vi "Text control 2 v7.2.vi"() -> ()   [LabVIEW 2019]
panel:
  in  "Tab Control":enum32{"Main", "Other parameters"}(tab)
  out "Vdg vs time (Bias Stress)":cluster{"Y data in":dbl[], "X data in":dbl[]}[](graph)
  out "Vp vs Vg (FPP)":cluster{"Y data in":dbl[], "X data in":dbl[]}[](graph)
  out "Vp2":dbl format="%.2e"
  out "Vp1":dbl format="%.2e"
  out "Vp vs time (FPP Bias Stress)":cluster{"Y data in":dbl[], "X data in":dbl[]}[](graph)
  in  "Plot sample extrema vs time":bool
  out "Line running":i32
  out "Total lines":i32
  out "Path":path=path "C:/users/rlp38/09Apr2009LTtesting/test2.txt"
  out "I vs Vg":cluster{"Y data in":dbl[], "X data in":dbl[]}[](graph)
  out "Is max":dbl format="%.2e"
  out "Id max":dbl format="%.2e"
  out "Ig max":dbl format="%.2e"
  out "Imax vs time":cluster{"Y data in":dbl[], "X data in":dbl[]}[](graph)
  out "Imin vs time":cluster{"Y data in":dbl[], "X data in":dbl[]}[](graph)
  out "I vs Vd":cluster{"Y data in":dbl[], "X data in":dbl[]}[](graph)
  in  "Script":string="#pulsedstressV d 0.03 20 0 0.5 0.0827 5\n#\n#itime m\n#gaterangemode a\n#drainrangemode a\n#pulsed on 0.05 0 0.02\n#transfer d -10 40 1 5 40 35\n#transfer d -10 40 1 5 40 35\n#transfer d -10 40 1 5 40 35\n#output d 0 40 20 0 40 1\n#\n#\n#sample 1 0.008 221 6 0.003\n#samplei 400e-6 200 6 0.002 0.1\n#vsu2pulse -10 4\n#\n#stressV 0.016 0.03 2e-4 0.1e-3 11\n#stressI 220e-7 0.08 15\n#transfer s -1 1 0.5 -0.005 0.005 0.005\n#output s 0 0 0 -0.008 0.008 0.002"
  out "Command running:":string
  out "Serial port data":string
  out "Elapsed Time":dbl caption="Elapsed Time (s)"
  in  "Time Units":u16(ring)=1 items=["Seconds", "Minutes", "Hours"]
  in  "Time Offset":dbl caption="Set Start Time (s)"
  in  "Reset":bool
  in  "Auto Reset":bool
  in  "integration time":u32(slide) max=2 step=1 scale=0.0..2.0
  out "Is on":dbl format="%.2e"
  out "Id on":dbl format="%.2e"
  out "Ig on":dbl format="%.2e"
  out "Ion vs time":cluster{"Y data in":dbl[], "X data in":dbl[]}[](graph)
  out "Ioff vs time":cluster{"Y data in":dbl[], "X data in":dbl[]}[](graph)
  out "Ig min":dbl format="%.2e"
  out "Id min":dbl format="%.2e"
  out "Is min":dbl format="%.2e"
  out "Is off":dbl format="%.2e"
  out "Id off":dbl format="%.2e"
  out "Ig off":dbl format="%.2e"
  in  "Integration time (long)":dbl=0.32 min=0.04 max=2.0 step=0.02 format="%.2f"
  in  "Integration time (short)":dbl=0.0019 min=8e-05 max=0.0019 step=8e-05 format="%^.0e"
  in  "Drain: Compliance":dbl=0.001 format="%.8f"
  in  "Gate: Compliance":dbl=0.001 format="%.8f"
  in  "Interrupt scan":bool
  in  "Interrupt program":bool
  in  "Plot output curve extrema vs time":bool
  in  "Plot transfer curve extrema vs time":bool
  out "I vs time (Bias Stress)":cluster{"Y data in":dbl[], "X data in":dbl[]}[](graph)
  in  "Sample I - Probe 4 (Disabled)":u32(ring)=3 items=["SMU1  ", "SMU2  ", "SMU3  ", "SMU4  ", "SMU5  ", "SMU6  ", "VSU1  ", "VSU2  "]
  in  "Sample I - Source/Common":u32(ring) items=["SMU1  ", "SMU2  ", "SMU3  ", "SMU4  ", "SMU5  ", "SMU6  ", "VSU1  ", "VSU2  "]
  in  "Sample I - Probe 3 (Disabled)":u32(ring)=2 items=["SMU1  ", "SMU2  ", "SMU3  ", "SMU4  ", "SMU5  ", "SMU6  ", "VSU1  ", "VSU2  "]
  in  "Sample I - Drain/Gate":u32(ring)=1 items=["SMU1  ", "SMU2  ", "SMU3  ", "SMU4  ", "SMU5  ", "SMU6  ", "VSU1  ", "VSU2  "]
  in  "Sample - Probe 4":u32(ring)=3 items=["SMU1  ", "SMU2  ", "SMU3  ", "SMU4  ", "SMU5  ", "SMU6  ", "VSU1  ", "VSU2  "]
  in  "Sample - Source/Common":u32(ring) items=["SMU1  ", "SMU2  ", "SMU3  ", "SMU4  ", "SMU5  ", "SMU6  ", "VSU1  ", "VSU2  "]
  in  "Sample - Gate":u32(ring)=2 items=["SMU1  ", "SMU2  ", "SMU3  ", "SMU4  ", "SMU5  ", "SMU6  ", "VSU1  ", "VSU2  "]
  in  "Sample - Drain":u32(ring)=1 items=["SMU1  ", "SMU2  ", "SMU3  ", "SMU4  ", "SMU5  ", "SMU6  ", "VSU1  ", "VSU2  "]
  in  "Gate Range\nmode":u16(ring) items=["Auto", "Limited", "Fixed"]
  in  "Gate Range":u8(slide)=3 max=11 scale=0.0..11.0
  in  "Source/Drain\nRange mode":u16(ring) items=["Auto", "Limited", "Fixed"]
  in  "Source/Drain Range":u8(slide)=3 max=11 scale=0.0..11.0
  in  "Panel Controls":T1={"Emergency Stop"=refnum, "TransGraph Max"=1e-05, "Text/Graph (text=false)"=TRUE} {"TransGraph Max" format="%.2e"}
  in  "Panel Controls 2":T2={"Emergency Stop"=refnum, "TransGraph Max"=1e-05, "Text/Graph (text=false)"=TRUE, "TransGraph Min"=1e-11} {"TransGraph Min" format="%.2e"; "TransGraph Max" format="%.2e"}
  out "error out":errorcluster
  in  "Delay before read (ms)":u32=1000
  in  "byte count":u32=64
  in  "Serial End Mode for Reads":u16(ring)=2 items=["None", "LastBit", "TermChar"]
  in  "Timeout (ms)":u32=10000
  in  "Enable Termination\nChar (T)":bool=TRUE
  in  "Termination char\n(0xA = '\\n' = LF)\n(0xD = '\\r' = CR)":u8=13 format="%.0x"
  in  "flow control":u16(ring) items=["None"=0, "XON/XOFF"=1, "RTS/CTS"=2, "DTR/DSR"=4]
  in  "stop bits":u16(ring)=10 items=["1.0"=10, "1.5"=15, "2.0"=20]
  in  "parity":u16(ring) items=["None", "Odd", "Even", "Mark", "Space"]
  in  "data bits":u16=8 min=5 max=8 step=1
  in  "VISA resource name":refnum<visa-resource-name>="COM6"
  in  "baud rate":u32=9600
  out "Timings Indicator":T3
  in  "Timings (overwritten by the Front Panel)":T4={"integration time"=0, "Short/Long integration time"=0.00064, "hold time (sec)"=0.0, "delay time (sec)"=0.0, "Step Time (0 disables)"=0.0, "sweep method"=0, "Pulse period"=0.005, "Base voltage"=0.0, "Pulse width"=0.0005} {"Pulse width" min=0.0005 max=0.1 step=0.0001 format="%.4f"; "Base voltage" format="%^.4e"; "Pulse period" min=0.005 max=1.0 step=0.0001 format="%.4f"; "sweep method" items=["Continuous", "Pulsed"]; "Step Time (0 disables)" format="%.2f"; "delay time (sec)" format="%.4f"; "hold time (sec)" format="%.4f"; "Short/Long integration time" format="%^.0e"; "integration time" scale=0.0..2.0}
  in  "Probe 4":cluster{"on/off":bool, "Voltage":dbl} {"Voltage" min=-100.0 max=100.0 format="%.2f"}
  in  "Full Reset":bool
  in  "Standby":T5
  out "Probe 4 Indicator":cluster{"on/off":bool, "Voltage":dbl} {"Voltage" min=-100.0 max=100.0 format="%.2f"}
  in  "Transfer/Output - Drain":u32(ring)=1 items=["SMU1  ", "SMU2  ", "SMU3  ", "SMU4  ", "SMU5  ", "SMU6  ", "VSU1  ", "VSU2  "]
  in  "Transfer/Output - Gate":u32(ring)=2 items=["SMU1  ", "SMU2  ", "SMU3  ", "SMU4  ", "SMU5  ", "SMU6  ", "VSU1  ", "VSU2  "]
  in  "Transfer/Output - Source/Common":u32(ring) items=["SMU1  ", "SMU2  ", "SMU3  ", "SMU4  ", "SMU5  ", "SMU6  ", "VSU1  ", "VSU2  "]
  in  "Transfer/Output - Probe 4":u32(ring)=3 items=["SMU1  ", "SMU2  ", "SMU3  ", "SMU4  ", "SMU5  ", "SMU6  ", "VSU1  ", "VSU2  "]
  in  "Pulsed Stress V - Probe 4":u32(ring)=3 items=["SMU1  ", "SMU2  ", "SMU3  ", "SMU4  ", "SMU5  ", "SMU6  ", "VSU1  ", "VSU2  "]
  in  "Pulsed Stress V - Vextra":u32(ring)=6 items=["SMU1  ", "SMU2  ", "SMU3  ", "SMU4  ", "SMU5  ", "SMU6  ", "VSU1  ", "VSU2  "]
  in  "Pulsed Stress V - Drain":u32(ring)=1 items=["SMU1  ", "SMU2  ", "SMU3  ", "SMU4  ", "SMU5  ", "SMU6  ", "VSU1  ", "VSU2  "]
  in  "Pulsed Stress V - Source/Common":u32(ring) items=["SMU1  ", "SMU2  ", "SMU3  ", "SMU4  ", "SMU5  ", "SMU6  ", "VSU1  ", "VSU2  "]
  in  "Pulsed Stress V - Gate":u32(ring)=2 items=["SMU1  ", "SMU2  ", "SMU3  ", "SMU4  ", "SMU5  ", "SMU6  ", "VSU1  ", "VSU2  "]
  in  "FPP - Drain":u32(ring)=1 items=["SMU1  ", "SMU2  ", "SMU3  ", "SMU4  ", "SMU5  ", "SMU6  ", "VSU1  ", "VSU2  "]
  in  "FPP - Gate":u32(ring)=2 items=["SMU1  ", "SMU2  ", "SMU3  ", "SMU4  ", "SMU5  ", "SMU6  ", "VSU1  ", "VSU2  "]
  in  "FPP - Probe 1":u32(ring) items=["SMU1  ", "SMU2  ", "SMU3  ", "SMU4  ", "SMU5  ", "SMU6  ", "VSU1  ", "VSU2  "]
  in  "FPP - Probe 2":u32(ring)=3 items=["SMU1  ", "SMU2  ", "SMU3  ", "SMU4  ", "SMU5  ", "SMU6  ", "VSU1  ", "VSU2  "]
  in  "FPP - Source":u32(ring)=6 items=["SMU1  ", "SMU2  ", "SMU3  ", "SMU4  ", "SMU5  ", "SMU6  ", "VSU1  ", "VSU2  "]
  in  "Stress V - Drain":u32(ring)=1 items=["SMU1  ", "SMU2  ", "SMU3  ", "SMU4  ", "SMU5  ", "SMU6  ", "VSU1  ", "VSU2  "]
  in  "Stress V - Gate":u32(ring)=2 items=["SMU1  ", "SMU2  ", "SMU3  ", "SMU4  ", "SMU5  ", "SMU6  ", "VSU1  ", "VSU2  "]
  in  "Stress V - Source/Common":u32(ring) items=["SMU1  ", "SMU2  ", "SMU3  ", "SMU4  ", "SMU5  ", "SMU6  ", "VSU1  ", "VSU2  "]
  in  "Stress I - Drain/Gate":u32(ring)=1 items=["SMU1  ", "SMU2  ", "SMU3  ", "SMU4  ", "SMU5  ", "SMU6  ", "VSU1  ", "VSU2  "]
  in  "Stress I - Source/Common":u32(ring) items=["SMU1  ", "SMU2  ", "SMU3  ", "SMU4  ", "SMU5  ", "SMU6  ", "VSU1  ", "VSU2  "]
  in  "VSU2 Stress - Source/Common":u32(ring) items=["SMU1  ", "SMU2  ", "SMU3  ", "SMU4  ", "SMU5  ", "SMU6  ", "VSU1  "]
  in  "VISA resource name in":refnum<visa-resource-name>="GPIB0::14::INSTR"
  in  "Gate":T6={"Gate Start"=0.0, "Gate Stop"=2.0, "Gate Step (linear only)"=1.0, "Gate Compliance"=0.0001, "Gate PComp"=0.0, "Range mode"=0, "Range"=6} {"Range" max=11 scale=0.0..11.0; "Range mode" items=["Auto", "Limited", "Fixed"]; "Gate PComp" format="%^.2e"; "Gate Compliance" format="%^.2e"; "Gate Step (linear only)" format="%^.4e"; "Gate Stop" format="%^.4e"; "Gate Start" format="%^.4e"}
  in  "Drain 2":T7={"Drain Start"=0.0, "Drain Stop"=2.0, "Drain Compliance"=0.0001, "Drain Step"=1.0, "Drain PComp"=0.0, "Range mode"=0, "Range"=6} {"Range" max=11 scale=0.0..11.0; "Range mode" items=["Auto", "Limited", "Fixed"]; "Drain PComp" format="%^.2e"; "Drain Step" format="%^.4e"; "Drain Compliance" format="%^.2e"; "Drain Stop" format="%^.4e"; "Drain Start" format="%^.4e"}
  # "Time"
  # "Syntax:\nitime [s|m|l] time(sec): [s|m|l] determines the integration time setting (small|medium|long) and time sets the value.\nNOTE: The value of the integration time has to be within the range allowed by its category (s|m|l), otherwise, the closest value will be used. (e.g. if the category is set to short but the time value is very long, the actual value used will be the maximum short integration time.\nIntegration times:\n    Short: Default: 640 us. Range: 8E-5 - 1.92E-3 seconds.\n    Medium: Fixed at 1 NPL cycle (0.02 seconds).\n    Long: Default: 16 NPL cycles (0.32 seconds). Range: 2-100 NPL cycles (0.04 seconds - 2 seconds).\ngaterangemode [a|l|f]\ndrainrangemode [a|l|f]\npulsed [on|off] PulsePeriod(sec) PulseBaseVoltage PulseONWidth(sec)\nstandby [on l off]\nwait NumMilliseconds\nwait-min NumMinutes\n# texthere = comment\nProbe4 [ON|OFF] Voltage\ntransfer [s|d] VgStart VgStop VgStep VdStart VdStop VdStep\noutput [s|d] VgStart VgStop VgStep VdStart VdStop VdStep\nsample Vg Vd NumSamples Time(s) SampleInterval(s)\nsamplei Idg NumSamples Time(s) SampleInterval(s) VDGcompliance\n100 samples is approximately 13 seconds with medium integration\n# if in doubt use SampleInterval(s) = 0.004\n    NOTE: When doing bias stress measurements, it is best to set the Time Units to \"Seconds\", as the \"sample\" command has been configured to give the output to seconds.\nstressV VG VD IGcompliance IDcompliance Duration(sec)\nstressI IDG VDGcompliance Duration(sec)\nvsu2pulse Bias Duration(s)\npulsedstressV [s|d] VEstop VgON VgOFF Period(s) PulseONwidth(s) Vd\nsample-fpp Vg Vd NumSamples Time\nresample-fpp Vg Vd\ntransfer-fpp [s|d] VgStart VgStop VgStep VdStart VdStop VdStep\noutput-fpp [s|d] VgStart VgStop VgStep VdStart VdStop VdStep\nserial SerialPortCommand"
  # "1\n2\n3\n4\n5\n6\n7\n8\n9\n10\n11\n12\n13\n14\n15\n16\n17\n18\n19\n20"
  # "SMUs"
  # "Serial port settings"
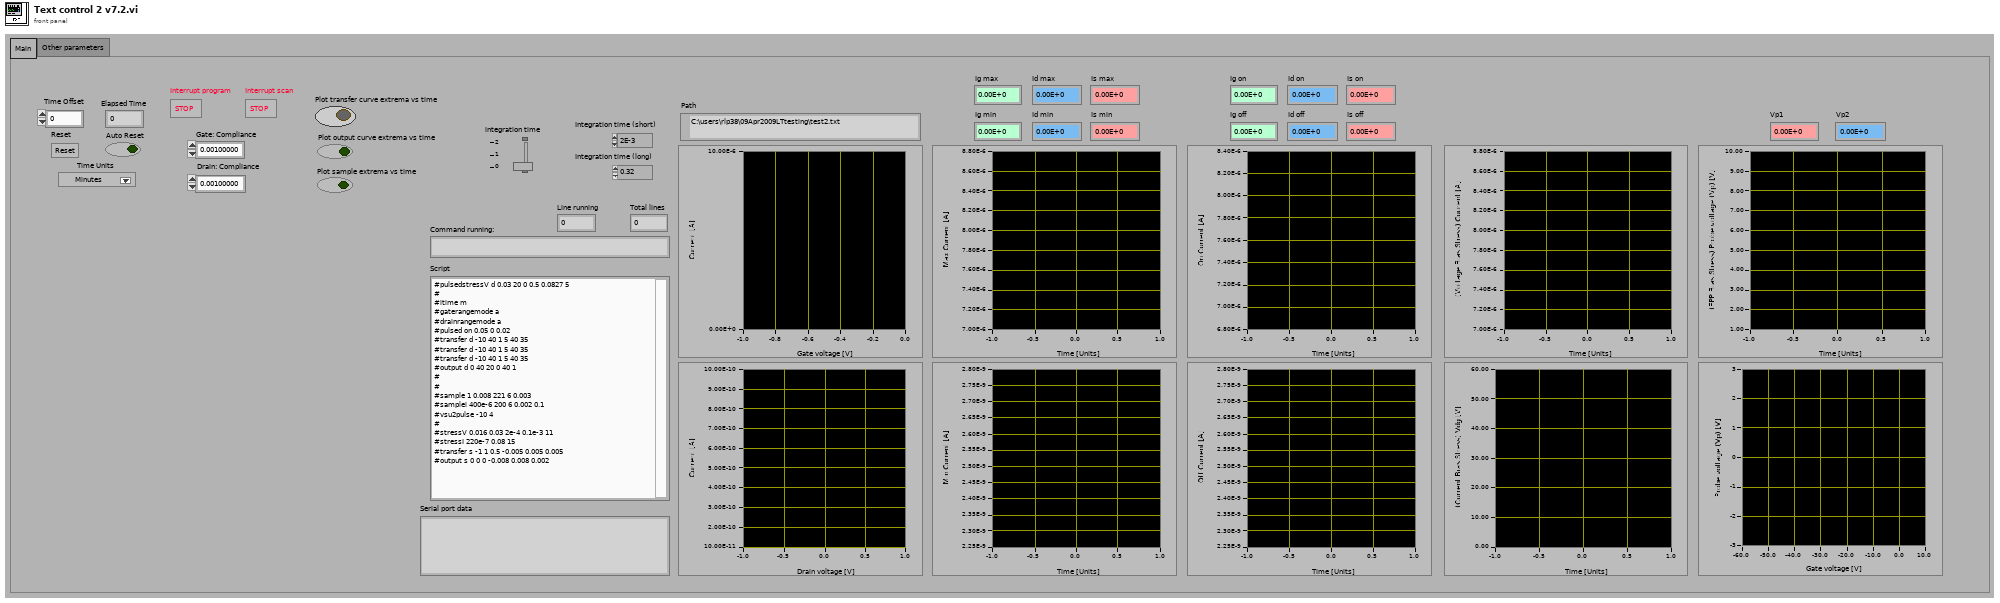
[diagram p1: front panel]
types:
  T1 = cluster{"Emergency Stop":refnum<vi>, "TransGraph Max":dbl, "Text/Graph (text=false)":bool}
  T2 = cluster{"Emergency Stop":refnum<vi>, "TransGraph Max":dbl, "Text/Graph (text=false)":bool, "TransGraph Min":dbl}
  T3 = cluster{"integration time (0:s, 1:m, 2:l)":u32, "Short/Long integration time":dbl, "hold time (sec)":dbl, "delay time (sec)":dbl, "Step Time (0 disables)":dbl, "sweep method":u16, "Pulse period":dbl, "Base voltage":dbl, "Pulse width":dbl}
  T4 = cluster{"integration time":u32, "Short/Long integration time":dbl, "hold time (sec)":dbl, "delay time (sec)":dbl, "Step Time (0 disables)":dbl, "sweep method":u16, "Pulse period":dbl, "Base voltage":dbl, "Pulse width":dbl}
  T5 = cluster{"Gate Standby":bool, "Drain Standby":bool}
  T6 = cluster{"Gate Start":dbl, "Gate Stop":dbl, "Gate Step (linear only)":dbl, "Gate Compliance":dbl, "Gate PComp":dbl, "Range mode":u16, "Range":u8}
  T7 = cluster{"Drain Start":dbl, "Drain Stop":dbl, "Drain Compliance":dbl, "Drain Step":dbl, "Drain PComp":dbl, "Range mode":u16, "Range":u8}
  T8 = enum16{"open", "replace", "create", "open or create", "replace or create", "replace or create with confirmation"}
  T9 = cluster{"V2 Start":dbl, "V2 Step":dbl, "Number of points":i32}
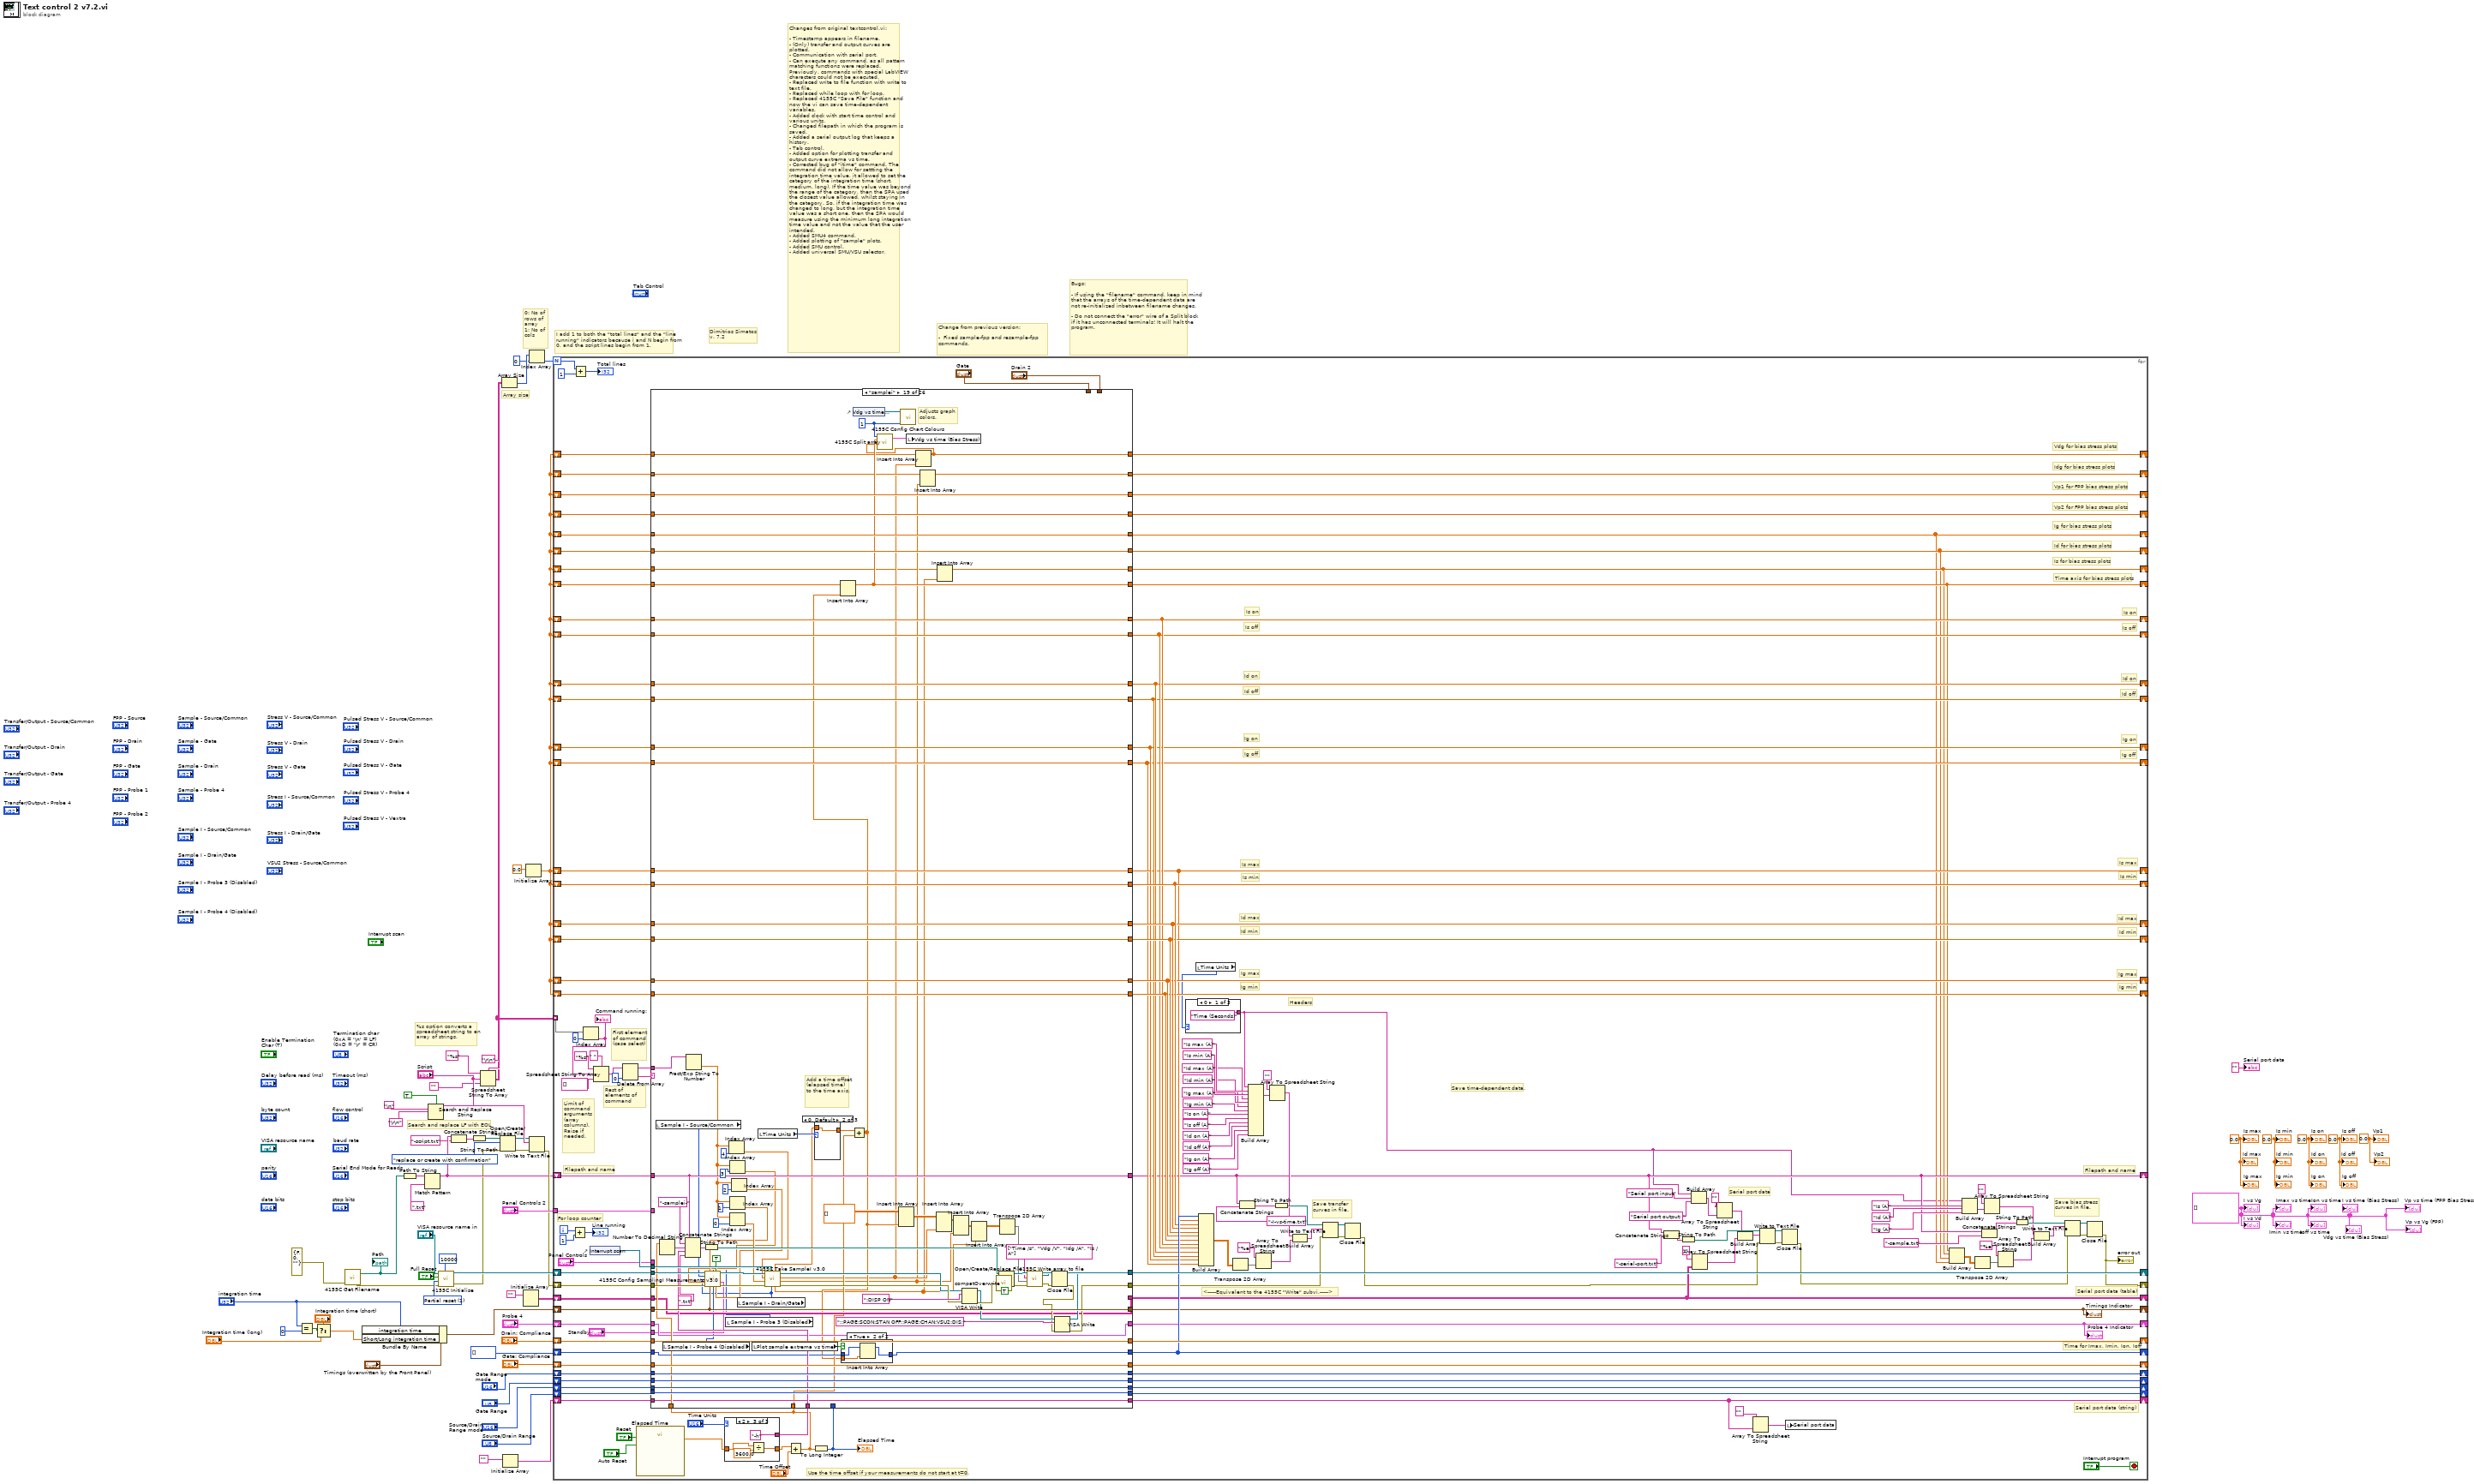
[diagram p0: block diagram]
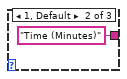
[diagram p2: hidden frame]
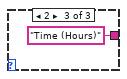
[diagram p3: hidden frame]
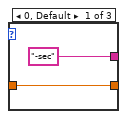
[diagram p4: hidden frame]
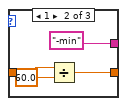
[diagram p5: hidden frame]
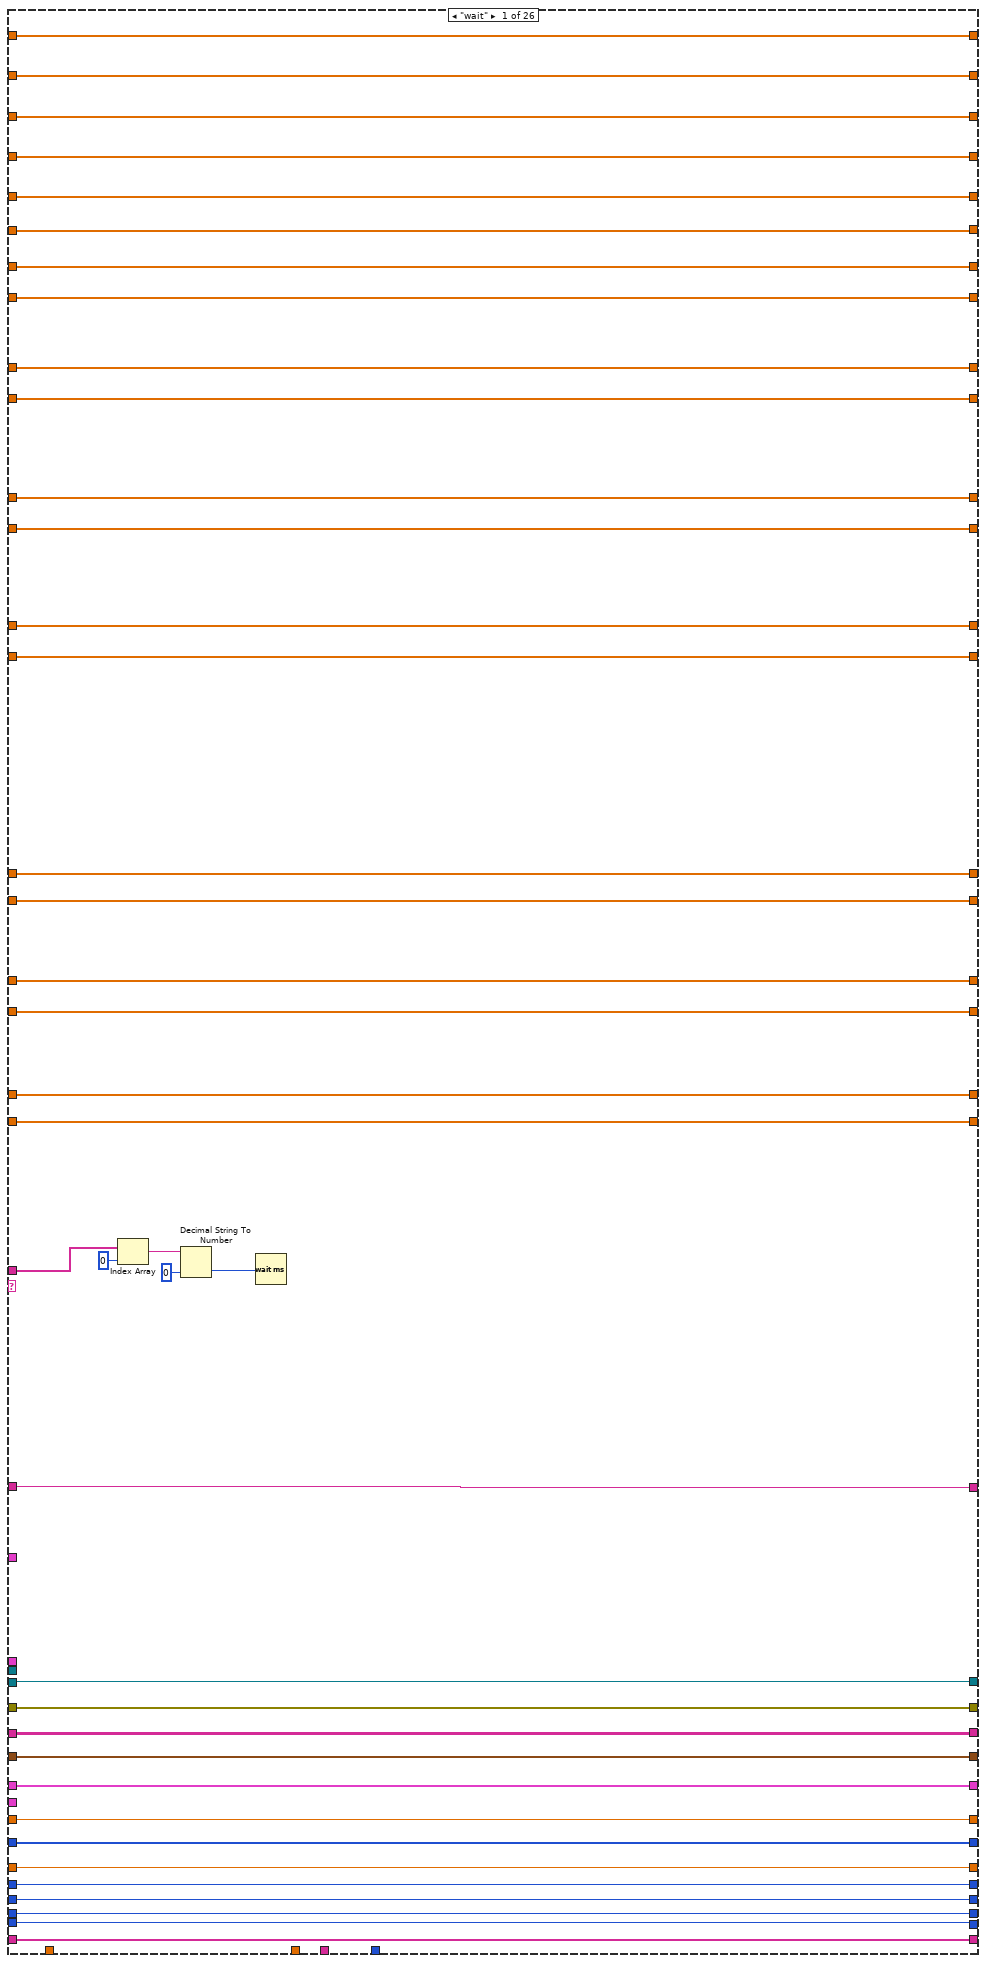
[diagram p6: hidden frame]
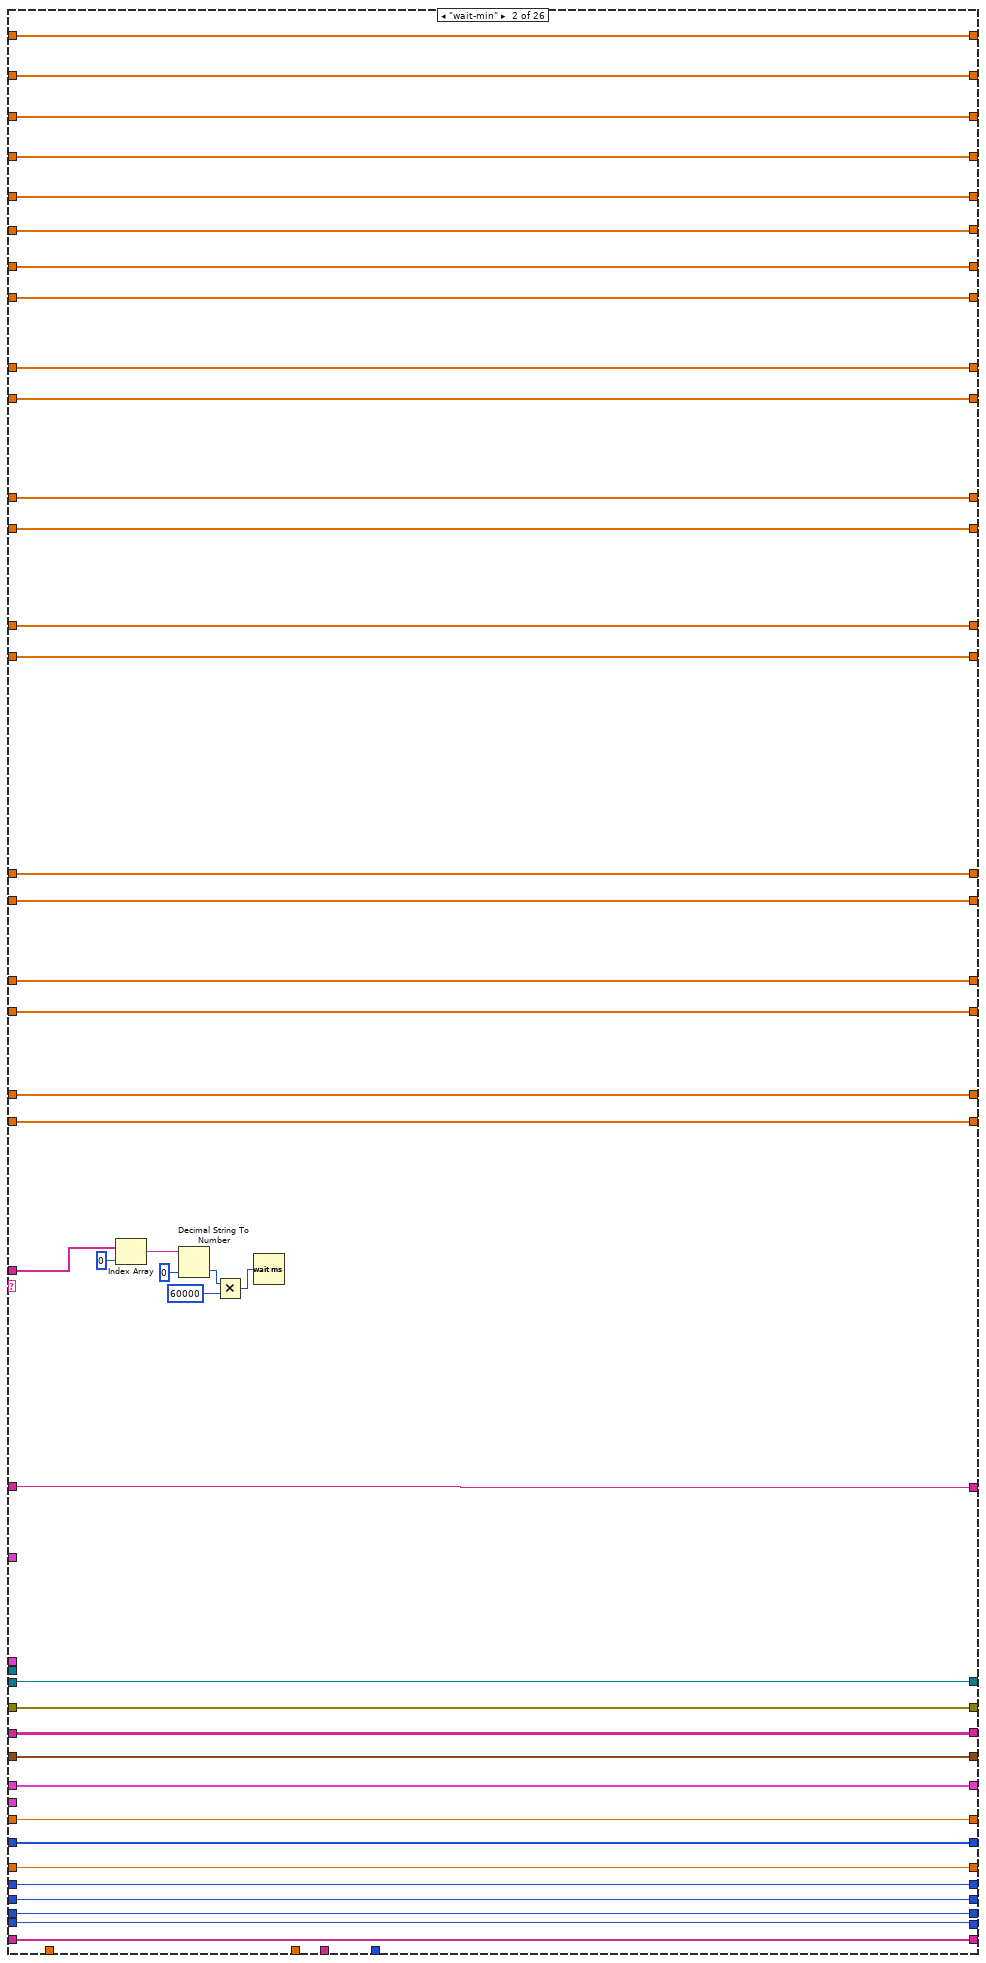
[diagram p7: hidden frame]
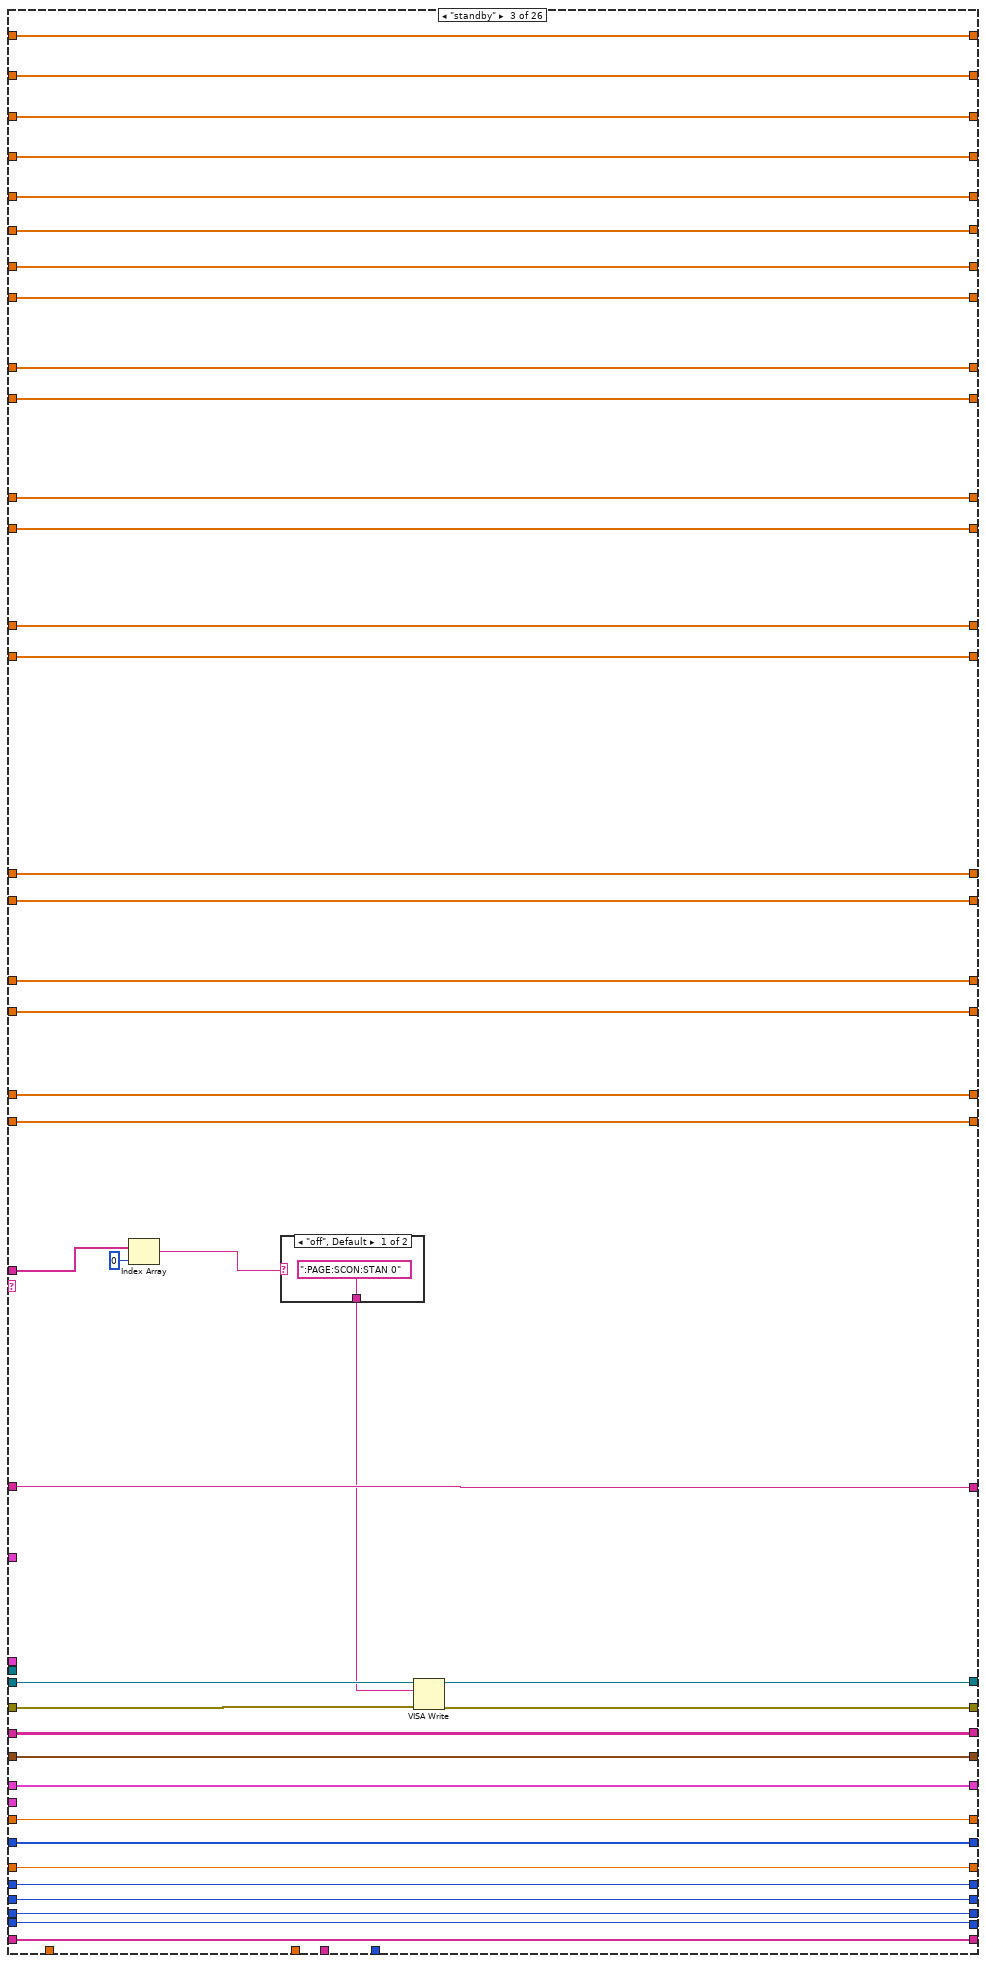
[diagram p8: hidden frame]
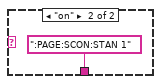
[diagram p9: hidden frame]
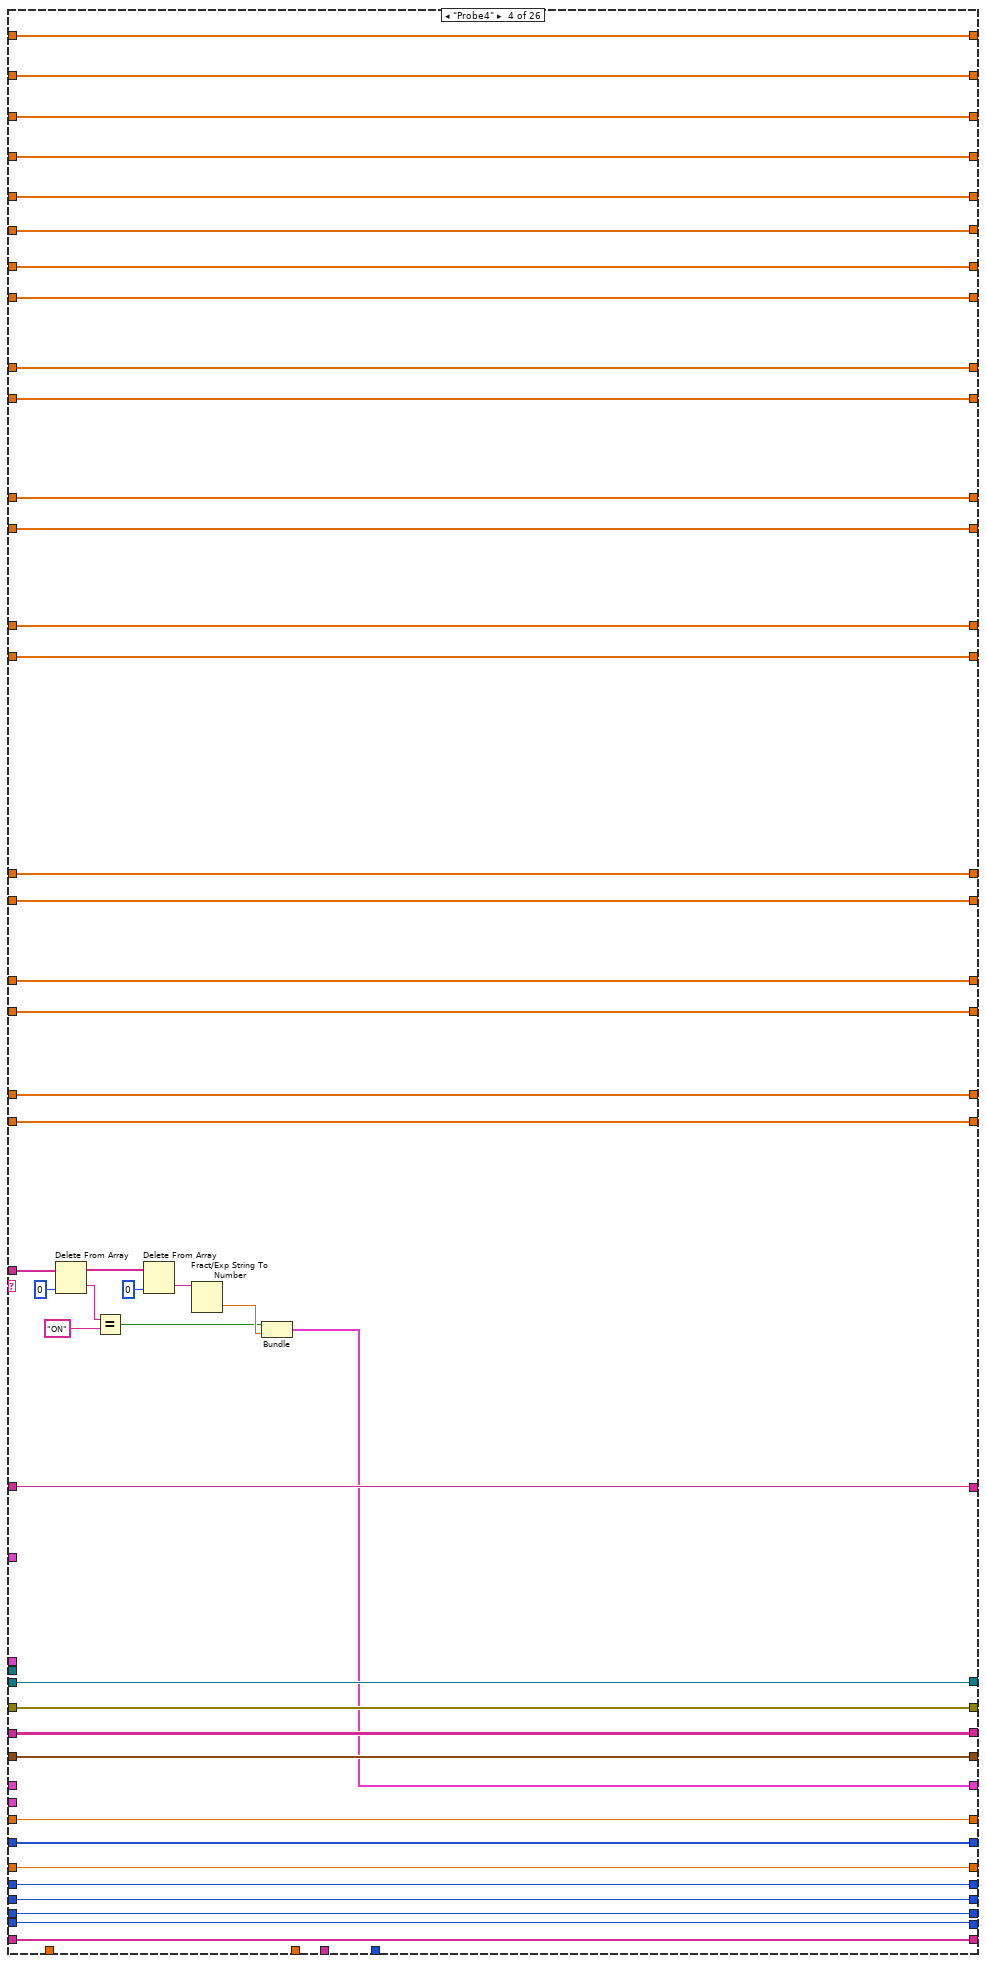
[diagram p10: hidden frame]
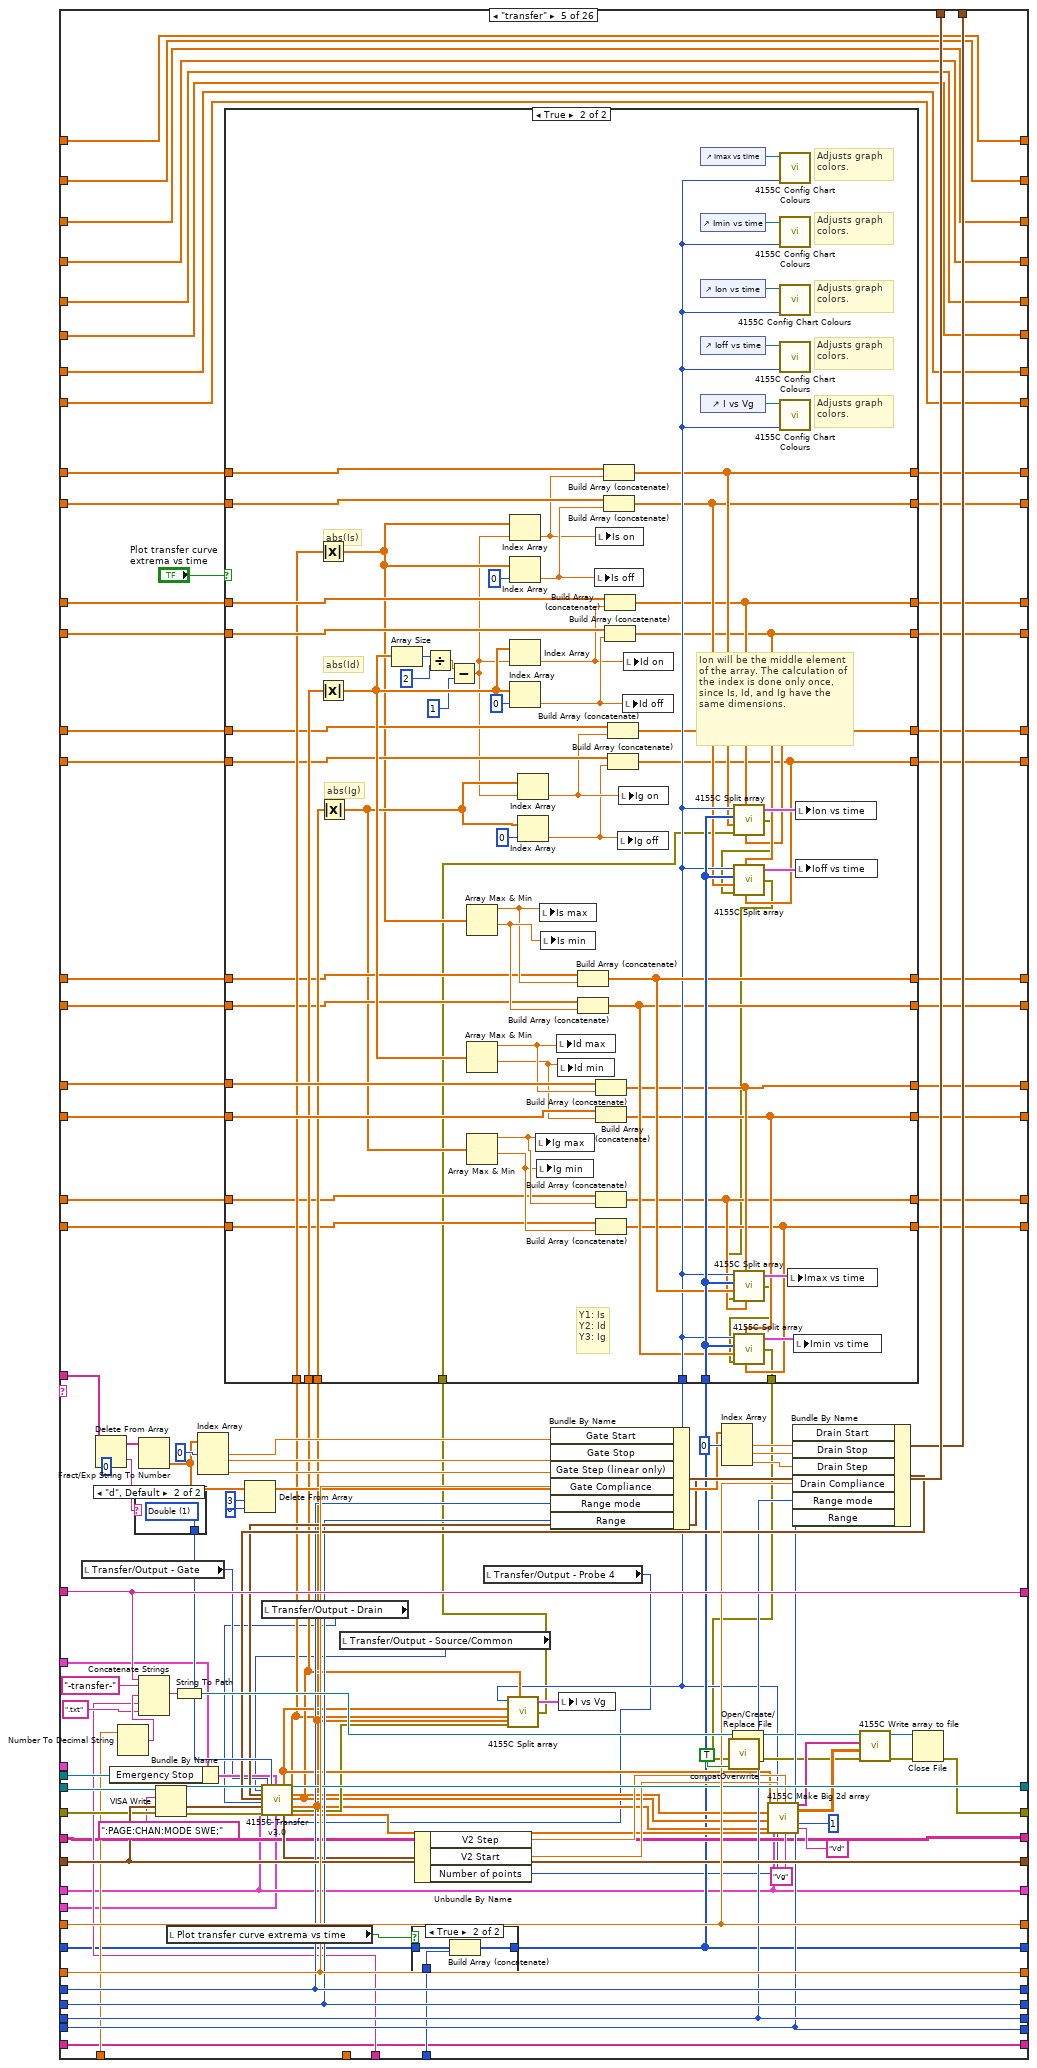
[diagram p11: hidden frame]
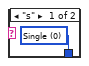
[diagram p14: hidden frame]
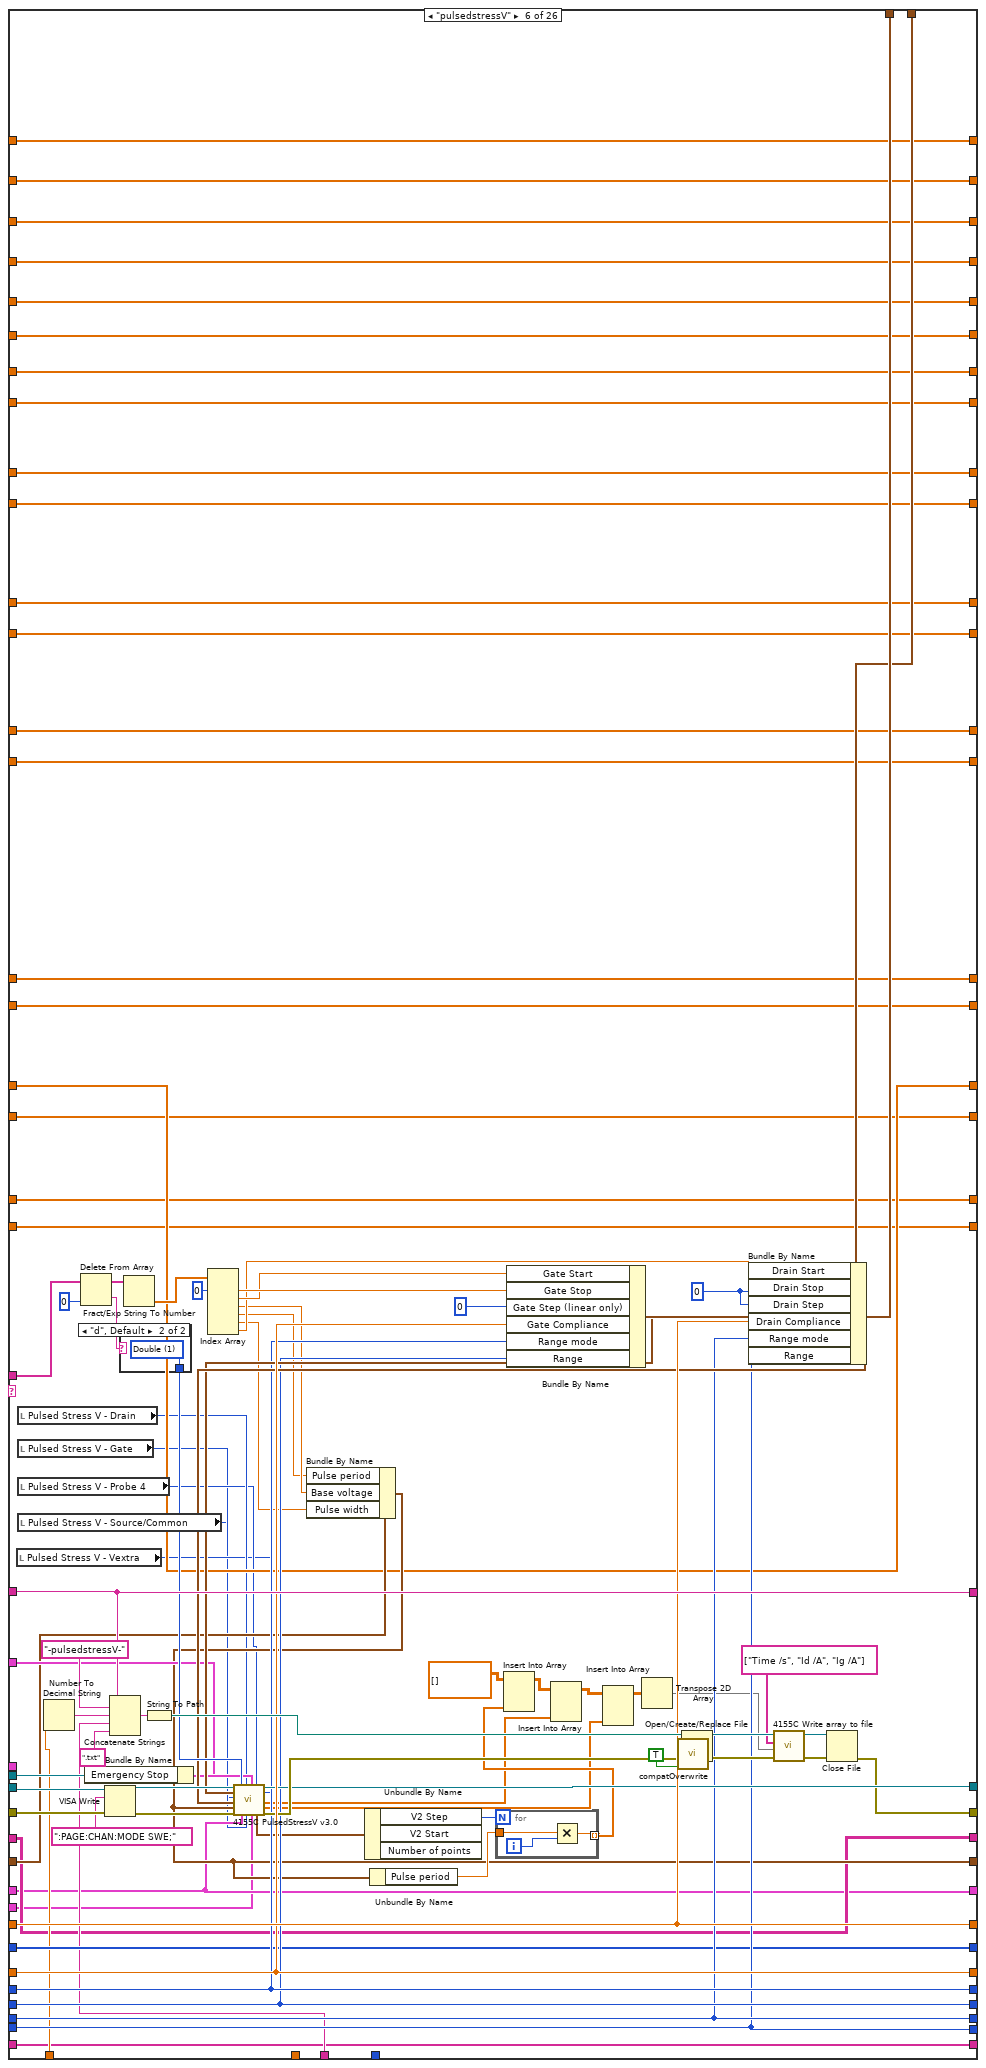
[diagram p15: hidden frame]
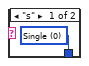
[diagram p16: hidden frame]
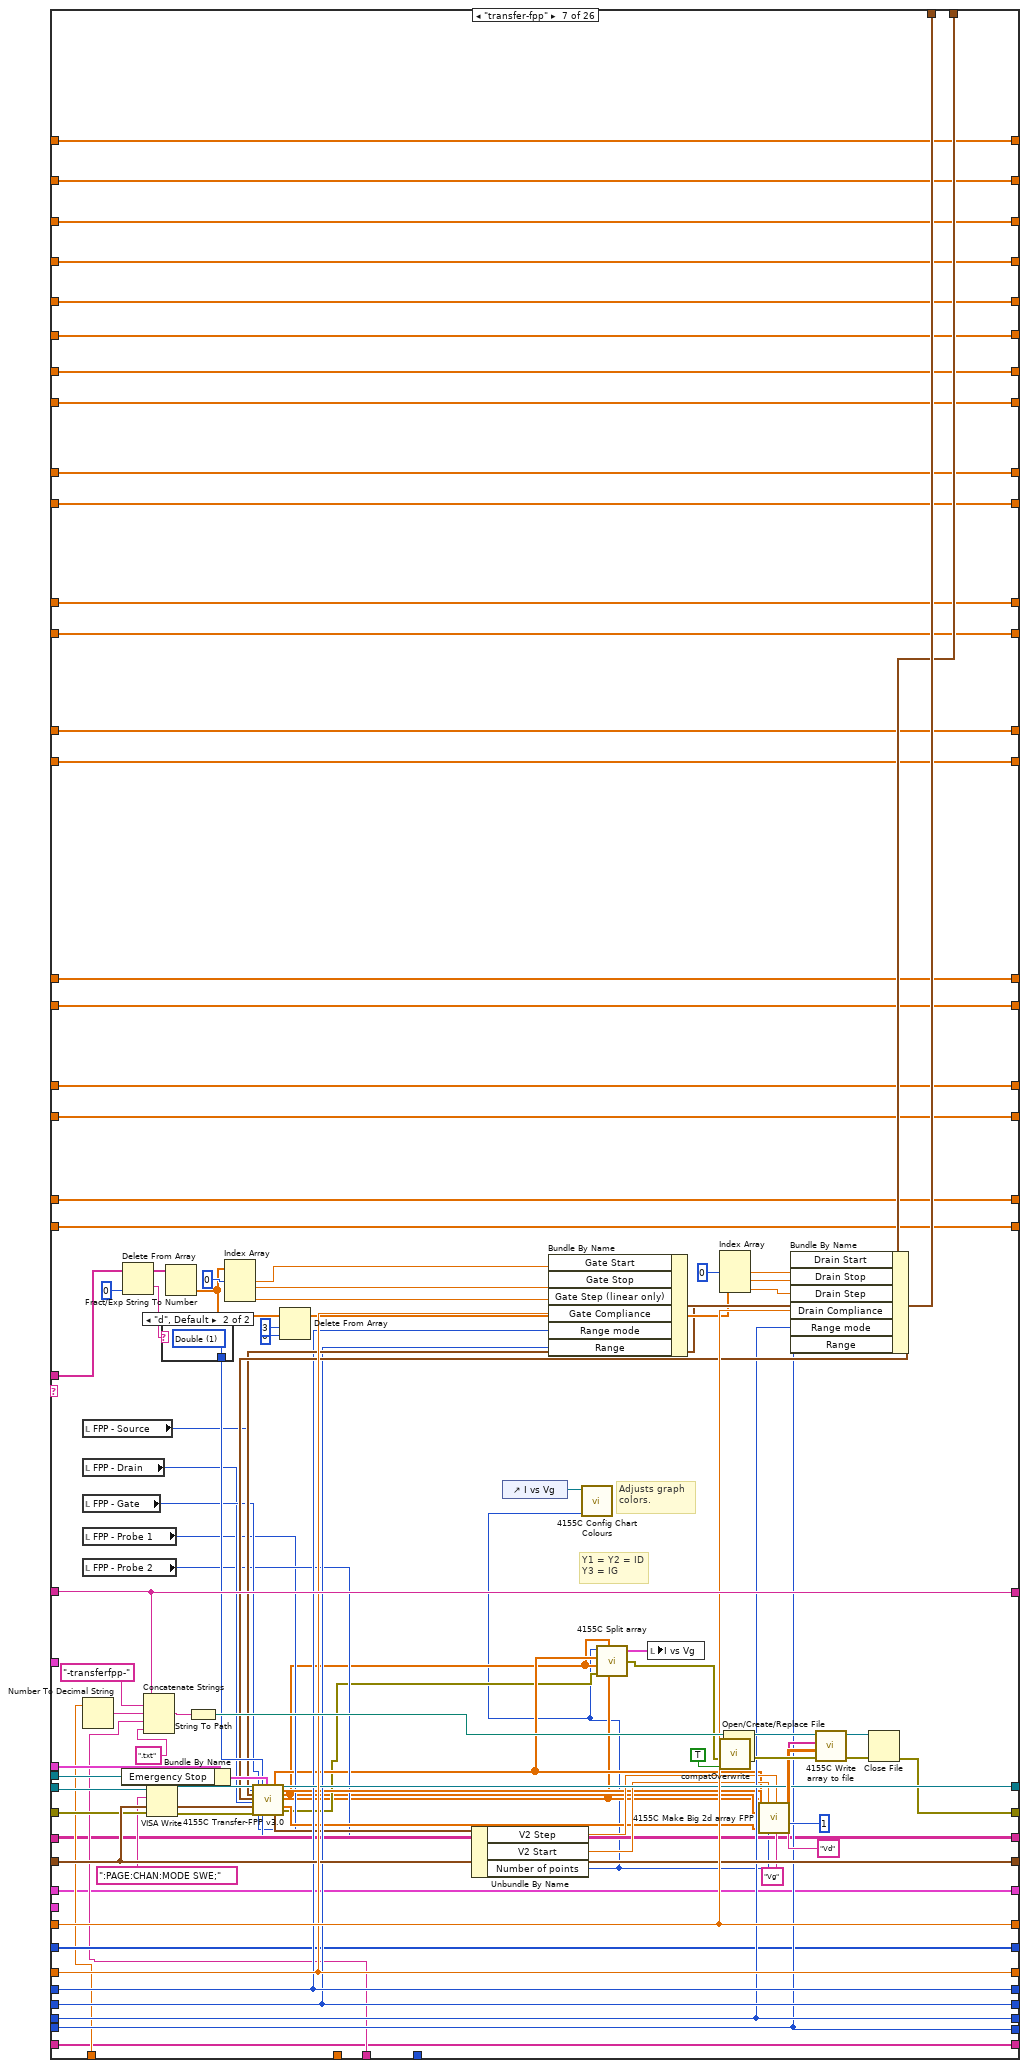
[diagram p17: hidden frame]
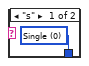
[diagram p18: hidden frame]
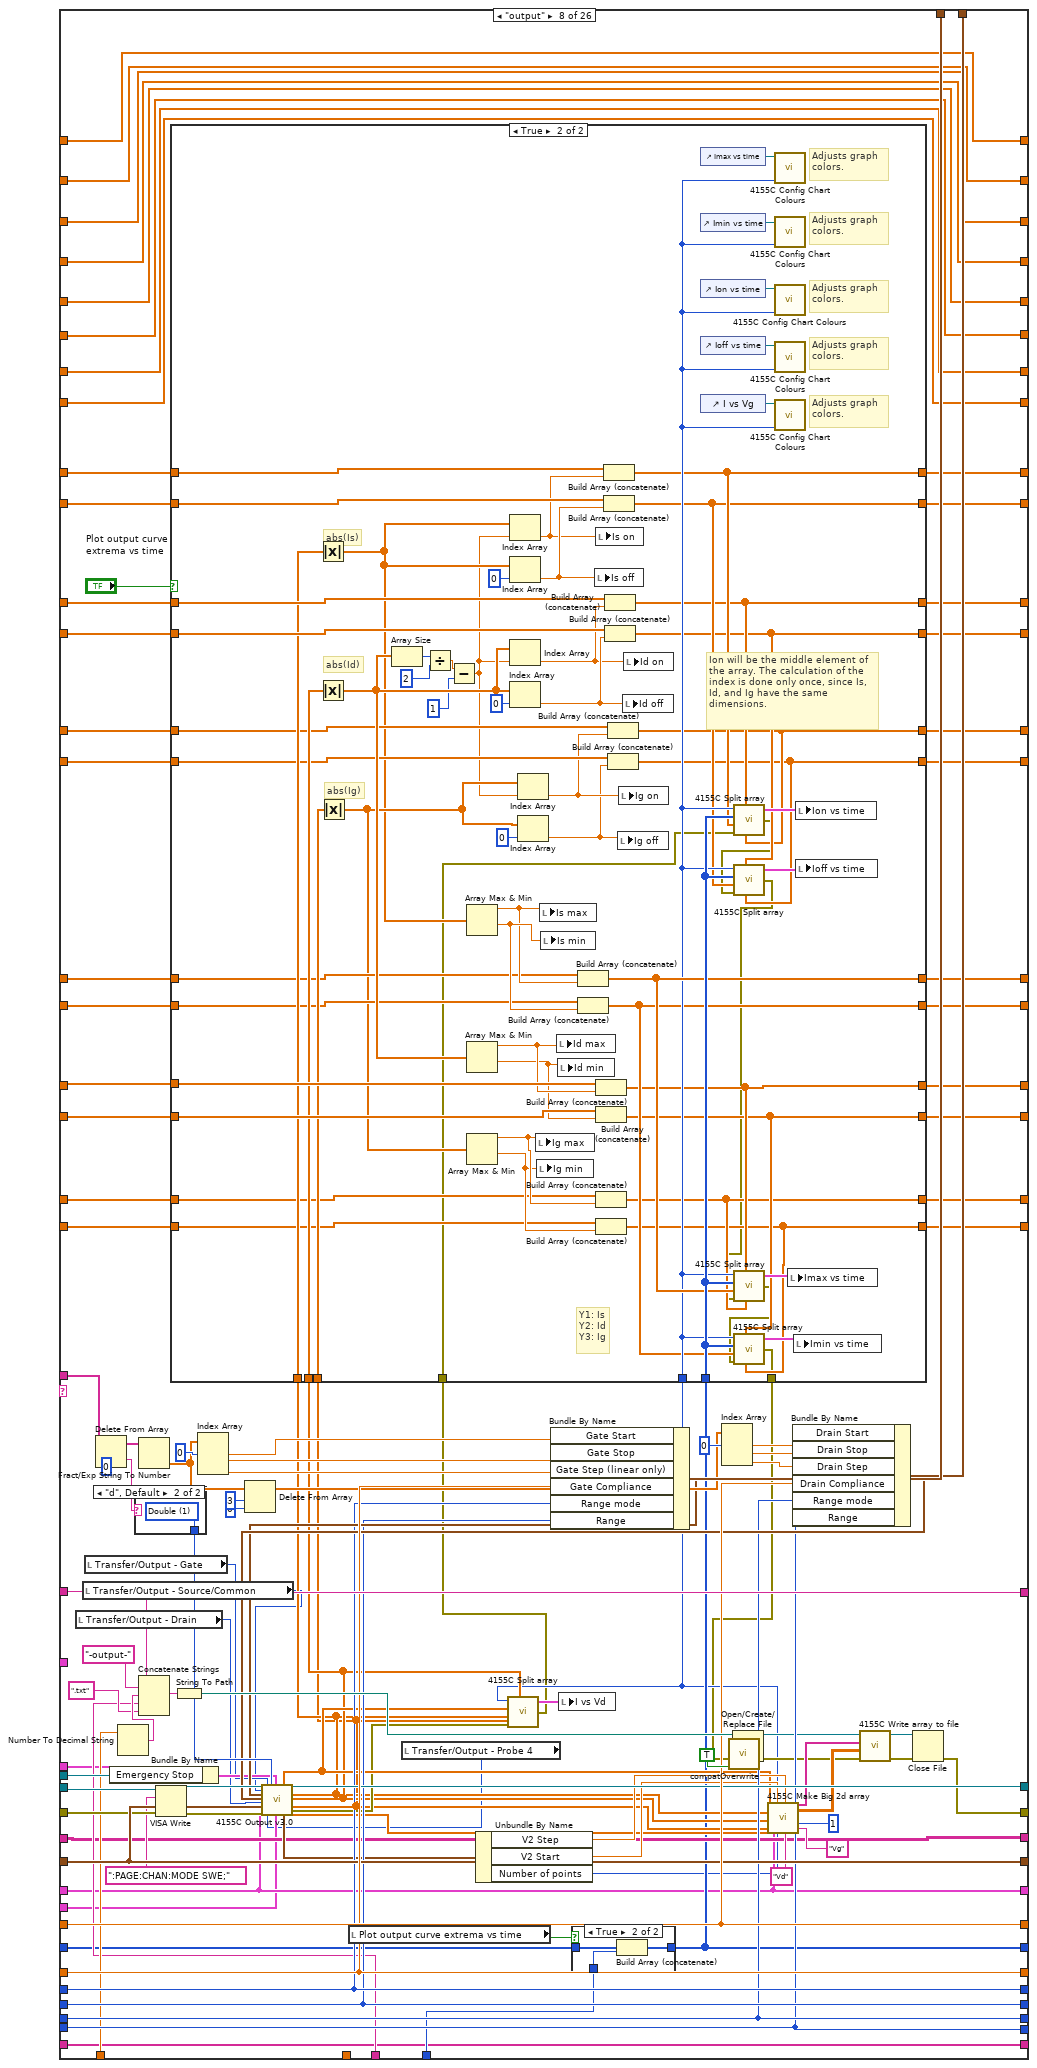
[diagram p19: hidden frame]
diagram:
  w3 = 0.0 ("Is off")
  w2 = cluster{"Y data in":dbl[], "X data in":dbl[]}[] [] ("I vs Vg")
  w10 = 0.0 ("Is off")
  w11 = 0.0 ("Is on")
  w12 = 0.0 ("Is min")
  w13 = 0.0 ("Is max")
  w56 = u16 1 items=["Reset All", "Partial reset"] ("Type of reset")
  # "Change from previous version:\n\n-  Fixed sample-fpp and resample-fpp commands."
  # "I add 1 to both the \"total lines\" and the \"line running\" indicators because i and N begin from 0, and the script lines begin from 1."
  # "Bugs:\n\n- If using the \"filename\" command, keep in mind that the arrays of the time-dependent data are not re-initialized inbetween filename changes. \n\n- Do not connect the \"error\" wire of a Split block if it has unconnected terminals! It will halt the program."
  # "Array size"
  # "%s option converts a spreadsheet string to an array of strings."
  # "0: No of rows of array\n1: No of cols"
  # "Dimitrios Simatos\nv. 7.2"
  # "Changes from original textcontrol.vi:\n\n- Timestamp appears in filename.\n- (Only) transfer and output curves are plotted.\n- Communication with serial port.\n- Can execute any command, as all pattern matching functions were replaced. Previously, commands with special LabVIEW characters could not be executed.\n- Replaced write to file function with write to text file.\n- Replaced while loop with for loop.\n- Replaced 4155C \"Save File\" function and now the vi can save time-dependent variables.\n- Added clock with start time control and various units.\n- Changed filepath in which the program is saved.\n- Added a serial output log that keeps a history.\n- Tab control.\n- Added option for plotting transfer and output curve extrema vs time.\n- Corrected bug of \"itime\" command. The command did not allow for settting the integration time value, it allowed to set the category of the integration time (short, medium, long). If the time value was beyond the range of the category, then the SPA used the closest value allowed, whilst staying in the category. So, if the integration time was changed to long, but the integration time value was a short one, then the SPA would measure using the minimum long integration time value and not the value that the user intended.\n- Added SMU4 command.\n- Added plotting of \"sample\" plots.\n- Added SMU control.\n- Added universal SMU/VSU selector."
  # "Search and replace LF with EOL"
  n1 = Equal?(x="integration time", y=u32 0) -> (x = y?=w57:bool)
  n2 = Select(t="Integration time (short)", s=w57, f="Integration time (long)") -> (s? t:f=w18:dbl)
  n3 = call "4155C Get Filename.vi"("error in (no error)"=errorcluster {"status"=FALSE, "code"=0, "source"=""}) -> ("error out"=w51:errorcluster, "path"=w26:path)  [unwired: 2 in, 1 out]
  "Path" <- w26
  n4 = Bundle By Name(cluster="Timings (overwritten by the Front Panel)", "integration time"="integration time", "Short/Long integration time"=w18) -> (w49:T4)
  n5 = Path To String(path=w26) -> (string=w27:string)
  n6 = Match Pattern(string=w27, regular expression=".txt") -> (before substring=w16:string)  [unwired: 1 in, 3 out]
  n7 = Search and Replace String(replace all?=TRUE ("replace all? (F)"), input string="Script", search string="\n", replace string="\r\n") -> (result string=w39:string)  [unwired: 4 in, 3 out]
  n8 = call "4155C Initialise.vi"("VISA resource name in"="VISA resource name in", "Reset"="Full Reset", "Type of reset"=w56, "error in (no error)"=w51, "VISA Timeout Value"=u32 10000) -> ("VISA Resource Name out"=w50:refnum<visa-resource-name>, "error out"=w8:errorcluster)
  n9 = Concatenate Strings(w16, "-script.txt" ("string")) -> (w17:string)
  n10 = String To Path(string=w17) -> (path=w6:path)
  n11 = Spreadsheet String To Array(delimiter (Tab)="\r\n", format string="%s", spreadsheet string="Script", array type (2D Dbl)="") -> (array=w30:string[][])
  n12 = Open/Create/Replace File(file path (use dialog)=w6, error in=w8, operation (0:open)=T8."replace or create with confirmation") -> (refnum out=w5:refnum<file>, error out=w7:errorcluster)  [unwired: 3 in, 1 out]
  n13 = Array Size(array=w30) -> (size(s)=w34:i32[])
  n14 = Initialize Array("") -> (w21:string[])  [unwired: 1 in]
  n15 = Initialize Array("") -> (w19:string[][])  [unwired: 2 in]
  n16 = Initialize Array(0.0 ("element")) -> (w1:dbl[])  [unwired: 1 in]
  n17 = Index Array(array=w34, index=0) -> (element=w32:i32)
  n18 = Write to Text File(file (use dialog)=w5, text=w39, error in=w7) -> (error out=w24:errorcluster)  [unwired: 1 in, 2 out]
  n19 = for {
    N: w32 -> [w166]
    shift-left: "Source/Drain Range" -> [w206]
    shift-right: [w202] -> _
    shift-left: "Source/Drain\nRange mode" -> [w207]
    shift-right: [w203] -> _
    shift-left: "Gate Range" -> [w208]
    shift-right: [w204] -> _
    shift-left: "Gate Range\nmode" -> [w209]
    shift-right: [w205] -> _
    shift-left: "Gate: Compliance" -> [w217]
    shift-right: [w214] -> _
    shift-left: "Drain: Compliance" -> [w218]
    shift-right: [w215] -> _
    shift-left: w49 -> [w219]
    shift-right: [w71] -> _
    shift-left: w24 -> [w220]
    shift-right: [w72] -> _
    shift-left: w50 -> [w221]
    shift-right: [w216] -> _
    shift-left: w16 -> [w222]
    shift-right: [w79] -> _
    tunnel: "Panel Controls 2" -> [w200]
    shift-right: [w119] -> _
    shift-left: w1 -> [w199]
    shift-right: [w153] -> _
    shift-left: i32[] [] -> [w195]
    tunnel: w30 -> [w194] mode=indexing
    shift-right: [w118] -> _
    shift-left: w1 -> [w171]
    shift-right: [w148] -> _
    shift-left: w21 -> [w158]
    shift-right: [w149] -> _
    shift-left: w19 -> [w151]
    shift-right: [w112] -> _
    shift-left: w1 -> [w140]
    shift-right: [w113] -> _
    shift-left: w1 -> [w139]
    shift-right: [w117] -> _
    shift-left: w1 -> [w128]
    shift-right: [w116] -> _
    shift-left: w1 -> [w127]
    shift-right: [w110] -> _
    shift-left: w1 -> [w126]
    shift-right: [w120] -> _
    shift-left: w1 -> [w125]
    shift-right: [w111] -> _
    shift-left: w1 -> [w124]
    shift-right: [w109] -> _
    shift-left: w1 -> [w123]
    shift-right: [w115] -> _
    shift-left: w1 -> [w122]
    shift-right: [w114] -> _
    shift-left: w1 -> [w121]
    shift-right: [w70] -> _
    shift-left: "Probe 4" -> [w201]
    shift-right: [w75] -> _
    shift-left: w1 -> [w100]
    shift-right: [w76] -> _
    shift-left: w1 -> [w99]
    shift-right: [w77] -> _
    shift-left: w1 -> [w98]
    shift-right: [w78] -> _
    shift-left: w1 -> [w97]
    shift-right: [w67] -> _
    shift-left: w1 -> [w69]
    shift-right: [w66] -> _
    shift-left: w1 -> [w68]
    shift-right: [w63] -> _
    shift-left: w1 -> [w65]
    shift-right: [w62] -> _
    shift-left: w1 -> [w64]
    i -> [w161]
    stop <- "Interrupt program" stop-if-true
    # "Vdg for bias stress plots"
    # "Idg for bias stress plots"
    # "Vp2 for FPP bias stress plots"
    # "Vp1 for FPP bias stress plots"
    # "Ig for bias stress plots"
    # "Id for bias stress plots"
    # "Is for bias stress plots"
    # "Time axis for bias stress plots"
    # "Save bias stress curves in file."
    # "Is off"
    # "Is on"
    # "Ig off"
    # "Ig on"
    # "Is min"
    # "Is max"
    # "Ig min"
    # "Ig max"
    # "Id min"
    # "Id max"
    # "Id off"
    # "Id on"
    # "Is off"
    # "Is on"
    # "Ig off"
    # "Ig on"
    # "Is min"
    # "Is max"
    # "Ig min"
    # "Ig max"
    # "Id min"
    # "Id max"
    # "Id off"
    # "Id on"
    # "Filepath and name"
    # "Limit of command arguments (array columns). Raise if needed."
    # "Serial port data (string)"
    # "Serial port data (table)"
    # "Serial port data"
    # "For loop counter"
    # "<-----Equivalent to the 4155C \"Write\" subvi.----->"
    # "Headers"
    # "Save transfer curves in file."
    # "Filepath and name"
    # "Save time-dependent data."
    # "Use the time offset if your measurements do not start at t=0."
    # "Time for Imax, Imin, Ion, Ioff"
    # "Rest of elements of command"
    # "First element of command\n(case select)"
    n20 = Add(x=w161, y=1) -> (x+y=→"Line running":i32)
    n21 = Add(x=w166, y=1) -> (x+y=→"Total lines":i32)
    n22 = Index Array(array=w194, index=0 ("line index")) -> (element=w189:string)
    "Command running:" <- w189
    n23 = control-ref of="Interrupt scan"() -> (w213:refnum<vi>)
    n24 = Spreadsheet String To Array(delimiter (Tab)=" ", format string="%s", spreadsheet string=w189, array type (2D Dbl)=string[] []) -> (array=w187:string[])
    n25 = Delete From Array(array=w187, index=0) -> (deleted portion=w141:string, array with subset deleted=w186:string[])  [unwired: 1 in]
    n26 = call "Elapsed Time"("Reset"="Reset", "Auto Reset"="Auto Reset") -> ("Elapsed Time (s)"=w196:dbl)  [unwired: 10 in, 7 out]
    n27 = case shown="2" "Time Units" {
      tunnel: ["-sec" "-min" "-h"] -> w197
      tunnel: [w226 w230 w233] -> w167
      tunnel: w196 -> [w226 w229 w234]
      frame 0, Default {
      }
      frame 1 {
        n28 = Divide(x=w229, y=60.0) -> (x/y=w230:dbl)
      }
      frame 2 {
        n29 = Divide(x=w234, y=3600.0) -> (x/y=w233:dbl)
      }
    }
    n30 = Add(x=w167, y="Time Offset") -> (x+y=w101:dbl)
    n31 = To Long Integer(number=w101) -> (32bit integer=w102:i32)
    "Elapsed Time" <- w102
    n32 = case shown="\"samplei\"" w141 {
      tunnel: w186 -> [w274 w315 w355 w375 w505 w626 w779 w905 w1080 w1115 w1192 w1241 w1288 w1331 w1367 _ _ w1565 w1716 _ w1837 w1905 w1970 w2091 w2243 w2329]
      tunnel: w222 -> [w269 w311 w353 w388 w512 w685 w786 w912 w1087 w1132 w1181 w1233 w1281 w1325 w1360 w1401 w1465 w1546 w1700 w1760 w1824 w1892 w1958 w2085 w2239 w2331]
      tunnel: w221 -> [w268 w310 w344 w387 w483 w670 w756 w883 w1056 w1133 w1182 w1234 w1282 w1326 w1361 w1406 w1467 w1571 w1722 w1764 w1843 w1911 w1976 w2097 w2203 w2335]
      tunnel: w220 -> [w267 w309 w343 w386 w482 w669 w755 w882 w1053 w1134 w1183 w1235 w1283 w1327 w1362 w1405 w1438 w1570 w1721 w1763 w1842 w1910 w1975 w2096 w2202 w2334]
      tunnel: w219 -> [w266 w308 w352 w384 w508 w646 w782 w908 w1083 w1142 w1191 w1232 w1280 w1324 w1359 w1404 w1462 w1538 w1692 w1769 w1817 w1885 w1951 w2084 w2238 w2336]
      tunnel: w218 -> [w265 w307 w351 w383 w510 w683 w784 w910 w1085 w1141 w1190 w1240 w1287 w1330 w1366 w1403 w1447 w1569 w1720 w1772 w1841 w1909 w1974 w2095 w2247 w2337]
      tunnel: w217 -> [w264 w306 w350 w381 w509 w682 w783 w909 w1084 w1140 w1189 w1239 w1286 w1329 w1365 w1402 w1448 w1547 w1701 w1771 w1825 w1893 w1959 w2086 w2240 w2339]
      tunnel: [w268 w310 w342 w387 w507 w680 w781 w907 w1082 w1133 w1182 w1234 w1282 w1326 w1361 w1406 w1467 w1539 w1674 w1762 w1818 w1886 w1952 w2044 w2205 w2335] -> w216
      tunnel: [w267 w309 w341 w386 w506 w679 w780 w906 w1081 w1134 w1183 w1235 w1283 w1327 w1362 w1405 w1437 w1548 w1675 w1761 w1826 w1894 w1960 w2043 w2204 w2333] -> w152
      tunnel: [w266 w308 w352 w384 w508 w642 w782 w908 w1083 w1135 w1184 w1232 w1280 w1324 w1359 w1404 w1462 w1538 w1692 w1769 w1817 w1885 w1951 w2084 w2238 w2336] -> w71
      tunnel: [w265 w307 w351 w383 w510 w683 w784 w910 w1085 w1141 w1190 w1240 w1287 w1330 w1366 w1403 w1447 w1569 w1720 w1772 w1841 w1909 w1974 w2095 w2247 w2337] -> w215
      tunnel: [w264 w306 w350 w381 w509 w682 w783 w909 w1084 w1140 w1189 w1239 w1286 w1329 w1365 w1402 w1448 w1547 w1701 w1771 w1825 w1893 w1959 w2086 w2240 w2339] -> w214
      tunnel: [w269 w311 w353 w388 w512 w685 w786 w912 w1087 w1132 w1181 w1233 w1281 w1325 w1360 w1401 w1465 w1546 w1700 w1760 w1824 w1892 w1958 w2085 w2239 w2331] -> w79
      tunnel: w213 -> [_ _ _ _ w514 w689 w790 w914 w1091 _ _ _ _ _ _ _ _ w1543 w1697 _ w1823 w1891 w1957 w2063 w2221 _]
      tunnel: "Gate" -> [_ _ _ _ w492 w673 w766 w892 w1067 _ _ _ _ _ _ _ _ _ _ _ _ _ _ _ _ _]
      tunnel: "Drain 2" -> [_ _ _ _ w491 w672 w765 w891 w1066 _ _ _ _ _ _ _ _ _ _ _ _ _ _ _ _ _]
      tunnel: "Panel Controls" -> [_ _ _ _ _ _ w764 w818 w1065 _ _ _ _ _ _ _ _ _ _ _ _ _ _ _ _ _]
      tunnel: w209 -> [w263 w305 w349 w380 w476 w663 w749 w876 w1051 w1139 w1188 _ w1279 w1323 w1358 w1400 w1449 w1534 w1688 w1765 w1813 w1881 w1947 w2080 w2234 w2340]
      tunnel: w208 -> [w262 w304 w348 w379 w475 w662 w748 w875 w1050 w1138 w1187 w1238 _ w1314 w1364 w1399 w1450 w1535 w1689 w1766 w1814 w1882 w1948 w2081 w2235 w2341]
      tunnel: w207 -> [w261 w303 w347 w378 w474 w661 w747 w874 w1049 w1137 w1186 w1237 w1285 w1328 _ w1398 w1451 w1536 w1690 w1767 w1815 w1883 w1949 w2082 w2236 w2342]
      tunnel: w206 -> [w260 w302 w346 w377 w473 w660 w746 w873 w1052 w1136 w1185 w1236 w1284 _ w1363 w1397 w1452 w1537 w1691 w1768 w1816 w1884 w1950 w2083 w2237 w2343]
      tunnel: [w263 w305 w349 w380 w476 w663 w749 w876 w1051 w1139 w1188 w1231 w1279 w1323 w1358 w1400 w1449 w1534 w1688 w1765 w1813 w1881 w1947 w2080 w2234 w2340] -> w205
      tunnel: [w262 w304 w348 w379 w475 w662 w748 w875 w1050 w1138 w1187 w1238 w1271 w1314 w1364 w1399 w1450 w1535 w1689 w1766 w1814 w1882 w1948 w2081 w2235 w2341] -> w204
      tunnel: [w261 w303 w347 w378 w474 w661 w747 w874 w1049 w1137 w1186 w1237 w1285 w1328 w1357 w1398 w1451 w1536 w1690 w1767 w1815 w1883 w1949 w2082 w2236 w2342] -> w203
      tunnel: [w260 w302 w346 w377 w473 w660 w746 w873 w1052 w1136 w1185 w1236 w1284 w1315 w1363 w1397 w1452 w1537 w1691 w1768 w1816 w1884 w1950 w2083 w2237 w2343] -> w202
      tunnel: w201 -> [w244 w283 w324 _ w414 w615 w721 w814 w1026 w1112 w1164 w1215 w1255 w1298 w1341 w1381 w1415 w1521 w1655 w1744 w1784 w1856 w1923 w2030 w2187 w2300]
      tunnel: w200 -> [_ _ _ _ w467 w657 _ _ _ _ _ _ _ _ _ _ _ _ _ _ _ _ _ _ _ _]
      tunnel: [w259 w298 w339 w392 w429 w634 w739 w830 w1044 w1131 w1179 w1230 w1270 w1313 w1356 w1396 w1433 w1511 w1659 w1759 w1802 w1874 w1941 w2005 w2166 w2332] -> w119
      tunnel: w199 -> [w259 w298 w339 w392 w464 w634 w739 w865 w1044 w1131 w1179 w1230 w1270 w1313 w1356 w1396 w1433 w1517 w1659 w1759 w1802 w1874 w1941 w2011 w2172 w2332]
      tunnel: w101 -> [_ _ _ _ w463 w631 w737 w864 w1041 _ _ _ _ _ _ _ w1431 w1526 w1671 _ w1799 w1871 w1938 w2040 w2196 _]
      tunnel: w197 -> [_ _ _ _ w460 w630 w735 w861 w1040 _ _ _ _ _ _ _ w1429 w1524 w1670 _ w1798 w1870 w1937 w2039 w2197 _]
      tunnel: w102 -> [_ _ _ _ w456 _ _ w857 _ _ _ _ _ _ _ _ _ _ _ _ _ _ _ _ _ _]
      tunnel: [w258 w297 w338 w382 w433 w633 w738 w834 w1043 w1130 w1178 w1229 w1269 w1312 w1355 w1395 w1432 w1496 w1643 w1758 w1801 w1873 w1940 w1999 w2161 w2338] -> w153
      tunnel: w195 -> [w258 w297 w338 w382 w459 w633 w738 w860 w1043 w1130 w1178 w1229 w1269 w1312 w1355 w1395 w1432 w1498 w1644 w1758 w1801 w1873 w1940 w2000 w2163 w2338]
      tunnel: [w257 w296 w337 w391 w428 w629 w734 w829 w1039 w1129 w1177 w1228 w1268 w1311 w1354 w1394 w1428 w1510 w1658 w1757 w1797 w1869 w1936 w2004 w2165 w2327] -> w118
      tunnel: w171 -> [w257 w296 w337 w391 w455 w629 w734 w856 w1039 w1129 w1177 w1228 w1268 w1311 w1354 w1394 w1428 w1516 w1658 w1757 w1797 w1869 w1936 w2010 w2171 w2327]
      tunnel: [w256 w295 w336 w376 w448 w628 w733 w849 w1038 w1128 w1176 w1227 w1267 w1310 w1353 w1393 w1427 w1523 w1669 w1756 w1796 w1868 w1935 w2038 w2195 w2326] -> w148
      tunnel: w158 -> [w256 w295 w336 w376 w448 w628 w733 w849 w1038 w1128 w1176 w1227 w1267 w1310 w1353 w1393 w1427 w1523 w1669 w1756 w1796 w1868 w1935 w2038 w2195 w2325]
      tunnel: [w255 w294 w335 w385 w447 w627 w732 w848 w1037 w1127 w1175 w1226 w1266 w1309 w1352 w1392 w1426 w1522 w1668 w1755 w1795 w1867 w1934 w2037 w2194 w2311] -> w149
      tunnel: w151 -> [w255 w294 w335 w385 w447 w627 w732 w848 w1037 w1127 w1175 w1226 w1266 w1309 w1352 w1392 w1426 w1522 w1668 w1755 w1795 w1867 w1934 w2037 w2194 w2311]
      tunnel: [w253 w292 w333 w397 w422 w624 w730 w823 w1035 w1125 w1174 w1225 w1264 w1307 w1350 w1390 w1424 w1504 w1667 w1754 w1794 w1866 w1932 w2036 w2193 w2310] -> w112
      tunnel: w140 -> [w253 w292 w333 w397 w446 w624 w730 w847 w1035 w1125 w1174 w1225 w1264 w1307 w1350 w1390 w1424 w1504 w1667 w1754 w1794 w1866 w1932 w2036 w2193 w2310]
      tunnel: [w254 w293 w334 w398 w423 w625 w731 w824 w1036 w1126 w1173 w1224 w1265 w1308 w1351 w1391 w1425 w1505 w1666 w1753 w1793 w1865 w1933 w2035 w2192 w2309] -> w113
      tunnel: w139 -> [w254 w293 w334 w398 w445 w625 w731 w846 w1036 w1126 w1173 w1224 w1265 w1308 w1351 w1391 w1425 w1505 w1666 w1753 w1793 w1865 w1933 w2035 w2192 w2309]
      tunnel: [w246 w285 w326 w390 w427 w621 w728 w828 w1033 w1118 w1171 w1222 w1262 w1305 w1348 w1388 w1417 w1509 w1657 w1752 w1786 w1858 w1925 w2003 w2168 w2302] -> w117
      tunnel: w128 -> [w246 w285 w326 w390 w441 w621 w728 w842 w1033 w1118 w1171 w1222 w1262 w1305 w1348 w1388 w1417 w1515 w1657 w1752 w1786 w1858 w1925 w2009 w2170 w2302]
      tunnel: [w245 w284 w325 w389 w426 w622 w729 w827 w1034 w1117 w1172 w1223 w1263 w1306 w1349 w1389 w1416 w1508 w1656 w1751 w1785 w1857 w1924 w2002 w2167 w2301] -> w116
      tunnel: w127 -> [w245 w284 w325 w389 w440 w622 w729 w841 w1034 w1117 w1172 w1223 w1263 w1306 w1349 w1389 w1416 w1514 w1656 w1751 w1785 w1857 w1924 w2008 w2169 w2301]
      tunnel: [w248 w287 w328 w394 w432 w620 w726 w833 w1031 w1123 w1169 w1220 w1260 w1303 w1346 w1386 w1419 w1513 w1661 w1746 w1788 w1860 w1927 w2007 w2174 w2306] -> w110
      tunnel: w126 -> [w248 w287 w328 w394 w439 w620 w726 w840 w1031 w1123 w1169 w1220 w1260 w1303 w1346 w1386 w1419 w1519 w1661 w1746 w1788 w1860 w1927 w2013 w2176 w2306]
      tunnel: [w247 w286 w327 w393 w430 w623 w727 w831 w1032 w1124 w1170 w1221 w1261 w1304 w1347 w1387 w1418 w1512 w1660 w1745 w1787 w1859 w1926 w2006 w2164 w2305] -> w120
      tunnel: w125 -> [w247 w286 w327 w393 w438 w623 w727 w839 w1032 w1124 w1170 w1221 w1261 w1304 w1347 w1387 w1418 w1518 w1660 w1745 w1787 w1859 w1926 w2012 w2173 w2305]
      tunnel: [w250 w289 w330 w396 w421 w619 w724 w822 w1029 w1121 w1167 w1218 w1258 w1301 w1344 w1384 w1421 w1503 w1663 w1748 w1790 w1862 w1929 w2032 w2189 w2308] -> w111
      tunnel: w124 -> [w250 w289 w330 w396 w437 w619 w724 w838 w1029 w1121 w1167 w1218 w1258 w1301 w1344 w1384 w1421 w1503 w1663 w1748 w1790 w1862 w1929 w2032 w2189 w2308]
      tunnel: [w249 w288 w329 w395 w420 w618 w725 w821 w1030 w1122 w1168 w1219 w1259 w1302 w1345 w1385 w1420 w1502 w1662 w1747 w1789 w1861 w1928 w2031 w2188 w2307] -> w109
      tunnel: w123 -> [w249 w288 w329 w395 w436 w618 w725 w837 w1030 w1122 w1168 w1219 w1259 w1302 w1345 w1385 w1420 w1502 w1662 w1747 w1789 w1861 w1928 w2031 w2188 w2307]
      tunnel: [w252 w291 w332 w400 w425 w617 w722 w826 w1027 w1119 w1165 w1216 w1256 w1299 w1342 w1382 w1423 w1507 w1665 w1750 w1792 w1864 w1931 w2034 w2191 w2304] -> w115
      tunnel: w122 -> [w252 w291 w332 w400 w435 w617 w722 w836 w1027 w1119 w1165 w1216 w1256 w1299 w1342 w1382 w1423 w1507 w1665 w1750 w1792 w1864 w1931 w2034 w2191 w2304]
      tunnel: [w251 w290 w331 w399 w424 w616 w723 w825 w1028 w1120 w1166 w1217 w1257 w1300 w1343 w1383 w1422 w1506 w1664 w1749 w1791 w1863 w1930 w2033 w2190 w2303] -> w114
      tunnel: w121 -> [w251 w290 w331 w399 w434 w616 w723 w835 w1028 w1120 w1166 w1217 w1257 w1300 w1343 w1383 w1422 w1506 w1664 w1749 w1791 w1863 w1930 w2033 w2190 w2303]
      tunnel: [w244 w283 w324 w366 w414 w615 w721 w814 w1026 w1112 w1164 w1215 w1255 w1298 w1341 w1381 w1415 w1521 w1655 w1744 w1784 w1856 w1923 w2030 w2187 w2300] -> w70
      tunnel: w101 -> [_ _ _ _ _ _ _ _ _ _ _ _ _ _ _ _ _ w1473 w1639 _ _ _ _ w2014 w2180 _]
      tunnel: [w243 w282 w323 w365 w413 w614 w720 w813 w1025 w1111 w1163 w1214 w1254 w1297 w1340 w1380 w1414 w1485 w1654 w1743 w1783 w1855 w1922 w2020 w2183 w2299] -> w75
      tunnel: [w242 w281 w322 w364 w412 w613 w719 w812 w1024 w1110 w1162 w1213 w1253 w1296 w1339 w1379 w1413 w1482 w1653 w1742 w1782 w1854 w1921 w1981 w2144 w2298] -> w76
      tunnel: [w241 w280 w321 w363 w411 w612 w718 w811 w1023 w1109 w1161 w1212 w1252 w1295 w1338 w1378 w1412 w1483 w1626 w1741 w1781 w1853 w1920 w1993 w2156 w2297] -> w77
      tunnel: [w240 w279 w320 w362 w410 w611 w717 w810 w1022 w1108 w1160 w1211 w1251 w1294 w1337 w1377 w1411 w1484 w1633 w1740 w1780 w1852 w1919 w1989 w2152 w2296] -> w78
      tunnel: w100 -> [w243 w282 w323 w365 w413 w614 w720 w813 w1025 w1111 w1163 w1214 w1254 w1297 w1340 w1380 w1414 w1489 w1654 w1743 w1783 w1855 w1922 w2023 w2186 w2299]
      tunnel: w99 -> [w242 w281 w322 w364 w412 w613 w719 w812 w1024 w1110 w1162 w1213 w1253 w1296 w1339 w1379 w1413 w1488 w1653 w1742 w1782 w1854 w1921 w2022 w2185 w2298]
      tunnel: w98 -> [w241 w280 w321 w363 w411 w612 w718 w811 w1023 w1109 w1161 w1212 w1252 w1295 w1338 w1378 w1412 w1487 w1627 w1741 w1781 w1853 w1920 w1993 w2156 w2297]
      tunnel: w97 -> [w240 w279 w320 w362 w410 w611 w717 w810 w1022 w1108 w1160 w1211 w1251 w1294 w1337 w1377 w1411 w1486 w1635 w1740 w1780 w1852 w1919 w2021 w2184 w2296]
      tunnel: "Standby" -> [_ _ _ _ w409 w610 _ w809 _ _ _ _ _ _ _ _ _ w1480 w1652 _ _ _ _ w2029 _ _]
      tunnel: w69 -> [w239 w278 w319 w361 w404 w604 w711 w803 w1015 w1107 w1159 w1210 w1250 w1293 w1336 w1376 w1410 w1471 w1647 w1739 w1776 w1849 w1917 w1987 w2150 w2295]
      tunnel: w68 -> [w238 w277 w318 w360 w403 w603 w710 w804 w1016 w1106 w1158 w1209 w1249 w1292 w1335 w1375 w1409 w1470 w1646 w1738 w1775 w1848 w1916 w1986 w2149 w2294]
      tunnel: [w239 w278 w319 w361 w404 w604 w711 w803 w1015 w1107 w1159 w1210 w1250 w1293 w1336 w1376 w1410 w1471 w1647 w1739 w1776 w1849 w1917 w1982 w2145 w2295] -> w67
      tunnel: [w238 w277 w318 w360 w403 w603 w710 w804 w1016 w1106 w1158 w1209 w1249 w1292 w1335 w1375 w1409 w1470 w1646 w1738 w1775 w1848 w1916 w1985 w2148 w2294] -> w66
      tunnel: w65 -> [w237 w276 w317 w359 w401 w601 w700 w801 w1001 w1104 w1156 w1207 w1247 w1290 w1333 w1373 w1407 w1469 w1632 w1737 w1774 w1847 w1915 w1980 w2143 w2293]
      tunnel: w64 -> [w236 w275 w316 w358 w402 w602 w701 w802 w1002 w1105 w1157 w1208 w1248 w1291 w1334 w1374 w1408 w1468 w1631 w1736 w1773 w1846 w1914 w1979 w2142 w2292]
      tunnel: [w237 w276 w317 w359 w401 w601 w700 w801 w1001 w1104 w1156 w1207 w1247 w1290 w1333 w1373 w1407 w1469 w1624 w1737 w1774 w1847 w1915 w1980 w2143 w2293] -> w63
      tunnel: [w236 w275 w316 w358 w402 w602 w701 w802 w1002 w1105 w1157 w1208 w1248 w1291 w1334 w1374 w1408 w1468 w1630 w1736 w1773 w1846 w1914 w1979 w2142 w2292] -> w62
      frame "wait" {
        n33 = Index Array(array=w274, index=0 ("Index")) -> (element=w272:string)
        n34 = Decimal String To Number(string=w272, default (0L)=u32 0) -> (number=w271:u32)  [unwired: 1 in, 1 out]
        n35 = Wait (ms)(milliseconds to wait=w271) -> ()  [unwired: 1 out]
      }
      frame "wait-min" {
        n36 = Index Array(array=w315, index=0 ("Index")) -> (element=w313:string)
        n37 = Decimal String To Number(string=w313, default (0L)=u32 0) -> (number=w301:u32)  [unwired: 1 in, 1 out]
        n38 = Multiply(x=w301, y=u32 60000) -> (x*y=w300:u32)
        n39 = Wait (ms)(milliseconds to wait=w300) -> ()  [unwired: 1 out]
      }
      frame "standby" {
        n40 = Index Array(array=w355, index=0 ("Index")) -> (element=w345:string)
        n41 = case shown="\"off\", Default" w345 {
          tunnel: [":PAGE:SCON:STAN 0" ":PAGE:SCON:STAN 1"] -> w340
          frame "off", Default {
          }
          frame "on" {
          }
        }
        n42 = VISA Write(VISA resource name=w344, write buffer=w340, error in (no error)=w343) -> (VISA resource name out=w342:refnum<visa-resource-name>, error out=w341:errorcluster)  [unwired: 1 out]
      }
      frame "Probe4" {
        n43 = Delete From Array(array=w375, index=0) -> (deleted portion=w369:string, array with subset deleted=w372:string[])  [unwired: 1 in]
        n44 = Equal?(x=w369, y="ON") -> (x = y?=w367:bool)
        n45 = Delete From Array(array=w372, index=0) -> (deleted portion=w371:string)  [unwired: 1 in, 1 out]
        n46 = Fract/Exp String To Number(string=w371) -> (number=w368:dbl)  [unwired: 3 in, 1 out]
        n47 = Bundle(w367, w368) -> (w366:cluster{bool, dbl})  [unwired: 1 in]
      }
      frame "transfer" {
        n48 = local read "Transfer/Output - Gate"() -> (w408:u32)
        n49 = Delete From Array(array=w505, index=0 ("Index")) -> (deleted portion=w503:string, array with subset deleted=w502:string[])  [unwired: 1 in]
        n50 = Bundle By Name(cluster=w467, "Emergency Stop"=w514) -> (w468:T2)
        n51 = Number To Decimal String(number=w463) -> (decimal integer string=w462:string)  [unwired: 1 in]
        n52 = case shown="\"d\", Default" w503 {
          tunnel: [w599 w600] -> w501
          frame "s" {
            w599 = u16 0 items=["Single", "Double"] ("sweep mode")
          }
          frame "d", Default {
            w600 = u16 1 items=["Single", "Double"] ("sweep mode")
          }
        }
        n53 = Fract/Exp String To Number(string=w502) -> (number=w487:dbl[])  [unwired: 3 in, 1 out]
        n54 = Concatenate Strings(w512, "-transfer-" ("Prefix"), w462, w460, ".txt" ("Suffix (transfer)")) -> (w513:string)
        n55 = VISA Write(VISA resource name=w483, write buffer=":PAGE:CHAN:MODE SWE;" ("write buffer (\"\")"), error in (no error)=w482) -> (VISA resource name out=w480:refnum<visa-resource-name>, error out=w481:errorcluster)  [unwired: 1 out]
        n56 = local read "Plot transfer curve extrema vs time"() -> (w415:bool)
        n57 = String To Path(string=w513) -> (path=w511:path)
        n58 = Index Array(array=w487, index #1=0 ("Index")) -> (element #1=w500:dbl, element #2=w499:dbl, element #3=w498:dbl)  [unwired: 2 in]
        n59 = Delete From Array(array=w487, length=3 ("Length"), index=0 ("Index")) -> (array with subset deleted=w485:dbl[])  [unwired: 1 out]
        n60 = local read "Transfer/Output - Drain"() -> (w405:u32)
        n61 = local read "Transfer/Output - Source/Common"() -> (w407:u32)
        n62 = case shown="True" w415 {
          tunnel: w459 -> [w516 w519]
          tunnel: w456 -> [_ w518]
          tunnel: [w516 w517] -> w433
          frame False {
          }
          frame True {
            n63 = Build Array (concatenate)(w519, w518) -> (w517:i32[])
          }
        }
        n64 = local read "Transfer/Output - Probe 4"() -> (w406:u32)
        n65 = Bundle By Name(cluster=w492, "Gate Start"=w500, "Gate Stop"=w499, "Gate Step (linear only)"=w498, "Gate Compliance"=w509, "Range mode"=w476, "Range"=w475) -> (w477:T6)
        n66 = Index Array(array=w485, index #1=0 ("Index")) -> (element #1=w495:dbl, element #2=w494:dbl, element #3=w493:dbl)  [unwired: 2 in]
        n67 = call <vilib>:"compatOverwrite.vi"("overwrite (F)"=TRUE) -> ("overwrite?"=w466:T8)
        n68 = Bundle By Name(cluster=w491, "Drain Start"=w495, "Drain Stop"=w494, "Drain Step"=w493, "Drain Compliance"=w510, "Range mode"=w474, "Range"=w473) -> (w478:T7)
        n69 = call "4155C Transfer v3.0.vi"("VISA resource name in"=w480, "Source/Common"=w407, 2:"Gate"=w477, 3:"Drain"=w478, 4:"Drain"=w405, "Timings"=w508, "error in (no error)"=w481, 7:"Probe 4"=w414, 8:"Gate"=w408, 9:"Probe 4"=w406, "sweep mode"=w501, "Panel Controls"=w468, "Standby"=w409) -> ("VG"=w465:dbl[], "Outparams"=w472:T9, "VISA Resource Name out"=w507:refnum<visa-resource-name>, "IS"=w443:dbl[], "ID"=w444:dbl[], "IG"=w442:dbl[], "error out"=w457:errorcluster, "Probe 4"=w469:dbl[])  [unwired: 7 in]
        n70 = Unbundle By Name(w472) -> ("V2 Step"=w471:dbl, "V2 Start"=w470:dbl, "Number of points"=w431:i32)
        n71 = call "4155C Split array.vi"("Number of VAR2 steps"=w431, "Y2 data in"=w444, "X data in"=w465, "Y1 data in"=w443, "Y3 data in"=w442, "error in (no error)"=w457) -> ("Array of clusters"=w458:cluster{"Y data in":dbl[], "X data in":dbl[]}[], "error out"=w419:errorcluster)  [unwired: 1 in]
        n72 = case shown="True" "Plot transfer curve extrema vs time" {
          tunnel: w464 -> [w522 w598]
          tunnel: w455 -> [w523 w593]
          tunnel: w446 -> [w529 w589]
          tunnel: w445 -> [w530 w588]
          tunnel: w444 -> [_ w585]
          tunnel: w443 -> [_ w583]
          tunnel: w442 -> [_ w582]
          tunnel: w441 -> [w524 w578]
          tunnel: w440 -> [w526 w577]
          tunnel: w439 -> [w520 w574]
          tunnel: w438 -> [w521 w573]
          tunnel: w437 -> [w528 w570]
          tunnel: w436 -> [w527 w569]
          tunnel: w435 -> [w532 w566]
          tunnel: w434 -> [w531 w565]
          tunnel: w433 -> [_ w558]
          tunnel: [w520 w553] -> w432
          tunnel: w431 -> [_ w552]
          tunnel: [w521 w551] -> w430
          tunnel: [w522 w550] -> w429
          tunnel: [w523 w549] -> w428
          tunnel: [w524 w548] -> w427
          tunnel: [w526 w547] -> w426
          tunnel: [w532 w546] -> w425
          tunnel: [w531 w545] -> w424
          tunnel: [w530 w544] -> w423
          tunnel: [w529 w543] -> w422
          tunnel: [w528 w542] -> w421
          tunnel: [w527 w541] -> w420
          tunnel: w419 -> [w525 w540]
          tunnel: [w525 w536] -> w418
          frame False {
          }
          frame True {
            # "Adjusts graph colors."
            # "Adjusts graph colors."
            # "Ion will be the middle element of the array. The calculation of the index is done only once, since Is, Id, and Ig have the same dimensions."
            # "abs(Ig)"
            # "abs(Is)"
            # "Y1: Is\nY2: Id\nY3: Ig"
            # "abs(Id)"
            # "Adjusts graph colors."
            # "Adjusts graph colors."
            # "Adjusts graph colors."
            n73 = Absolute Value(x=w583) -> (abs(x)=w568:dbl[])
            n74 = Absolute Value(x=w585) -> (abs(x)=w584:dbl[])
            n75 = Absolute Value(x=w582) -> (abs(x)=w571:dbl[])
            n76 = Array Size(array=w584) -> (size(s)=w592:i32)
            n77 = Divide(x=w592, y=2) -> (x/y=w535:dbl)
            n78 = Subtract(x=w535, y=1) -> (x-y=w534:dbl)
            n79 = Array Max & Min(array=w568) -> (max value=w575:dbl, min value=w576:dbl)  [unwired: 2 out]
            n80 = Array Max & Min(array=w584) -> (max value=w597:dbl, min value=w581:dbl)  [unwired: 2 out]
            n81 = Array Max & Min(array=w571) -> (max value=w580:dbl, min value=w579:dbl)  [unwired: 2 out]
            n82 = Index Array(array=w568, index=w534) -> (element=w559:dbl)
            n83 = Index Array(array=w568, index=0) -> (element=w560:dbl)
            n84 = Index Array(array=w584, index=w534) -> (element=w561:dbl)
            n85 = Index Array(array=w584, index=0) -> (element=w562:dbl)
            n86 = Index Array(array=w571, index=w534) -> (element=w564:dbl)
            n87 = Index Array(array=w571, index=0) -> (element=w563:dbl)
            n88 = local write "Ig max"(w580) -> ()
            n89 = local write "Ig min"(w579) -> ()
            n90 = local write "Is max"(w575) -> ()
            n91 = local write "Is min"(w576) -> ()
            n92 = local write "Id max"(w597) -> ()
            n93 = local write "Id min"(w581) -> ()
            n94 = Build Array (concatenate)(w574, w575) -> (w553:dbl[])
            n95 = Build Array (concatenate)(w573, w576) -> (w551:dbl[])
            n96 = local write "Is off"(w560) -> ()
            n97 = local write "Is on"(w559) -> ()
            n98 = Build Array (concatenate)(w598, w597) -> (w550:dbl[])
            n99 = Build Array (concatenate)(w593, w581) -> (w549:dbl[])
            n100 = Build Array (concatenate)(w578, w580) -> (w548:dbl[])
            n101 = Build Array (concatenate)(w577, w579) -> (w547:dbl[])
            n102 = Build Array (concatenate)(w566, w559) -> (w546:dbl[])
            n103 = Build Array (concatenate)(w565, w560) -> (w545:dbl[])
            n104 = Build Array (concatenate)(w588, w561) -> (w544:dbl[])
            n105 = Build Array (concatenate)(w589, w562) -> (w543:dbl[])
            n106 = Build Array (concatenate)(w570, w564) -> (w542:dbl[])
            n107 = Build Array (concatenate)(w569, w563) -> (w541:dbl[])
            n108 = local write "Ig off"(w563) -> ()
            n109 = local write "Ig on"(w564) -> ()
            n110 = local write "Id off"(w562) -> ()
            n111 = local write "Id on"(w561) -> ()
            n112 = control-ref of="Imax vs time"() -> (w587:refnum<vi>)
            n113 = control-ref of="Imin vs time"() -> (w586:refnum<vi>)
            n114 = control-ref of="Ion vs time"() -> (w555:refnum<vi>)
            n115 = control-ref of="Ioff vs time"() -> (w554:refnum<vi>)
            n116 = control-ref of="I vs Vg"() -> (w596:refnum<vi>)
            n117 = call "4155C Split array.vi"("Number of VAR2 steps"=w552, "Y2 data in"=w544, "X data in"=w558, "Y1 data in"=w546, "Y3 data in"=w542, "error in (no error)"=w540) -> ("Array of clusters"=w556:cluster{"Y data in":dbl[], "X data in":dbl[]}[], "error out"=w539:errorcluster)  [unwired: 1 in]
            n118 = call "4155C Split array.vi"("Number of VAR2 steps"=w552, "Y2 data in"=w543, "X data in"=w558, "Y1 data in"=w545, "Y3 data in"=w541, "error in (no error)"=w539) -> ("Array of clusters"=w557:cluster{"Y data in":dbl[], "X data in":dbl[]}[], "error out"=w538:errorcluster)  [unwired: 1 in]
            n119 = call "4155C Split array.vi"("Number of VAR2 steps"=w552, "Y2 data in"=w550, "X data in"=w558, "Y1 data in"=w553, "Y3 data in"=w548, "error in (no error)"=w538) -> ("Array of clusters"=w595:cluster{"Y data in":dbl[], "X data in":dbl[]}[], "error out"=w537:errorcluster)  [unwired: 1 in]
            n120 = call "4155C Split array.vi"("Number of VAR2 steps"=w552, "Y2 data in"=w549, "X data in"=w558, "Y1 data in"=w551, "Y3 data in"=w547, "error in (no error)"=w537) -> ("Array of clusters"=w594:cluster{"Y data in":dbl[], "X data in":dbl[]}[], "error out"=w536:errorcluster)  [unwired: 1 in]
            n121 = call "4155C Config Chart Colours.vi"("Numeric"=w552, "XY Graph 2"=w587) -> ()  [unwired: 6 in]
            n122 = call "4155C Config Chart Colours.vi"("Numeric"=w552, "XY Graph 2"=w586) -> ()  [unwired: 6 in]
            n123 = call "4155C Config Chart Colours.vi"("Numeric"=w552, "XY Graph 2"=w555) -> ()  [unwired: 6 in]
            n124 = call "4155C Config Chart Colours.vi"("Numeric"=w552, "XY Graph 2"=w554) -> ()  [unwired: 6 in]
            n125 = call "4155C Config Chart Colours.vi"("Numeric"=w552, "XY Graph 2"=w596) -> ()  [unwired: 6 in]
            n126 = local write "Imax vs time"(w595) -> ()
            n127 = local write "Imin vs time"(w594) -> ()
            n128 = local write "Ion vs time"(w556) -> ()
            n129 = local write "Ioff vs time"(w557) -> ()
          }
        }
        n130 = local write "I vs Vg"(w458) -> ()
        n131 = Open/Create/Replace File(file path (use dialog)=w511, error in=w418, operation (0:open)=w466) -> (refnum out=w453:refnum<file>, error out=w451:errorcluster)  [unwired: 3 in, 1 out]
        n132 = call "4155C Make Big 2d array.vi"("1D Var1"=w465, "1d IS"=w443, "1d ID"=w444, "1d IG"=w442, "1d SMU4"=w469, "SMU4"=w414, "VAR2 START"=w470, "Number of VAR2 steps"=w431, "VAR2 STEP"=w471, "VAR1 Name"="Vg", "Decimal places in header"=i8 1, "VAR2 Name"="Vd") -> ("Header array"=w454:string[], "Data array"=w452:dbl[][])  [unwired: 14 in]
        n133 = call "4155C Write array to file.vi"("Byte Stream File Refnum"=w453, "Header"=w454, "Data Array"=w452, "error in (no error)"=w451) -> ("dup refnum"=w450:refnum<file>, "error out"=w449:errorcluster)  [unwired: 1 in]
        n134 = Close File(refnum=w450, error in=w449) -> (error out=w506:errorcluster)  [unwired: 1 out]
      }
      frame "pulsedstressV" {
        w640 = 0
        n135 = local read "Pulsed Stress V - Vextra"() -> (w607:u32)
        n136 = local read "Pulsed Stress V - Drain"() -> (w609:u32)
        n137 = local read "Pulsed Stress V - Gate"() -> (w606:u32)
        n138 = local read "Pulsed Stress V - Probe 4"() -> (w608:u32)
        n139 = local read "Pulsed Stress V - Source/Common"() -> (w605:u32)
        n140 = Number To Decimal String(number=w631) -> (decimal integer string=w686:string)  [unwired: 1 in]
        n141 = Delete From Array(array=w626, index=0 ("Index")) -> (deleted portion=w677:string, array with subset deleted=w676:string[])  [unwired: 1 in]
        n142 = Bundle By Name(cluster=w657, "Emergency Stop"=w689) -> (w658:T2)
        n143 = VISA Write(VISA resource name=w670, write buffer=":PAGE:CHAN:MODE SWE;" ("write buffer (\"\")"), error in (no error)=w669) -> (VISA resource name out=w667:refnum<visa-resource-name>, error out=w668:errorcluster)  [unwired: 1 out]
        n144 = Concatenate Strings(w685, "-pulsedstressV-" ("Substring"), w686, w630, ".txt" ("Substring")) -> (w688:string)
        n145 = case shown="\"d\", Default" w677 {
          tunnel: [w698 w699] -> w675
          frame "s" {
            w698 = u16 0 items=["Single", "Double"] ("sweep mode")
          }
          frame "d", Default {
            w699 = u16 1 items=["Single", "Double"] ("sweep mode")
          }
        }
        n146 = Fract/Exp String To Number(string=w676) -> (number=w671:dbl[])  [unwired: 3 in, 1 out]
        n147 = String To Path(string=w688) -> (path=w684:path)
        n148 = Index Array(array=w671, index #1=0 ("Index")) -> (element #1=w649:dbl, element #2=w648:dbl, element #3=w645:dbl, element #4=w644:dbl, element #5=w643:dbl, element #6=w647:dbl)  [unwired: 5 in]
        n149 = Bundle By Name(cluster=w646, "Pulse period"=w644, "Base voltage"=w645, "Pulse width"=w643) -> (w642:T4)
        n150 = Unbundle By Name(w642) -> ("Pulse period"=w650:dbl)
        n151 = Bundle By Name(cluster=w673, "Gate Start"=w648, "Gate Stop"=w649, "Gate Step (linear only)"=0, "Gate Compliance"=w682, "Range mode"=w663, "Range"=w662) -> (w664:T6)
        n152 = call <vilib>:"compatOverwrite.vi"("overwrite (F)"=TRUE) -> ("overwrite?"=w635:T8)
        n153 = Bundle By Name(cluster=w672, "Drain Start"=w647, "Drain Stop"=w640, "Drain Step"=w640, "Drain Compliance"=w683, "Range mode"=w661, "Range"=w660) -> (w665:T7)
        n154 = call "4155C PulsedStressV v3.0.vi"("VISA resource name in"=w667, "Gate"=w664, "Pulsed Stress V - Source/Common"=w605, "Drain"=w665, "Timings"=w642, "error in (no error)"=w668, "sweep mode"=w675, "Probe 4"=w615, "Pulsed Stress V - Drain"=w609, "Pulsed Stress V - Gate"=w606, "Panel Controls"=w658, "Standby"=w610, "Pulsed Stress V - Probe 4"=w608, "Pulsed Stress V - Vextra"=w607) -> ("Outparams"=w659:T9, "VISA Resource Name out"=w680:refnum<visa-resource-name>, "ID"=w638:dbl[], "IG"=w636:dbl[], "error out"=w681:errorcluster)  [unwired: 1 in]
        n155 = Unbundle By Name(w659) -> ("Number of points"=w637:i32)  [unwired: 2 out]
        n156 = for {
          N: w637 -> [_]
          tunnel: [w695] -> w639 mode=indexing
          tunnel: w650 -> [w697]
          i -> [w696]
          n157 = Multiply(x=w697, y=w696) -> (x*y=w695:dbl)
        }
        n158 = Insert Into Array(array=dbl[][] [] ("Input Array"), new element=w639) -> (w651:dbl[][])  [unwired: 2 in]
        n159 = Insert Into Array(array=w651, new element=w638) -> (w656:dbl[][])  [unwired: 2 in]
        n160 = Insert Into Array(array=w656, new element=w636) -> (w655:dbl[][])  [unwired: 2 in]
        n161 = Transpose 2D Array(2D array=w655) -> (transposed array=w654:dbl[][])
        n162 = Open/Create/Replace File(file path (use dialog)=w684, error in=w681, operation (0:open)=w635) -> (refnum out=w692:refnum<file>, error out=w693:errorcluster)  [unwired: 3 in, 1 out]
        n163 = call "4155C Write array to file.vi"("Byte Stream File Refnum"=w692, "Header"=string[] ["Time /s", "Id /A", "Ig /A"], "Data Array"=w654, "error in (no error)"=w693) -> ("dup refnum"=w690:refnum<file>, "error out"=w691:errorcluster)  [unwired: 1 in]
        n164 = Close File(refnum=w690, error in=w691) -> (error out=w679:errorcluster)  [unwired: 1 out]
      }
      frame "transfer-fpp" {
        # "Adjusts graph colors."
        # "Y1 = Y2 = ID\nY3 = IG"
        n165 = local read "FPP - Source"() -> (w716:u32)
        n166 = local read "FPP - Drain"() -> (w714:u32)
        n167 = local read "FPP - Gate"() -> (w715:u32)
        n168 = local read "FPP - Probe 1"() -> (w712:u32)
        n169 = local read "FPP - Probe 2"() -> (w713:u32)
        n170 = Number To Decimal String(number=w737) -> (decimal integer string=w787:string)  [unwired: 1 in]
        n171 = Bundle By Name(cluster=w764, "Emergency Stop"=w790) -> (w798:T1)
        n172 = Delete From Array(array=w779, index=0 ("Index")) -> (deleted portion=w777:string, array with subset deleted=w776:string[])  [unwired: 1 in]
        n173 = Concatenate Strings(w786, "-transferfpp-" ("Substring"), w787, w735, ".txt" ("Substring")) -> (w789:string)
        n174 = VISA Write(VISA resource name=w756, write buffer=":PAGE:CHAN:MODE SWE;" ("write buffer (\"\")"), error in (no error)=w755) -> (VISA resource name out=w753:refnum<visa-resource-name>, error out=w754:errorcluster)  [unwired: 1 out]
        n175 = case shown="\"d\", Default" w777 {
          tunnel: [w799 w800] -> w775
          frame "s" {
            w799 = u16 0 items=["Single", "Double"] ("sweep mode")
          }
          frame "d", Default {
            w800 = u16 1 items=["Single", "Double"] ("sweep mode")
          }
        }
        n176 = Fract/Exp String To Number(string=w776) -> (number=w760:dbl[])  [unwired: 3 in, 1 out]
        n177 = String To Path(string=w789) -> (path=w785:path)
        n178 = Index Array(array=w760, index #1=0 ("Index")) -> (element #1=w774:dbl, element #2=w773:dbl, element #3=w772:dbl)  [unwired: 2 in]
        n179 = Delete From Array(array=w760, length=3 ("Length"), index=0 ("Index")) -> (array with subset deleted=w758:dbl[])  [unwired: 1 out]
        n180 = control-ref of="I vs Vg"() -> (w703:refnum<vi>)
        n181 = Bundle By Name(cluster=w766, "Gate Start"=w774, "Gate Stop"=w773, "Gate Step (linear only)"=w772, "Gate Compliance"=w783, "Range mode"=w749, "Range"=w748) -> (w750:T6)
        n182 = Index Array(array=w758, index #1=0 ("Index")) -> (element #1=w769:dbl, element #2=w768:dbl, element #3=w767:dbl)  [unwired: 2 in]
        n183 = call <vilib>:"compatOverwrite.vi"("overwrite (F)"=TRUE) -> ("overwrite?"=w740:T8)
        n184 = Bundle By Name(cluster=w765, "Drain Start"=w769, "Drain Stop"=w768, "Drain Step"=w767, "Drain Compliance"=w784, "Range mode"=w747, "Range"=w746) -> (w751:T7)
        n185 = call "4155C Transfer-FPP v3.0.vi"("VISA resource name in"=w753, "FPP - Source"=w716, "Gate"=w750, "Drain"=w751, "FPP - Drain"=w714, "Timings"=w782, "error in (no error)"=w754, "FPP - Gate"=w715, "FPP - Probe 1"=w712, "sweep mode"=w775, "FPP - Probe 2"=w713, "Panel Controls"=w798) -> ("VG"=w708:dbl[], "Outparams"=w745:T9, "VISA Resource Name out"=w781:refnum<visa-resource-name>, "Vprobe2"=w742:dbl[], "ID"=w705:dbl[], "IG"=w704:dbl[], "Vprobe1"=w741:dbl[], "error out"=w707:errorcluster)  [unwired: 8 in]
        n186 = Unbundle By Name(w745) -> ("V2 Step"=w744:dbl, "V2 Start"=w743:dbl, "Number of points"=w702:i32)
        n187 = call "4155C Config Chart Colours.vi"("Numeric"=w702, "XY Graph 2"=w703) -> ()  [unwired: 6 in]
        n188 = call "4155C Split array.vi"("Number of VAR2 steps"=w702, "Y2 data in"=w705, "X data in"=w708, "Y1 data in"=w705, "Y3 data in"=w704, "error in (no error)"=w707) -> ("Array of clusters"=w709:cluster{"Y data in":dbl[], "X data in":dbl[]}[], "error out"=w706:errorcluster)  [unwired: 1 in]
        n189 = local write "I vs Vg"(w709) -> ()
        n190 = Open/Create/Replace File(file path (use dialog)=w785, error in=w706, operation (0:open)=w740) -> (refnum out=w795:refnum<file>, error out=w796:errorcluster)  [unwired: 3 in, 1 out]
        n191 = call "4155C Make Big 2d array FPP.vi"("1D Var1"=w708, "1d ID"=w705, "1d Vp2"=w742, "1d IG"=w704, "1d Vp1"=w741, "VAR2 START"=w743, "Number of VAR2 steps"=w702, "VAR2 STEP"=w744, "VAR1 Name"="Vg", "Decimal places in header"=i8 1, "VAR2 Name"="Vd") -> ("Header array"=w791:string[], "Data array"=w792:dbl[][])  [unwired: 15 in]
        n192 = call "4155C Write array to file.vi"("Byte Stream File Refnum"=w795, "Header"=w791, "Data Array"=w792, "error in (no error)"=w796) -> ("dup refnum"=w793:refnum<file>, "error out"=w794:errorcluster)  [unwired: 1 in]
        n193 = Close File(refnum=w793, error in=w794) -> (error out=w780:errorcluster)  [unwired: 1 out]
      }
      frame "output" {
        n194 = local read "Transfer/Output - Drain"() -> (w806:u32)
        n195 = local read "Transfer/Output - Source/Common"() -> (w805:u32)
        n196 = local read "Transfer/Output - Gate"() -> (w807:u32)
        n197 = Delete From Array(array=w905, index=0 ("Index")) -> (deleted portion=w903:string, array with subset deleted=w902:string[])  [unwired: 1 in]
        n198 = Bundle By Name(cluster=w818, "Emergency Stop"=w914) -> (w868:T1)
        n199 = Number To Decimal String(number=w864) -> (decimal integer string=w863:string)  [unwired: 1 in]
        n200 = case shown="\"d\", Default" w903 {
          tunnel: [w999 w1000] -> w901
          frame "s" {
            w999 = u16 0 items=["Single", "Double"] ("sweep mode")
          }
          frame "d", Default {
            w1000 = u16 1 items=["Single", "Double"] ("sweep mode")
          }
        }
        n201 = Fract/Exp String To Number(string=w902) -> (number=w887:dbl[])  [unwired: 3 in, 1 out]
        n202 = Concatenate Strings(w912, "-output-" ("Substring"), w863, w861, ".txt" ("Suffix (transfer)")) -> (w913:string)
        n203 = VISA Write(VISA resource name=w883, write buffer=":PAGE:CHAN:MODE SWE;" ("write buffer (\"\")"), error in (no error)=w882) -> (VISA resource name out=w880:refnum<visa-resource-name>, error out=w881:errorcluster)  [unwired: 1 out]
        n204 = String To Path(string=w913) -> (path=w911:path)
        n205 = Index Array(array=w887, index #1=0 ("Index")) -> (element #1=w900:dbl, element #2=w899:dbl, element #3=w898:dbl)  [unwired: 2 in]
        n206 = Delete From Array(array=w887, length=3 ("Length"), index=0 ("Index")) -> (array with subset deleted=w885:dbl[])  [unwired: 1 out]
        n207 = local read "Plot output curve extrema vs time"() -> (w815:bool)
        n208 = local read "Transfer/Output - Probe 4"() -> (w808:u32)
        n209 = Bundle By Name(cluster=w892, "Gate Start"=w900, "Gate Stop"=w899, "Gate Step (linear only)"=w898, "Gate Compliance"=w909, "Range mode"=w876, "Range"=w875) -> (w877:T6)
        n210 = case shown="True" w815 {
          tunnel: w860 -> [w916 w919]
          tunnel: w857 -> [_ w918]
          tunnel: [w916 w917] -> w834
          frame False {
          }
          frame True {
            n211 = Build Array (concatenate)(w919, w918) -> (w917:i32[])
          }
        }
        n212 = Index Array(array=w885, index #1=0 ("Index")) -> (element #1=w895:dbl, element #2=w894:dbl, element #3=w893:dbl)  [unwired: 2 in]
        n213 = call <vilib>:"compatOverwrite.vi"("overwrite (F)"=TRUE) -> ("overwrite?"=w867:T8)
        n214 = Bundle By Name(cluster=w891, "Drain Start"=w895, "Drain Stop"=w894, "Drain Step"=w893, "Drain Compliance"=w910, "Range mode"=w874, "Range"=w873) -> (w878:T7)
        n215 = call "4155C Output v3.0.vi"("VISA resource name in"=w880, "Source/Common"=w805, 2:"Gate"=w877, 3:"Drain"=w878, 4:"Drain"=w806, "Timings"=w908, "error in (no error)"=w881, 7:"Probe 4"=w814, 8:"Gate"=w807, 9:"Probe 4"=w808, "sweep mode"=w901, "Panel controls"=w868, "Standby"=w809) -> ("VD"=w866:dbl[], "Outparams"=w872:T9, "VISA Resource Name out"=w907:refnum<visa-resource-name>, "IS"=w844:dbl[], "ID"=w845:dbl[], "IG"=w843:dbl[], "error out"=w858:errorcluster, "Probe 4"=w869:dbl[])  [unwired: 7 in]
        n216 = Unbundle By Name(w872) -> ("V2 Step"=w871:dbl, "V2 Start"=w870:dbl, "Number of points"=w832:i32)
        n217 = call "4155C Split array.vi"("Number of VAR2 steps"=w832, "Y2 data in"=w845, "X data in"=w866, "Y1 data in"=w844, "Y3 data in"=w843, "error in (no error)"=w858) -> ("Array of clusters"=w859:cluster{"Y data in":dbl[], "X data in":dbl[]}[], "error out"=w820:errorcluster)  [unwired: 1 in]
        n218 = case shown="True" "Plot output curve extrema vs time" {
          tunnel: w865 -> [w928 w998]
          tunnel: w856 -> [w929 w993]
          tunnel: w847 -> [w923 w989]
          tunnel: w846 -> [w922 w988]
          tunnel: w845 -> [_ w985]
          tunnel: w844 -> [_ w983]
          tunnel: w843 -> [_ w982]
          tunnel: w842 -> [w930 w978]
          tunnel: w841 -> [w931 w977]
          tunnel: w840 -> [w926 w974]
          tunnel: w839 -> [w927 w973]
          tunnel: w838 -> [w924 w970]
          tunnel: w837 -> [w925 w969]
          tunnel: w836 -> [w920 w966]
          tunnel: w835 -> [w921 w965]
          tunnel: w834 -> [_ w958]
          tunnel: [w926 w953] -> w833
          tunnel: w832 -> [_ w952]
          tunnel: [w927 w951] -> w831
          tunnel: [w928 w950] -> w830
          tunnel: [w929 w949] -> w829
          tunnel: [w930 w948] -> w828
          tunnel: [w931 w947] -> w827
          tunnel: [w920 w946] -> w826
          tunnel: [w921 w945] -> w825
          tunnel: [w922 w944] -> w824
          tunnel: [w923 w943] -> w823
          tunnel: [w924 w942] -> w822
          tunnel: [w925 w941] -> w821
          tunnel: w820 -> [w932 w940]
          tunnel: [w932 w936] -> w819
          frame False {
          }
          frame True {
            # "Adjusts graph colors."
            # "Adjusts graph colors."
            # "Ion will be the middle element of the array. The calculation of the index is done only once, since Is, Id, and Ig have the same dimensions."
            # "abs(Ig)"
            # "abs(Is)"
            # "Y1: Is\nY2: Id\nY3: Ig"
            # "abs(Id)"
            # "Adjusts graph colors."
            # "Adjusts graph colors."
            # "Adjusts graph colors."
            n219 = Absolute Value(x=w983) -> (abs(x)=w968:dbl[])
            n220 = Absolute Value(x=w985) -> (abs(x)=w984:dbl[])
            n221 = Absolute Value(x=w982) -> (abs(x)=w971:dbl[])
            n222 = Array Size(array=w984) -> (size(s)=w992:i32)
            n223 = Divide(x=w992, y=2) -> (x/y=w935:dbl)
            n224 = Subtract(x=w935, y=1) -> (x-y=w934:dbl)
            n225 = Array Max & Min(array=w968) -> (max value=w975:dbl, min value=w976:dbl)  [unwired: 2 out]
            n226 = Array Max & Min(array=w984) -> (max value=w997:dbl, min value=w981:dbl)  [unwired: 2 out]
            n227 = Array Max & Min(array=w971) -> (max value=w980:dbl, min value=w979:dbl)  [unwired: 2 out]
            n228 = Index Array(array=w968, index=w934) -> (element=w959:dbl)
            n229 = Index Array(array=w968, index=0) -> (element=w960:dbl)
            n230 = Index Array(array=w984, index=w934) -> (element=w961:dbl)
            n231 = Index Array(array=w984, index=0) -> (element=w962:dbl)
            n232 = Index Array(array=w971, index=w934) -> (element=w964:dbl)
            n233 = Index Array(array=w971, index=0) -> (element=w963:dbl)
            n234 = local write "Ig max"(w980) -> ()
            n235 = local write "Ig min"(w979) -> ()
            n236 = local write "Is max"(w975) -> ()
            n237 = local write "Is min"(w976) -> ()
            n238 = local write "Id max"(w997) -> ()
            n239 = local write "Id min"(w981) -> ()
            n240 = Build Array (concatenate)(w974, w975) -> (w953:dbl[])
            n241 = Build Array (concatenate)(w973, w976) -> (w951:dbl[])
            n242 = local write "Is off"(w960) -> ()
            n243 = local write "Is on"(w959) -> ()
            n244 = Build Array (concatenate)(w998, w997) -> (w950:dbl[])
            n245 = Build Array (concatenate)(w993, w981) -> (w949:dbl[])
            n246 = Build Array (concatenate)(w978, w980) -> (w948:dbl[])
            n247 = Build Array (concatenate)(w977, w979) -> (w947:dbl[])
            n248 = Build Array (concatenate)(w966, w959) -> (w946:dbl[])
            n249 = Build Array (concatenate)(w965, w960) -> (w945:dbl[])
            n250 = Build Array (concatenate)(w988, w961) -> (w944:dbl[])
            n251 = Build Array (concatenate)(w989, w962) -> (w943:dbl[])
            n252 = Build Array (concatenate)(w970, w964) -> (w942:dbl[])
            n253 = Build Array (concatenate)(w969, w963) -> (w941:dbl[])
            n254 = local write "Ig off"(w963) -> ()
            n255 = local write "Ig on"(w964) -> ()
            n256 = local write "Id off"(w962) -> ()
            n257 = local write "Id on"(w961) -> ()
            n258 = control-ref of="Imax vs time"() -> (w987:refnum<vi>)
            n259 = control-ref of="Imin vs time"() -> (w986:refnum<vi>)
            n260 = control-ref of="Ion vs time"() -> (w955:refnum<vi>)
            n261 = control-ref of="Ioff vs time"() -> (w954:refnum<vi>)
            n262 = control-ref of="I vs Vg"() -> (w996:refnum<vi>)
            n263 = call "4155C Split array.vi"("Number of VAR2 steps"=w952, "Y2 data in"=w944, "X data in"=w958, "Y1 data in"=w946, "Y3 data in"=w942, "error in (no error)"=w940) -> ("Array of clusters"=w956:cluster{"Y data in":dbl[], "X data in":dbl[]}[], "error out"=w939:errorcluster)  [unwired: 1 in]
            n264 = call "4155C Split array.vi"("Number of VAR2 steps"=w952, "Y2 data in"=w943, "X data in"=w958, "Y1 data in"=w945, "Y3 data in"=w941, "error in (no error)"=w939) -> ("Array of clusters"=w957:cluster{"Y data in":dbl[], "X data in":dbl[]}[], "error out"=w938:errorcluster)  [unwired: 1 in]
            n265 = call "4155C Split array.vi"("Number of VAR2 steps"=w952, "Y2 data in"=w950, "X data in"=w958, "Y1 data in"=w953, "Y3 data in"=w948, "error in (no error)"=w938) -> ("Array of clusters"=w995:cluster{"Y data in":dbl[], "X data in":dbl[]}[], "error out"=w937:errorcluster)  [unwired: 1 in]
            n266 = call "4155C Split array.vi"("Number of VAR2 steps"=w952, "Y2 data in"=w949, "X data in"=w958, "Y1 data in"=w951, "Y3 data in"=w947, "error in (no error)"=w937) -> ("Array of clusters"=w994:cluster{"Y data in":dbl[], "X data in":dbl[]}[], "error out"=w936:errorcluster)  [unwired: 1 in]
            n267 = call "4155C Config Chart Colours.vi"("Numeric"=w952, "XY Graph 2"=w987) -> ()  [unwired: 6 in]
            n268 = call "4155C Config Chart Colours.vi"("Numeric"=w952, "XY Graph 2"=w986) -> ()  [unwired: 6 in]
            n269 = call "4155C Config Chart Colours.vi"("Numeric"=w952, "XY Graph 2"=w955) -> ()  [unwired: 6 in]
            n270 = call "4155C Config Chart Colours.vi"("Numeric"=w952, "XY Graph 2"=w954) -> ()  [unwired: 6 in]
            n271 = call "4155C Config Chart Colours.vi"("Numeric"=w952, "XY Graph 2"=w996) -> ()  [unwired: 6 in]
            n272 = local write "Imax vs time"(w995) -> ()
            n273 = local write "Imin vs time"(w994) -> ()
            n274 = local write "Ion vs time"(w956) -> ()
            n275 = local write "Ioff vs time"(w957) -> ()
          }
        }
        n276 = local write "I vs Vd"(w859) -> ()
        n277 = Open/Create/Replace File(file path (use dialog)=w911, error in=w819, operation (0:open)=w867) -> (refnum out=w854:refnum<file>, error out=w852:errorcluster)  [unwired: 3 in, 1 out]
        n278 = call "4155C Make Big 2d array.vi"("1D Var1"=w866, "1d IS"=w844, "1d ID"=w845, "1d IG"=w843, "1d SMU4"=w869, "SMU4"=w814, "VAR2 START"=w870, "Number of VAR2 steps"=w832, "VAR2 STEP"=w871, "VAR1 Name"="Vd", "Decimal places in header"=i8 1, "VAR2 Name"="Vg") -> ("Header array"=w855:string[], "Data array"=w853:dbl[][])  [unwired: 14 in]
        n279 = call "4155C Write array to file.vi"("Byte Stream File Refnum"=w854, "Header"=w855, "Data Array"=w853, "error in (no error)"=w852) -> ("dup refnum"=w851:refnum<file>, "error out"=w850:errorcluster)  [unwired: 1 in]
        n280 = Close File(refnum=w851, error in=w850) -> (error out=w906:errorcluster)  [unwired: 1 out]
      }
      frame "output-fpp" {
        # "Adjusts graph colors."
        # "Adjusts graph colors."
        # "Y1 = Vp2\nY2 = Y3 = Vp1"
        n281 = local read "FPP - Source"() -> (w1019:u32)
        n282 = local read "FPP - Drain"() -> (w1020:u32)
        n283 = local read "FPP - Gate"() -> (w1021:u32)
        n284 = Number To Decimal String(number=w1041) -> (decimal integer string=w1088:string)  [unwired: 1 in]
        n285 = Bundle By Name(cluster=w1065, "Emergency Stop"=w1091) -> (w1101:T1)
        n286 = Delete From Array(array=w1080, index=0 ("Index")) -> (deleted portion=w1078:string, array with subset deleted=w1077:string[])  [unwired: 1 in]
        n287 = VISA Write(VISA resource name=w1056, write buffer=":PAGE:CHAN:MODE SWE;" ("write buffer (\"\")"), error in (no error)=w1053) -> (VISA resource name out=w1055:refnum<visa-resource-name>, error out=w1054:errorcluster)  [unwired: 1 out]
        n288 = Concatenate Strings(w1087, "-outputfpp-" ("Substring"), w1088, w1040, ".txt" ("Substring")) -> (w1090:string)
        n289 = case shown="\"d\", Default" w1078 {
          tunnel: [w1102 w1103] -> w1076
          frame "s" {
            w1102 = u16 0 items=["Single", "Double"] ("sweep mode")
          }
          frame "d", Default {
            w1103 = u16 1 items=["Single", "Double"] ("sweep mode")
          }
        }
        n290 = Fract/Exp String To Number(string=w1077) -> (number=w1059:dbl[])  [unwired: 3 in, 1 out]
        n291 = String To Path(string=w1090) -> (path=w1086:path)
        n292 = Index Array(array=w1059, index #1=0 ("Index")) -> (element #1=w1075:dbl, element #2=w1074:dbl, element #3=w1073:dbl)  [unwired: 2 in]
        n293 = Delete From Array(array=w1059, length=3 ("Length"), index=0 ("Index")) -> (array with subset deleted=w1058:dbl[])  [unwired: 1 out]
        n294 = local read "FPP - Probe 1"() -> (w1017:u32)
        n295 = local read "FPP - Probe 2"() -> (w1018:u32)
        n296 = control-ref of="I vs Vd"() -> (w1005:refnum<vi>)
        n297 = control-ref of="Vp vs Vg (FPP)"() -> (w1004:refnum<vi>)
        n298 = Bundle By Name(cluster=w1067, "Gate Start"=w1075, "Gate Stop"=w1074, "Gate Step (linear only)"=w1073, "Gate Compliance"=w1084, "Range mode"=w1051, "Range"=w1050) -> (w1100:T6)
        n299 = Index Array(array=w1058, index #1=0 ("Index")) -> (element #1=w1070:dbl, element #2=w1069:dbl, element #3=w1068:dbl)  [unwired: 2 in]
        n300 = call <vilib>:"compatOverwrite.vi"("overwrite (F)"=TRUE) -> ("overwrite?"=w1045:T8)
        n301 = Bundle By Name(cluster=w1066, "Drain Start"=w1070, "Drain Stop"=w1069, "Drain Step"=w1068, "Drain Compliance"=w1085, "Range mode"=w1049, "Range"=w1052) -> (w1099:T7)
        n302 = call "4155C Output-FPP v3.0.vi"("VISA resource name in"=w1055, "FPP - Source"=w1019, "Gate"=w1100, "Drain"=w1099, "FPP - Drain"=w1020, "Timings"=w1083, "error in (no error)"=w1054, "FPP - Gate"=w1021, "FPP - Probe 1"=w1017, "sweep mode"=w1076, "FPP - Probe 2"=w1018, "Panel controls"=w1101) -> ("VD"=w1008:dbl[], "Outparams"=w1047:T9, "VISA Resource Name out"=w1082:refnum<visa-resource-name>, "Vprobe2"=w1007:dbl[], "ID"=w1011:dbl[], "IG"=w1010:dbl[], "Vprobe1"=w1006:dbl[], "error out"=w1012:errorcluster)  [unwired: 8 in]
        n303 = Unbundle By Name(w1047) -> ("V2 Step"=w1048:dbl, "V2 Start"=w1046:dbl, "Number of points"=w1003:i32)
        n304 = call "4155C Split array.vi"("Number of VAR2 steps"=w1003, "Y2 data in"=w1011, "X data in"=w1008, "Y1 data in"=w1011, "Y3 data in"=w1010, "error in (no error)"=w1012) -> ("Array of clusters"=w1014:cluster{"Y data in":dbl[], "X data in":dbl[]}[], "error out"=w1013:errorcluster)  [unwired: 1 in]
        n305 = call "4155C Split array.vi"("Number of VAR2 steps"=w1003, "Y2 data in"=w1006, "X data in"=w1008, "Y1 data in"=w1007, "Y3 data in"=w1006) -> ("Array of clusters"=w1009:cluster{"Y data in":dbl[], "X data in":dbl[]}[])  [unwired: 2 in, 1 out]
        n306 = call "4155C Config Chart Colours.vi"("Numeric"=w1003, "XY Graph 2"=w1005) -> ()  [unwired: 6 in]
        n307 = local write "I vs Vd"(w1014) -> ()
        n308 = call "4155C Config Chart Colours.vi"("Numeric"=w1003, "XY Graph 2"=w1004) -> ()  [unwired: 6 in]
        n309 = local write "Vp vs Vg (FPP)"(w1009) -> ()
        n310 = Open/Create/Replace File(file path (use dialog)=w1086, error in=w1013, operation (0:open)=w1045) -> (refnum out=w1096:refnum<file>, error out=w1097:errorcluster)  [unwired: 3 in, 1 out]
        n311 = call "4155C Make Big 2d array FPP.vi"("1D Var1"=w1008, "1d ID"=w1011, "1d Vp2"=w1007, "1d IG"=w1010, "1d Vp1"=w1006, "VAR2 START"=w1046, "Number of VAR2 steps"=w1003, "VAR2 STEP"=w1048, "VAR1 Name"="Vd", "Decimal places in header"=i8 1, "VAR2 Name"="Vg") -> ("Header array"=w1092:string[], "Data array"=w1093:dbl[][])  [unwired: 15 in]
        n312 = call "4155C Write array to file.vi"("Byte Stream File Refnum"=w1096, "Header"=w1092, "Data Array"=w1093, "error in (no error)"=w1097) -> ("dup refnum"=w1094:refnum<file>, "error out"=w1095:errorcluster)  [unwired: 1 in]
        n313 = Close File(refnum=w1094, error in=w1095) -> (error out=w1081:errorcluster)  [unwired: 1 out]
      }
      frame "itime" {
        n314 = Delete From Array(array=w1115, index=1) -> (deleted portion=w1114:string)  [unwired: 1 in, 1 out]
        n315 = Delete From Array(array=w1115, index=0 ("Index")) -> (deleted portion=w1143:string)  [unwired: 1 in, 1 out]
        n316 = Fract/Exp String To Number(string=w1114) -> (number=w1113:dbl)  [unwired: 3 in, 1 out]
        n317 = case shown="\"l\"" w1143 {
          tunnel: w1142 -> [w1148 w1150 w1154]
          tunnel: [w1147 w1149 w1153] -> w1135
          tunnel: w1113 -> [w1145 _ w1152]
          frame "s" {
            w1146 = u32 0 items=["short  ", "medium  ", "long  "] ("integration time 2")
            n318 = Bundle By Name(cluster=w1148, "integration time"=w1146, "Short/Long integration time"=w1145) -> (w1147:T4)
          }
          frame "m", Default {
            w1151 = u32 1 items=["short  ", "medium  ", "long  "] ("integration time 2")
            n319 = Bundle By Name(cluster=w1150, "integration time"=w1151) -> (w1149:T4)
          }
          frame "l" {
            w1155 = u32 2 items=["short  ", "medium  ", "long  "] ("integration time 2")
            n320 = Bundle By Name(cluster=w1154, "integration time"=w1155, "Short/Long integration time"=w1152) -> (w1153:T4)
          }
        }
      }
      frame "pulsed" {
        n321 = Delete From Array(array=w1192, index=0 ("Index")) -> (deleted portion=w1193:string, array with subset deleted=w1180:string[])  [unwired: 1 in]
        n322 = case shown="\"on\", Default" w1193 {
          tunnel: w1191 -> [w1203 w1206]
          tunnel: [w1202 w1205] -> w1184
          tunnel: w1180 -> [w1200 _]
          frame "on", Default {
            w1201 = u16 1 items=["Continuous", "Pulsed"] ("sweep method")
            n323 = Fract/Exp String To Number(string=w1200) -> (number=w1198:dbl[])  [unwired: 3 in, 1 out]
            n324 = Index Array(array=w1198, index #1=0 ("Index")) -> (element #1=w1197:dbl, element #2=w1196:dbl, element #3=w1195:dbl)  [unwired: 2 in]
            n325 = Bundle By Name(cluster=w1203, "sweep method"=w1201, "Pulse period"=w1197, "Base voltage"=w1196, "Pulse width"=w1195) -> (w1202:T4)
          }
          frame "off" {
            w1204 = u16 0 items=["Continuous", "Pulsed"] ("sweep method")
            n326 = Bundle By Name(cluster=w1206, "sweep method"=w1204) -> (w1205:T4)
          }
        }
      }
      frame "gaterangemode" {
        n327 = Delete From Array(array=w1241, index=0 ("Index")) -> (deleted portion=w1242:string)  [unwired: 1 in, 1 out]
        n328 = case shown="\"f\"" w1242 {
          tunnel: [w1244 w1245 w1246] -> w1231
          frame "a", Default {
            w1244 = u16 0 items=["Auto", "Limited", "Fixed"] ("Gate Range\nmode 2")
          }
          frame "f" {
            w1245 = u16 2 items=["Auto", "Limited", "Fixed"] ("Gate Range\nmode 2")
          }
          frame "l" {
            w1246 = u16 1 items=["Auto", "Limited", "Fixed"] ("Gate Range\nmode 2")
          }
        }
      }
      frame "gaterange" {
        (unwired) u8 11 items=["10fA  ", "100fA  ", "1nA  ", "10nA", "100nA", "1uA", "10uA", "100uA", "1mA", "10mA", "100mA", "1A"] ("Gate Range 2")
        n329 = Delete From Array(array=w1288, index=0 ("Index")) -> (deleted portion=w1278:string)  [unwired: 1 in, 1 out]
        n330 = Scan Value(string=w1278, format string="") -> (value=w1276:dbl)  [unwired: 1 in, 1 out]
        n331 = Logarithm Base 10(1:w1276) -> (0:w1275:dbl)
        n332 = Round To Nearest(number=w1275) -> (nearest integer value=w1274:dbl)
        n333 = Add(x=w1274, y=11.0) -> (x+y=w1272:dbl)
        n334 = To Unsigned Byte Integer(number=w1272) -> (unsigned 8bit integer=w1271:u8)
      }
      frame "drainrange" {
        (unwired) u8 11 items=["10fA  ", "100fA  ", "1nA  ", "10nA", "100nA", "1uA", "10uA", "100uA", "1mA", "10mA", "100mA", "1A"] ("Gate Range 2")
        n335 = Delete From Array(array=w1331, index=0 ("Index")) -> (deleted portion=w1322:string)  [unwired: 1 in, 1 out]
        n336 = Scan Value(string=w1322, format string="") -> (value=w1320:dbl)  [unwired: 1 in, 1 out]
        n337 = Logarithm Base 10(1:w1320) -> (0:w1319:dbl)
        n338 = Round To Nearest(number=w1319) -> (nearest integer value=w1318:dbl)
        n339 = Add(x=w1318, y=11.0) -> (x+y=w1316:dbl)
        n340 = To Unsigned Byte Integer(number=w1316) -> (unsigned 8bit integer=w1315:u8)
      }
      frame "drainrangemode" {
        n341 = Delete From Array(array=w1367, index=0 ("Index")) -> (deleted portion=w1368:string)  [unwired: 1 in, 1 out]
        n342 = case shown="\"f\"" w1368 {
          tunnel: [w1370 w1371 w1372] -> w1357
          frame "a", Default {
            w1370 = u16 0 items=["Auto", "Limited", "Fixed"] ("Gate Range\nmode 2")
          }
          frame "f" {
            w1371 = u16 2 items=["Auto", "Limited", "Fixed"] ("Gate Range\nmode 2")
          }
          frame "l" {
            w1372 = u16 1 items=["Auto", "Limited", "Fixed"] ("Gate Range\nmode 2")
          }
        }
      }
      frame "Error", Default {
      }
      frame "logfile" {
        n343 = Number To Decimal String(number=w1431) -> (decimal integer string=w1466:string)  [unwired: 1 in]
        n344 = Concatenate Strings(w1465, "logfile" ("Substring"), w1466, w1429, ".txt" ("Substring")) -> (w1463:string)
        n345 = String To Path(string=w1463) -> (path=w1436:path)
        n346 = Unbundle(w1462) -> ("integration time"=w1461:u32, "Short/Long integration time"=w1460:dbl, "hold time (sec)"=w1459:dbl, "delay time (sec)"=w1458:dbl, "Step Time (0 disables)"=w1457:dbl, "sweep method"=w1456:u16, "Pulse period"=w1455:dbl, "Base voltage"=w1454:dbl, "Pulse width"=w1453:dbl)
        n347 = Build Array(w1461, w1460, w1459, w1458, w1457, w1456, w1455, w1454, w1453, w1447, w1448, w1449, w1450, w1451, w1452) -> (w1440:dbl[])
        n348 = Insert Into Array(array=dbl[][] [] ("Input Array"), new element=w1440) -> (w1439:dbl[][])  [unwired: 2 in]
        n349 = call <vilib>:"compatOverwrite.vi"("overwrite (F)"=TRUE) -> ("overwrite?"=w1434:T8)
        n350 = Open/Create/Replace File(file path (use dialog)=w1436, error in=w1438, operation (0:open)=w1434) -> (refnum out=w1444:refnum<file>, error out=w1443:errorcluster)  [unwired: 3 in, 1 out]
        n351 = call "4155C Write array to file.vi"("Byte Stream File Refnum"=w1444, "Header"=string[] ["Int Time", "Short/Long Itime", "Hold time", "Delay time", "Step time", "Sweep method", "Pulse period", "Base Voltage", "Pulse width", "Drain compliance", "Gate compliance", "Gate range mode", "Gate range", "S/D range mode", "S/D range"], "Data Array"=w1439, "error in (no error)"=w1443) -> ("dup refnum"=w1446:refnum<file>, "error out"=w1445:errorcluster)  [unwired: 1 in]
        n352 = Close File(refnum=w1446, error in=w1445) -> (error out=w1437:errorcluster)  [unwired: 1 out]
      }
      frame "sample" {
        w1494 = 1
        # "Add a time offset (elapsed time) to the time axis."
        # "Adjusts graph colors."
        n353 = Number To Decimal String(number=w1526) -> (decimal integer string=w1568:string)  [unwired: 1 in]
        n354 = Fract/Exp String To Number(string=w1565) -> (number=w1530:dbl[])  [unwired: 3 in, 1 out]
        n355 = local read "Sample - Probe 4"() -> (w1476:u32)
        n356 = Concatenate Strings(w1546, "-sample-" ("Substring"), w1568, w1524, ".txt" ("Substring")) -> (w1566:string)
        n357 = local read "Sample - Drain"() -> (w1477:u32)
        n358 = Index Array(array=w1530, index=0 ("Index")) -> (element=w1563:dbl)
        n359 = String To Path(string=w1566) -> (path=w1550:path)
        n360 = Index Array(array=w1530, index=2 ("Index")) -> (element=w1559:dbl)
        n361 = Index Array(array=w1530, index=3 ("Index")) -> (element=w1532:dbl)
        n362 = Index Array(array=w1530, index=4 ("Index")) -> (element=w1529:dbl)
        n363 = Index Array(array=w1530, index=1 ("Index")) -> (element=w1560:dbl)
        n364 = local read "Plot sample extrema vs time"() -> (w1497:bool)
        n365 = local read "Time Units"() -> (w1472:u16)
        n366 = local read "Sample - Gate"() -> (w1479:u32)
        n367 = local read "Sample - Source/Common"() -> (w1478:u32)
        n368 = call "4155C Config Sampling Measurements v3.0.vi"("VISA session"=w1571, "Num Points"=w1559, "Sample - Drain"=w1477, "Display on/off"=TRUE, "Gate Compliance"=w1547, "Sampling interval"=w1529, "Sample - Source/Common"=w1478, "Sample - Probe 4"=w1476, "Drain Compliance"=w1569, "Standby"=w1480, "error in (no error)"=w1570, "Timings"=w1538, "Sample - Gate"=w1479, "Sample time"=w1532) -> ("dup VISA resource name"=w1573:refnum<visa-resource-name>, "error out"=w1572:errorcluster)
        n369 = call "4155C Take Sample v3.0.vi"("VISA resource name in"=w1573, "Emergency Stop"=w1543, "Sample - Gate"=w1479, "Vg"=w1563, "Sample - Drain"=w1477, "Vd"=w1560, "error in (no error)"=w1572) -> ("Time"=w1474:dbl[], "VISA Resource Name out"=w1540:refnum<visa-resource-name>, "Ig"=w1490:dbl[], "Id"=w1491:dbl[], "Is"=w1492:dbl[], "error out"=w1495:errorcluster)  [unwired: 3 in]
        n370 = case shown="0, Default" w1472 {
          tunnel: [w1576 w1577 w1580] -> w1475
          tunnel: w1474 -> [w1575 w1577 w1579]
          frame 2 {
            n371 = Divide(x=w1575, y=3600.0) -> (x/y=w1576:dbl[])
          }
          frame 0, Default {
          }
          frame 1 {
            n372 = Divide(x=w1579, y=60.0) -> (x/y=w1580:dbl[])
          }
        }
        n373 = Insert Into Array(array=w1488, new element=w1491) -> (w1482:dbl[])  [unwired: 1 in]
        n374 = Add(x=w1475, y=w1473) -> (x+y=w1493:dbl[])
        n375 = Insert Into Array(array=w1487, new element=w1492) -> (w1483:dbl[])  [unwired: 1 in]
        n376 = Insert Into Array(array=w1489, new element=w1490) -> (w1485:dbl[])  [unwired: 1 in]
        n377 = case shown="True" w1497 {
          tunnel: w1498 -> [w1581 w1583]
          tunnel: [w1581 w1584] -> w1496
          tunnel: w1493 -> [_ w1582]
          frame False {
          }
          frame True {
            n378 = Insert Into Array(array=w1583, new element=w1582) -> (w1584:i32[])  [unwired: 1 in]
          }
        }
        n379 = case shown="True" "Plot sample extrema vs time" {
          tunnel: w1492 -> [_ w1612]
          tunnel: w1491 -> [_ w1613]
          tunnel: w1490 -> [_ w1614]
          tunnel: [w1591 w1601] -> w1481
          tunnel: w1495 -> [w1591 w1605]
          tunnel: w1519 -> [w1590 w1617]
          tunnel: w1518 -> [w1589 w1616]
          tunnel: w1517 -> [w1588 w1618]
          tunnel: w1516 -> [w1587 w1615]
          tunnel: w1515 -> [w1586 w1620]
          tunnel: w1514 -> [w1585 w1619]
          tunnel: [w1590 w1603] -> w1513
          tunnel: [w1589 w1596] -> w1512
          tunnel: [w1588 w1597] -> w1511
          tunnel: [w1587 w1621] -> w1510
          tunnel: [w1586 w1604] -> w1509
          tunnel: [w1585 w1598] -> w1508
          tunnel: w1496 -> [_ w1592]
          frame False {
          }
          frame True {
            w1599 = 1
            # "Number of VAR2 steps is 1."
            # "abs(Ig)"
            # "abs(Is)"
            # "abs(Id)"
            # "Adjusts graph colors."
            n380 = Absolute Value(x=w1614) -> (abs(x)=w1593:dbl[])
            n381 = Absolute Value(x=w1613) -> (abs(x)=w1594:dbl[])
            n382 = Absolute Value(x=w1612) -> (abs(x)=w1595:dbl[])
            n383 = Array Max & Min(array=w1595) -> (max value=w1611:dbl, min value=w1608:dbl)  [unwired: 2 out]
            n384 = Array Max & Min(array=w1594) -> (max value=w1610:dbl, min value=w1607:dbl)  [unwired: 2 out]
            n385 = Array Max & Min(array=w1593) -> (max value=w1609:dbl, min value=w1606:dbl)  [unwired: 2 out]
            n386 = local write "Id max"(w1610) -> ()
            n387 = local write "Id min"(w1607) -> ()
            n388 = local write "Ig max"(w1609) -> ()
            n389 = local write "Ig min"(w1606) -> ()
            n390 = Insert Into Array(array=w1620, new element=w1593) -> (w1604:dbl[])  [unwired: 1 in]
            n391 = Insert Into Array(array=w1619, new element=w1593) -> (w1598:dbl[])  [unwired: 1 in]
            n392 = local write "Is max"(w1611) -> ()
            n393 = local write "Is min"(w1608) -> ()
            n394 = Insert Into Array(array=w1618, new element=w1594) -> (w1597:dbl[])  [unwired: 1 in]
            n395 = Insert Into Array(array=w1615, new element=w1594) -> (w1621:dbl[])  [unwired: 1 in]
            n396 = Insert Into Array(array=w1617, new element=w1595) -> (w1603:dbl[])  [unwired: 1 in]
            n397 = Insert Into Array(array=w1616, new element=w1595) -> (w1596:dbl[])  [unwired: 1 in]
            n398 = control-ref of="Imax vs time"() -> (w1622:refnum<vi>)
            n399 = call "4155C Config Chart Colours.vi"("Numeric"=w1599, "XY Graph 2"=w1622) -> ()  [unwired: 6 in]
            n400 = call "4155C Split array.vi"("Number of VAR2 steps"=w1599, "Y2 data in"=w1597, "X data in"=w1592, "Y1 data in"=w1603, "Y3 data in"=w1604, "error in (no error)"=w1605) -> ("Array of clusters"=w1623:cluster{"Y data in":dbl[], "X data in":dbl[]}[], "error out"=w1602:errorcluster)  [unwired: 1 in]
            n401 = call "4155C Split array.vi"("Number of VAR2 steps"=w1599, "Y2 data in"=w1597, "X data in"=w1592, "Y1 data in"=w1596, "Y3 data in"=w1598, "error in (no error)"=w1602) -> ("Array of clusters"=w1600:cluster{"Y data in":dbl[], "X data in":dbl[]}[], "error out"=w1601:errorcluster)  [unwired: 1 in]
            n402 = local write "Imax vs time"(w1623) -> ()
            n403 = local write "Imin vs time"(w1600) -> ()
          }
        }
        n404 = Insert Into Array(array=w1486, new element=w1493) -> (w1484:dbl[])  [unwired: 1 in]
        n405 = control-ref of="I vs time (Bias Stress)"() -> (w1501:refnum<vi>)
        n406 = call "4155C Split array.vi"("Number of VAR2 steps"=w1494, "Y2 data in"=w1482, "X data in"=w1484, "Y1 data in"=w1483, "Y3 data in"=w1485) -> ("Array of clusters"=w1500:cluster{"Y data in":dbl[], "X data in":dbl[]}[])  [unwired: 2 in, 1 out]
        n407 = call "4155C Config Chart Colours.vi"("Numeric"=w1494, "XY Graph 2"=w1501) -> ()  [unwired: 6 in]
        n408 = local write "I vs time (Bias Stress)"(w1500) -> ()
        n409 = Insert Into Array(array=dbl[][] [] ("Input Array"), new element=w1493) -> (w1499:dbl[][])  [unwired: 2 in]
        n410 = Insert Into Array(array=w1499, new element=w1490) -> (w1553:dbl[][])  [unwired: 2 in]
        n411 = VISA Write(VISA resource name=w1540, write buffer=":DISP ON" ("write buffer (\"\")"), error in (no error)=w1481) -> (VISA resource name out=w1539:refnum<visa-resource-name>, error out=w1541:errorcluster)  [unwired: 1 out]
        n412 = Insert Into Array(array=w1553, new element=w1491) -> (w1552:dbl[][])  [unwired: 2 in]
        n413 = Insert Into Array(array=w1552, new element=w1492) -> (w1545:dbl[][])  [unwired: 2 in]
        n414 = Transpose 2D Array(2D array=w1545) -> (transposed array=w1544:dbl[][])
        n415 = call <vilib>:"compatOverwrite.vi"("overwrite (F)"=TRUE) -> ("overwrite?"=w1527:T8)
        n416 = Open/Create/Replace File(file path (use dialog)=w1550, error in=w1541, operation (0:open)=w1527) -> (refnum out=w1556:refnum<file>, error out=w1555:errorcluster)  [unwired: 3 in, 1 out]
        n417 = call "4155C Write array to file.vi"("Byte Stream File Refnum"=w1556, "Header"=string[] ["Time /Units", "Ig /A", "Id /A", "Is /A"], "Data Array"=w1544, "error in (no error)"=w1555) -> ("dup refnum"=w1558:refnum<file>, "error out"=w1557:errorcluster)  [unwired: 1 in]
        n418 = Close File(refnum=w1558, error in=w1557) -> (error out=w1548:errorcluster)  [unwired: 1 out]
      }
      frame "samplei" {
        w1636 = 1
        # "Adjusts graph colors."
        # "Add a time offset (elapsed time) to the time axis."
        n419 = local read "Sample I - Source/Common"() -> (w1648:u32)
        n420 = Number To Decimal String(number=w1671) -> (decimal integer string=w1719:string)  [unwired: 1 in]
        n421 = local read "Sample I - Probe 4 (Disabled)"() -> (w1651:u32)
        n422 = Concatenate Strings(w1700, "-samplei-" ("Substring"), w1719, w1670, ".txt" ("Substring")) -> (w1717:string)
        n423 = Fract/Exp String To Number(string=w1716) -> (number=w1685:dbl[])  [unwired: 3 in, 1 out]
        n424 = String To Path(string=w1717) -> (path=w1703:path)
        n425 = local read "Sample I - Probe 3 (Disabled)"() -> (w1650:u32)
        n426 = Index Array(array=w1685, index=4 ("Index")) -> (element=w1679:dbl)
        n427 = Index Array(array=w1685, index=3 ("Index")) -> (element=w1680:dbl)
        n428 = Index Array(array=w1685, index=1 ("Index")) -> (element=w1682:dbl)
        n429 = Index Array(array=w1685, index=0 ("Index")) -> (element=w1683:dbl)
        n430 = Index Array(array=w1685, index=2 ("Index")) -> (element=w1681:dbl)
        n431 = local read "Sample I - Drain/Gate"() -> (w1649:u32)
        n432 = call "4155C Config SamplingI Measurements v3.0.vi"("VISA session"=w1722, "Num Points"=w1682, "Sample I - Probe 3 (Disabled)"=w1650, "Display on/off"=TRUE, "Sample I - Source/Common"=w1648, "Sample I - Drain/Gate"=w1649, "Sampling interval"=w1680, "Standby"=w1652, "error in (no error)"=w1721, "Timings"=w1692, "Sample I - Probe 4 (Disabled)"=w1651, "Sample time"=w1681) -> ("dup VISA resource name"=w1724:refnum<visa-resource-name>, "error out"=w1723:errorcluster)  [unwired: 2 in]
        n433 = local read "Plot sample extrema vs time"() -> (w1645:bool)
        n434 = local read "Time Units"() -> (w1641:u16)
        n435 = call "4155C Take SampleI v3.0.vi"("Sample I - Drain/Gate"=w1649, "Emergency Stop"=w1697, "error in (no error)"=w1723, "Idg 2"=w1683, "Vdg compliance 2"=w1679, "VISA resource name in"=w1724) -> ("error out"=w1695:errorcluster, "Idg"=w1628:dbl[], "Vdg"=w1629:dbl[], "VISA Resource Name out"=w1693:refnum<visa-resource-name>, "Is"=w1625:dbl[], "Time"=w1640:dbl[])
        n436 = case shown="0, Default" w1641 {
          tunnel: [w1727 w1728 w1731] -> w1642
          tunnel: w1640 -> [w1726 w1728 w1730]
          frame 2 {
            n437 = Divide(x=w1726, y=3600.0) -> (x/y=w1727:dbl[])
          }
          frame 0, Default {
          }
          frame 1 {
            n438 = Divide(x=w1730, y=60.0) -> (x/y=w1731:dbl[])
          }
        }
        n439 = Add(x=w1642, y=w1639) -> (x+y=w1634:dbl[])
        n440 = Insert Into Array(array=w1635, new element=w1634) -> (w1633:dbl[])  [unwired: 1 in]
        n441 = case shown="True" w1645 {
          tunnel: w1644 -> [w1732 w1734]
          tunnel: [w1732 w1735] -> w1643
          tunnel: w1634 -> [_ w1733]
          frame False {
          }
          frame True {
            n442 = Insert Into Array(array=w1734, new element=w1733) -> (w1735:i32[])  [unwired: 1 in]
          }
        }
        n443 = control-ref of="Vdg vs time (Bias Stress)"() -> (w1638:refnum<vi>)
        n444 = Insert Into Array(array=dbl[][] [] ("Input Array"), new element=w1634) -> (w1707:dbl[][])  [unwired: 2 in]
        n445 = call "4155C Config Chart Colours.vi"("Numeric"=w1636, "XY Graph 2"=w1638) -> ()  [unwired: 6 in]
        n446 = Insert Into Array(array=w1632, new element=w1629) -> (w1624:dbl[])  [unwired: 1 in]
        n447 = call "4155C Split array.vi"("Number of VAR2 steps"=w1636, "X data in"=w1633, "Y1 data in"=w1624) -> ("Array of clusters"=w1637:cluster{"Y data in":dbl[], "X data in":dbl[]}[])  [unwired: 4 in, 1 out]
        n448 = local write "Vdg vs time (Bias Stress)"(w1637) -> ()
        n449 = Insert Into Array(array=w1631, new element=w1628) -> (w1630:dbl[])  [unwired: 1 in]
        n450 = Insert Into Array(array=w1707, new element=w1629) -> (w1706:dbl[][])  [unwired: 2 in]
        n451 = Insert Into Array(array=w1627, new element=w1625) -> (w1626:dbl[])  [unwired: 1 in]
        n452 = Insert Into Array(array=w1706, new element=w1628) -> (w1705:dbl[][])  [unwired: 2 in]
        n453 = VISA Write(VISA resource name=w1693, write buffer=":DISP ON" ("write buffer (\"\")"), error in (no error)=w1695) -> (VISA resource name out=w1678:refnum<visa-resource-name>, error out=w1694:errorcluster)  [unwired: 1 out]
        n454 = Insert Into Array(array=w1705, new element=w1625) -> (w1699:dbl[][])  [unwired: 2 in]
        n455 = call <vilib>:"compatOverwrite.vi"("overwrite (F)"=TRUE) -> ("overwrite?"=w1673:T8)
        n456 = Open/Create/Replace File(file path (use dialog)=w1703, error in=w1694, operation (0:open)=w1673) -> (refnum out=w1710:refnum<file>, error out=w1709:errorcluster)  [unwired: 3 in, 1 out]
        n457 = Transpose 2D Array(2D array=w1699) -> (transposed array=w1698:dbl[][])
        n458 = call "4155C Write array to file.vi"("Byte Stream File Refnum"=w1710, "Header"=string[] ["Time /s", "Vdg /V", "Idg /A", "Is /A"], "Data Array"=w1698, "error in (no error)"=w1709) -> ("dup refnum"=w1712:refnum<file>, "error out"=w1711:errorcluster)  [unwired: 1 in]
        n459 = Close File(refnum=w1712, error in=w1711) -> (error out=w1676:errorcluster)  [unwired: 1 out]
        n460 = VISA Write(VISA resource name=w1678, write buffer=";:PAGE:SCON:STAN OFF;:PAGE:CHAN:VSU2:DIS;" ("write buffer (\"\")"), error in (no error)=w1676) -> (VISA resource name out=w1674:refnum<visa-resource-name>, error out=w1675:errorcluster)  [unwired: 1 out]
      }
      frame "#" {
        n461 = VISA Write(VISA resource name=w1764, write buffer=":DISP ON" ("write buffer (\"\")"), error in (no error)=w1763) -> (VISA resource name out=w1762:refnum<visa-resource-name>, error out=w1761:errorcluster)  [unwired: 1 out]
      }
      frame "stressV" {
        n462 = Number To Decimal String(number=w1799) -> (decimal integer string=w1840:string)  [unwired: 1 in]
        n463 = Concatenate Strings(w1824, "-stressV-" ("Substring"), w1840, w1798, ".txt" ("Substring")) -> (w1838:string)
        n464 = Fract/Exp String To Number(string=w1837) -> (number=w1810:dbl[])  [unwired: 3 in, 1 out]
        n465 = local read "Stress V - Drain"() -> (w1777:u32)
        n466 = String To Path(string=w1838) -> (path=w1828:path)
        n467 = Index Array(array=w1810, index=3 ("Index")) -> (element=w1807:dbl)
        n468 = Index Array(array=w1810, index=1 ("Index")) -> (element=w1805:dbl)
        n469 = Index Array(array=w1810, index=0 ("Index")) -> (element=w1804:dbl)
        n470 = Index Array(array=w1810, index=4 ("Index")) -> (element=w1809:dbl)
        n471 = Index Array(array=w1810, index=2 ("Index")) -> (element=w1806:dbl)
        n472 = local read "Stress V - Gate"() -> (w1778:u32)
        n473 = local read "Stress V - Source/Common"() -> (w1779:u32)
        n474 = call "4155C Config V Stress v3.0.vi"("Display on/off"=TRUE, "Stress V - Gate"=w1778, "Stress V - Drain"=w1777, "Stress V - Source/Common"=w1779, "IG compliance"=w1806, "ID compliance"=w1807, "error in (no error)"=w1842, "VG"=w1804, "VD"=w1805, "VISA session"=w1843) -> ("error out"=w1844:errorcluster, "dup VISA resource name"=w1845:refnum<visa-resource-name>)
        n475 = call "4155C Apply Stress.vi"("error in (no error)"=w1844, "Duration"=w1809, "Emergency Stop"=w1823, "VISA resource name in"=w1845) -> ("error out"=w1821:errorcluster, "VISA Resource Name out"=w1819:refnum<visa-resource-name>)
        n476 = VISA Write(VISA resource name=w1819, write buffer=":DISP ON" ("write buffer (\"\")"), error in (no error)=w1821) -> (VISA resource name out=w1818:refnum<visa-resource-name>, error out=w1820:errorcluster)  [unwired: 1 out]
        n477 = call <vilib>:"compatOverwrite.vi"("overwrite (F)"=TRUE) -> ("overwrite?"=w1803:T8)
        n478 = Open/Create/Replace File(file path (use dialog)=w1828, error in=w1820, operation (0:open)=w1803) -> (refnum out=w1831:refnum<file>, error out=w1830:errorcluster)  [unwired: 3 in, 1 out]
        n479 = call "4155C Write array to file.vi"("Byte Stream File Refnum"=w1831, "Header"=string[] ["V stress completed successfully", ""], "error in (no error)"=w1830) -> ("dup refnum"=w1833:refnum<file>, "error out"=w1832:errorcluster)  [unwired: 2 in]
        n480 = Close File(refnum=w1833, error in=w1832) -> (error out=w1826:errorcluster)  [unwired: 1 out]
      }
      frame "stressI" {
        n481 = Number To Decimal String(number=w1871) -> (decimal integer string=w1908:string)  [unwired: 1 in]
        n482 = Concatenate Strings(w1892, "-stressI-" ("Substring"), w1908, w1870, ".txt" ("Substring")) -> (w1906:string)
        n483 = Fract/Exp String To Number(string=w1905) -> (number=w1880:dbl[])  [unwired: 3 in, 1 out]
        n484 = local read "Stress I - Source/Common"() -> (w1850:u32)
        n485 = Index Array(array=w1880, index=1 ("Index")) -> (element=w1876:dbl)
        n486 = Index Array(array=w1880, index=0 ("Index")) -> (element=w1877:dbl)
        n487 = Index Array(array=w1880, index=2 ("Index")) -> (element=w1878:dbl)
        n488 = String To Path(string=w1906) -> (path=w1896:path)
        n489 = local read "Stress I - Drain/Gate"() -> (w1851:u32)
        n490 = call "4155C Config I Stress v3.0.vi"("Stress I - Drain/Gate"=w1851, "Stress I - Source/Common"=w1850, "Display on/off"=TRUE, "error in (no error)"=w1910, "VDG compliance"=w1876, "IDG"=w1877, "VISA session"=w1911) -> ("error out"=w1912:errorcluster, "dup VISA resource name"=w1913:refnum<visa-resource-name>)  [unwired: 1 in]
        n491 = call "4155C Apply Stress.vi"("error in (no error)"=w1912, "Duration"=w1878, "Emergency Stop"=w1891, "VISA resource name in"=w1913) -> ("error out"=w1889:errorcluster, "VISA Resource Name out"=w1887:refnum<visa-resource-name>)
        n492 = VISA Write(VISA resource name=w1887, write buffer=":DISP ON" ("write buffer (\"\")"), error in (no error)=w1889) -> (VISA resource name out=w1886:refnum<visa-resource-name>, error out=w1888:errorcluster)  [unwired: 1 out]
        n493 = call <vilib>:"compatOverwrite.vi"("overwrite (F)"=TRUE) -> ("overwrite?"=w1875:T8)
        n494 = Open/Create/Replace File(file path (use dialog)=w1896, error in=w1888, operation (0:open)=w1875) -> (refnum out=w1899:refnum<file>, error out=w1898:errorcluster)  [unwired: 3 in, 1 out]
        n495 = call "4155C Write array to file.vi"("Byte Stream File Refnum"=w1899, "Header"=string[] ["I stress completed successfully", ""], "error in (no error)"=w1898) -> ("dup refnum"=w1901:refnum<file>, "error out"=w1900:errorcluster)  [unwired: 2 in]
        n496 = Close File(refnum=w1901, error in=w1900) -> (error out=w1894:errorcluster)  [unwired: 1 out]
      }
      frame "vsu2pulse" {
        n497 = Number To Decimal String(number=w1938) -> (decimal integer string=w1973:string)  [unwired: 1 in]
        n498 = Concatenate Strings(w1958, "-vsu2-" ("Substring"), w1973, w1937, ".txt" ("Substring")) -> (w1971:string)
        n499 = Fract/Exp String To Number(string=w1970) -> (number=w1946:dbl[])  [unwired: 3 in, 1 out]
        n500 = String To Path(string=w1971) -> (path=w1962:path)
        n501 = Index Array(array=w1946, index=1 ("Index")) -> (element=w1945:dbl)
        n502 = Index Array(array=w1946, index=0 ("Index")) -> (element=w1943:dbl)
        n503 = local read "VSU2 Stress - Source/Common"() -> (w1918:u32)
        n504 = call "4155C Config VSU2 Stress v3.0.vi"("VISA session"=w1976, "Display on/off"=TRUE, "VSU2"=w1943, "error in (no error)"=w1975, "VSU2 Stress - Source/Common"=w1918) -> ("dup VISA resource name"=w1978:refnum<visa-resource-name>, "error out"=w1977:errorcluster)
        n505 = call "4155C Apply Stress.vi"("error in (no error)"=w1977, "Duration"=w1945, "Emergency Stop"=w1957, "VISA resource name in"=w1978) -> ("error out"=w1955:errorcluster, "VISA Resource Name out"=w1953:refnum<visa-resource-name>)
        n506 = VISA Write(VISA resource name=w1953, write buffer=":DISP ON" ("write buffer (\"\")"), error in (no error)=w1955) -> (VISA resource name out=w1952:refnum<visa-resource-name>, error out=w1954:errorcluster)  [unwired: 1 out]
        n507 = call <vilib>:"compatOverwrite.vi"("overwrite (F)"=TRUE) -> ("overwrite?"=w1942:T8)
        n508 = Open/Create/Replace File(file path (use dialog)=w1962, error in=w1954, operation (0:open)=w1942) -> (refnum out=w1965:refnum<file>, error out=w1964:errorcluster)  [unwired: 3 in, 1 out]
        n509 = call "4155C Write array to file.vi"("Byte Stream File Refnum"=w1965, "Header"=string[] ["VSU2 pulse completed successfully", ""], "error in (no error)"=w1964) -> ("dup refnum"=w1967:refnum<file>, "error out"=w1966:errorcluster)  [unwired: 2 in]
        n510 = Close File(refnum=w1967, error in=w1966) -> (error out=w1960:errorcluster)  [unwired: 1 out]
      }
      frame "sample-fpp" {
        w1990 = 1
        w2048 = string[] ["Time /s", "Id VgVd /A", "Ig VgVd /A", "Vp1 VgVd /V", "Vp2 VgVd /V"] ("Header")
        w2052 = "%d" ("format string")
        # "Y1 = Y2 = ID\nY3 = IG"
        # "Y1 = Vp2\nY2 = Y3 = Vp1"
        # "Add a time offset (elapsed time) to the time axis."
        n511 = local read "FPP - Drain"() -> (w2025:u32)
        n512 = local read "FPP - Source"() -> (w2024:u32)
        n513 = local read "Plot sample extrema vs time"() -> (w1998:bool)
        n514 = Fract/Exp String To Number(string=w2091) -> (number=w2079:dbl[])  [unwired: 3 in, 1 out]
        n515 = local read "FPP - Probe 1"() -> (w2028:u32)
        n516 = Number To Decimal String(number=w2040) -> (decimal integer string=w2094:string)  [unwired: 1 in]
        n517 = local read "Plot sample extrema vs time"() -> (w2001:bool)
        n518 = Concatenate Strings(w2085, "-samplefpp-" ("Substring"), w2094, w2039, ".txt" ("Substring")) -> (w2092:string)
        n519 = local read "FPP - Gate"() -> (w2026:u32)
        n520 = local read "Time Units"() -> (w2016:u16)
        n521 = String To Path(string=w2092) -> (path=w2060:path)
        n522 = local read "FPP - Probe 2"() -> (w2027:u32)
        n523 = Index Array(array=w2079, index=0 ("Index")) -> (element=w2047:dbl)
        n524 = Index Array(array=w2079, index=1 ("Index")) -> (element=w2046:dbl)
        n525 = control-ref of="I vs time (Bias Stress)"() -> (w2018:refnum<vi>)
        n526 = Index Array(array=w2079, index=2 ("Index")) -> (element=w2087:dbl)
        n527 = Index Array(array=w2079, index=3 ("Index")) -> (element=w2077:dbl)
        n528 = call "4155C Config Sampling Measurements FPP v3.0.vi"("VISA session"=w2097, "Gate Compliance"=w2086, "FPP - Source"=w2024, "FPP - Drain"=w2025, "Drain Compliance"=w2095, "error in (no error)"=w2096, "Num Points"=w2087, "Timings"=w2084, "FPP - Gate"=w2026, "FPP - Probe 1"=w2028, "Vg"=w2047, "Vd"=w2046, "Display on/off"=TRUE, "Sample time"=w2077, "FPP - Probe 2"=w2027, "Standby"=w2029) -> ("dup VISA resource name"=w2062:refnum<visa-resource-name>, "error out"=w2061:errorcluster)  [unwired: 2 in]
        n529 = Number To Decimal String(number=w2047) -> (decimal integer string=w2068:string)  [unwired: 1 in]
        n530 = call "4155C Take Sample FPP.vi"("VISA resource name in"=w2062, "error in (no error)"=w2061, "Emergency Stop"=w2063) -> ("Time"=w2015:dbl[], "Vp1"=w1984:dbl[], "VISA Resource Name out"=w2044:refnum<visa-resource-name>, "Ig"=w1995:dbl[], "Id"=w1994:dbl[], "Vp2"=w1983:dbl[], "error out"=w1997:errorcluster)  [unwired: 10 in]
        n531 = Insert Into Array(array=w2022, new element=w1994) -> (w1981:dbl[])  [unwired: 1 in]
        n532 = Insert Into Array(array=w2023, new element=w1995) -> (w2020:dbl[])  [unwired: 1 in]
        n533 = case shown="0, Default" w2016 {
          tunnel: [w2137 w2138 w2141] -> w2017
          tunnel: w2015 -> [w2136 w2138 w2140]
          frame 2 {
            n534 = Divide(x=w2136, y=3600.0) -> (x/y=w2137:dbl[])
          }
          frame 0, Default {
          }
          frame 1 {
            n535 = Divide(x=w2140, y=60.0) -> (x/y=w2141:dbl[])
          }
        }
        n536 = Add(x=w2017, y=w2014) -> (x+y=w1988:dbl[])
        n537 = case shown="True" w1998 {
          tunnel: w2000 -> [w2098 w2100]
          tunnel: [w2098 w2101] -> w1999
          tunnel: w1988 -> [_ w2099]
          frame False {
          }
          frame True {
            n538 = Insert Into Array(array=w2100, new element=w2099) -> (w2101:i32[])  [unwired: 1 in]
          }
        }
        n539 = Insert Into Array(array=w2021, new element=w1988) -> (w1989:dbl[])  [unwired: 1 in]
        n540 = case shown="True" w2001 {
          tunnel: w1994 -> [_ w2126]
          tunnel: w1995 -> [_ w2127]
          tunnel: [w2108 w2118] -> w1996
          tunnel: w1997 -> [w2108 w2121]
          tunnel: w2013 -> [w2107 w2111]
          tunnel: w2012 -> [w2106 w2110]
          tunnel: w2011 -> [w2105 w2129]
          tunnel: w2010 -> [w2104 w2128]
          tunnel: w2009 -> [w2103 w2131]
          tunnel: w2008 -> [w2102 w2130]
          tunnel: [w2107 w2111] -> w2007
          tunnel: [w2106 w2110] -> w2006
          tunnel: [w2105 w2109] -> w2005
          tunnel: [w2104 w2132] -> w2004
          tunnel: [w2103 w2120] -> w2003
          tunnel: [w2102 w2115] -> w2002
          tunnel: w1999 -> [_ w2112]
          frame False {
          }
          frame True {
            w2116 = 1
            # "Y1 = Y2 = ID\nY3 = IG"
            # "Number of VAR2 steps is 1."
            # "abs(Ig)"
            # "abs(Id)"
            # "Adjusts graph colors."
            n541 = Absolute Value(x=w2127) -> (abs(x)=w2113:dbl[])
            n542 = Absolute Value(x=w2126) -> (abs(x)=w2114:dbl[])
            n543 = Array Max & Min(array=w2114) -> (max value=w2125:dbl, min value=w2123:dbl)  [unwired: 2 out]
            n544 = Array Max & Min(array=w2113) -> (max value=w2124:dbl, min value=w2122:dbl)  [unwired: 2 out]
            n545 = local write "Id max"(w2125) -> ()
            n546 = local write "Id min"(w2123) -> ()
            n547 = local write "Ig max"(w2124) -> ()
            n548 = local write "Ig min"(w2122) -> ()
            n549 = Insert Into Array(array=w2131, new element=w2113) -> (w2120:dbl[])  [unwired: 1 in]
            n550 = Insert Into Array(array=w2130, new element=w2113) -> (w2115:dbl[])  [unwired: 1 in]
            n551 = Insert Into Array(array=w2129, new element=w2114) -> (w2109:dbl[])  [unwired: 1 in]
            n552 = Insert Into Array(array=w2128, new element=w2114) -> (w2132:dbl[])  [unwired: 1 in]
            n553 = control-ref of="Imax vs time"() -> (w2133:refnum<vi>)
            n554 = call "4155C Config Chart Colours.vi"("Numeric"=w2116, "XY Graph 2"=w2133) -> ()  [unwired: 6 in]
            n555 = call "4155C Split array.vi"("Number of VAR2 steps"=w2116, "Y2 data in"=w2109, "X data in"=w2112, "Y1 data in"=w2109, "Y3 data in"=w2120, "error in (no error)"=w2121) -> ("Array of clusters"=w2134:cluster{"Y data in":dbl[], "X data in":dbl[]}[], "error out"=w2119:errorcluster)  [unwired: 1 in]
            n556 = call "4155C Split array.vi"("Number of VAR2 steps"=w2116, "Y2 data in"=w2109, "X data in"=w2112, "Y1 data in"=w2109, "Y3 data in"=w2115, "error in (no error)"=w2119) -> ("Array of clusters"=w2117:cluster{"Y data in":dbl[], "X data in":dbl[]}[], "error out"=w2118:errorcluster)  [unwired: 1 in]
            n557 = local write "Imax vs time"(w2134) -> ()
            n558 = local write "Imin vs time"(w2117) -> ()
          }
        }
        n559 = call "4155C Split array.vi"("Number of VAR2 steps"=w1990, "Y2 data in"=w1981, "X data in"=w1989, "Y1 data in"=w1981, "Y3 data in"=w2020) -> ("Array of clusters"=w2019:cluster{"Y data in":dbl[], "X data in":dbl[]}[])  [unwired: 2 in, 1 out]
        n560 = call "4155C Config Chart Colours.vi"("Numeric"=w1990, "XY Graph 2"=w2018) -> ()  [unwired: 6 in]
        n561 = local write "I vs time (Bias Stress)"(w2019) -> ()
        n562 = Number To Decimal String(number=w2046) -> (decimal integer string=w2066:string)  [unwired: 1 in]
        n563 = Insert Into Array(array=w1987, new element=w1984) -> (w1982:dbl[])  [unwired: 1 in]
        n564 = Concatenate Strings("(Vg = " ("Substring"), w2068, "V, Vd = " ("Substring"), w2066, "V)" ("Substring")) -> (w2064:string)
        n565 = Insert Into Array(array=dbl[][] [] ("Input Array"), new element=w1988) -> (w2075:dbl[][])  [unwired: 2 in]
        n566 = Insert Into Array(array=w1986, new element=w1983) -> (w1985:dbl[])  [unwired: 1 in]
        n567 = Insert Into Array(array=w2075, new element=w1994) -> (w2074:dbl[][])  [unwired: 2 in]
        n568 = control-ref of="Vp vs time (FPP Bias Stress)"() -> (w1991:refnum<vi>)
        n569 = Insert Into Array(array=w2074, new element=w1995) -> (w2073:dbl[][])  [unwired: 2 in]
        n570 = Insert Into Array(array=w2073, new element=w1984) -> (w2071:dbl[][])  [unwired: 2 in]
        n571 = call "4155C Config Chart Colours.vi"("Numeric"=w1990, "XY Graph 2"=w1991) -> ()  [unwired: 6 in]
        n572 = call "4155C Split array.vi"("Number of VAR2 steps"=w1990, "Y2 data in"=w1982, "X data in"=w1989, "Y1 data in"=w1985, "Y3 data in"=w1982) -> ("Array of clusters"=w1992:cluster{"Y data in":dbl[], "X data in":dbl[]}[])  [unwired: 2 in, 1 out]
        n573 = Array To Spreadsheet String(array=w2048, 3:w2052) -> (spreadsheet string=w2054:string)  [unwired: 1 in]
        n574 = Insert Into Array(array=w2071, new element=w1983) -> (w2045:dbl[][])  [unwired: 2 in]
        n575 = Search and Replace String(replace all?=TRUE ("replace all? (F)"), input string=w2054, search string="VgVd", replace string=w2064) -> (result string=w2050:string)  [unwired: 4 in, 3 out]
        n576 = local write "Vp vs time (FPP Bias Stress)"(w1992) -> ()
        n577 = Spreadsheet String To Array(format string=w2052, spreadsheet string=w2050, array type (2D Dbl)=w2048) -> (array=w2049:string[])  [unwired: 1 in]
        n578 = Transpose 2D Array(2D array=w2045) -> (transposed array=w2070:dbl[][])
        n579 = call <vilib>:"compatOverwrite.vi"("overwrite (F)"=TRUE) -> ("overwrite?"=w2042:T8)
        n580 = Open/Create/Replace File(file path (use dialog)=w2060, error in=w1996, operation (0:open)=w2042) -> (refnum out=w2057:refnum<file>, error out=w2058:errorcluster)  [unwired: 3 in, 1 out]
        n581 = call "4155C Write array to file.vi"("Byte Stream File Refnum"=w2057, "Header"=w2049, "Data Array"=w2070, "error in (no error)"=w2058) -> ("dup refnum"=w2055:refnum<file>, "error out"=w2056:errorcluster)  [unwired: 1 in]
        n582 = Close File(refnum=w2055, error in=w2056) -> (error out=w2043:errorcluster)  [unwired: 1 out]
      }
      frame "resample-fpp" {
        w2153 = 1
        w2208 = string[] ["Time /s", "Id VgVd /A", "Ig VgVd /A", "Vp1 VgVd /V", "Vp2 VgVd /V"] ("Header")
        w2212 = "%d" ("format string")
        # "Y1 = Y2 = ID\nY3 = IG"
        # "Y1 = Vp2\nY2 = Y3 = Vp1"
        # "Add a time offset (elapsed time) to the time axis."
        n583 = Number To Decimal String(number=w2196) -> (decimal integer string=w2246:string)  [unwired: 1 in]
        n584 = Fract/Exp String To Number(string=w2243) -> (number=w2201:dbl[])  [unwired: 3 in, 1 out]
        n585 = Concatenate Strings(w2239, "-resamplefpp-" ("Substring"), w2246, w2197, ".txt" ("Substring")) -> (w2244:string)
        n586 = local read "Time Units"() -> (w2177:u16)
        n587 = local read "Plot sample extrema vs time"() -> (w2175:bool)
        n588 = String To Path(string=w2244) -> (path=w2220:path)
        n589 = Index Array(array=w2201, index=0 ("Index")) -> (element=w2207:dbl)
        n590 = Index Array(array=w2201, index=1 ("Index")) -> (element=w2206:dbl)
        n591 = Number To Decimal String(number=w2207) -> (decimal integer string=w2226:string)  [unwired: 1 in]
        n592 = call "4155C Take Sample FPP.vi"("VISA resource name in"=w2203, "error in (no error)"=w2202, "Emergency Stop"=w2221) -> ("Time"=w2178:dbl[], "Vp1"=w2147:dbl[], "VISA Resource Name out"=w2205:refnum<visa-resource-name>, "Ig"=w2158:dbl[], "Id"=w2157:dbl[], "Vp2"=w2146:dbl[], "error out"=w2160:errorcluster)  [unwired: 10 in]
        n593 = Insert Into Array(array=w2185, new element=w2157) -> (w2144:dbl[])  [unwired: 1 in]
        n594 = case shown="0, Default" w2177 {
          tunnel: [w2287 w2288 w2291] -> w2179
          tunnel: w2178 -> [w2286 w2288 w2290]
          frame 2 {
            n595 = Divide(x=w2286, y=3600.0) -> (x/y=w2287:dbl[])
          }
          frame 0, Default {
          }
          frame 1 {
            n596 = Divide(x=w2290, y=60.0) -> (x/y=w2291:dbl[])
          }
        }
        n597 = Insert Into Array(array=w2186, new element=w2158) -> (w2183:dbl[])  [unwired: 1 in]
        n598 = control-ref of="I vs time (Bias Stress)"() -> (w2181:refnum<vi>)
        n599 = Number To Decimal String(number=w2206) -> (decimal integer string=w2224:string)  [unwired: 1 in]
        n600 = Add(x=w2179, y=w2180) -> (x+y=w2151:dbl[])
        n601 = Insert Into Array(array=w2184, new element=w2151) -> (w2152:dbl[])  [unwired: 1 in]
        n602 = call "4155C Split array.vi"("Number of VAR2 steps"=w2153, "Y2 data in"=w2144, "X data in"=w2152, "Y1 data in"=w2144, "Y3 data in"=w2183) -> ("Array of clusters"=w2182:cluster{"Y data in":dbl[], "X data in":dbl[]}[])  [unwired: 2 in, 1 out]
        n603 = Concatenate Strings("(Vg = " ("Substring"), w2226, "V, Vd = " ("Substring"), w2224, "V)" ("Substring")) -> (w2222:string)
        n604 = call "4155C Config Chart Colours.vi"("Numeric"=w2153, "XY Graph 2"=w2181) -> ()  [unwired: 6 in]
        n605 = local write "I vs time (Bias Stress)"(w2182) -> ()
        n606 = Insert Into Array(array=dbl[][] [] ("Input Array"), new element=w2151) -> (w2233:dbl[][])  [unwired: 2 in]
        n607 = Insert Into Array(array=w2233, new element=w2157) -> (w2232:dbl[][])  [unwired: 2 in]
        n608 = Insert Into Array(array=w2232, new element=w2158) -> (w2231:dbl[][])  [unwired: 2 in]
        n609 = Array To Spreadsheet String(array=w2208, 3:w2212) -> (spreadsheet string=w2214:string)  [unwired: 1 in]
        n610 = Insert Into Array(array=w2231, new element=w2147) -> (w2229:dbl[][])  [unwired: 2 in]
        n611 = Insert Into Array(array=w2150, new element=w2147) -> (w2145:dbl[])  [unwired: 1 in]
        n612 = Search and Replace String(replace all?=TRUE ("replace all? (F)"), input string=w2214, search string="VgVd", replace string=w2222) -> (result string=w2210:string)  [unwired: 4 in, 3 out]
        n613 = Insert Into Array(array=w2229, new element=w2146) -> (w2200:dbl[][])  [unwired: 2 in]
        n614 = Insert Into Array(array=w2149, new element=w2146) -> (w2148:dbl[])  [unwired: 1 in]
        n615 = Spreadsheet String To Array(format string=w2212, spreadsheet string=w2210, array type (2D Dbl)=w2208) -> (array=w2209:string[])  [unwired: 1 in]
        n616 = control-ref of="Vp vs time (FPP Bias Stress)"() -> (w2154:refnum<vi>)
        n617 = local read "Plot sample extrema vs time"() -> (w2162:bool)
        n618 = call <vilib>:"compatOverwrite.vi"("overwrite (F)"=TRUE) -> ("overwrite?"=w2199:T8)
        n619 = Transpose 2D Array(2D array=w2200) -> (transposed array=w2228:dbl[][])
        n620 = call "4155C Config Chart Colours.vi"("Numeric"=w2153, "XY Graph 2"=w2154) -> ()  [unwired: 6 in]
        n621 = call "4155C Split array.vi"("Number of VAR2 steps"=w2153, "Y2 data in"=w2145, "X data in"=w2152, "Y1 data in"=w2148, "Y3 data in"=w2145) -> ("Array of clusters"=w2155:cluster{"Y data in":dbl[], "X data in":dbl[]}[])  [unwired: 2 in, 1 out]
        n622 = case shown="True" w2162 {
          tunnel: w2163 -> [w2248 w2250]
          tunnel: [w2248 w2251] -> w2161
          tunnel: w2151 -> [_ w2249]
          frame False {
          }
          frame True {
            n623 = Insert Into Array(array=w2250, new element=w2249) -> (w2251:i32[])  [unwired: 1 in]
          }
        }
        n624 = case shown="True" w2175 {
          tunnel: w2157 -> [_ w2276]
          tunnel: w2158 -> [_ w2277]
          tunnel: [w2258 w2268] -> w2159
          tunnel: w2160 -> [w2258 w2271]
          tunnel: w2176 -> [w2257 w2261]
          tunnel: w2173 -> [w2256 w2260]
          tunnel: w2172 -> [w2255 w2279]
          tunnel: w2171 -> [w2254 w2278]
          tunnel: w2170 -> [w2253 w2281]
          tunnel: w2169 -> [w2252 w2280]
          tunnel: [w2257 w2261] -> w2174
          tunnel: [w2256 w2260] -> w2164
          tunnel: [w2255 w2259] -> w2166
          tunnel: [w2254 w2282] -> w2165
          tunnel: [w2253 w2270] -> w2168
          tunnel: [w2252 w2265] -> w2167
          tunnel: w2161 -> [_ w2262]
          frame False {
          }
          frame True {
            w2266 = 1
            # "Y1 = Y2 = ID\nY3 = IG"
            # "Number of VAR2 steps is 1."
            # "abs(Ig)"
            # "abs(Id)"
            # "Adjusts graph colors."
            n625 = Absolute Value(x=w2277) -> (abs(x)=w2263:dbl[])
            n626 = Absolute Value(x=w2276) -> (abs(x)=w2264:dbl[])
            n627 = Array Max & Min(array=w2264) -> (max value=w2275:dbl, min value=w2273:dbl)  [unwired: 2 out]
            n628 = Array Max & Min(array=w2263) -> (max value=w2274:dbl, min value=w2272:dbl)  [unwired: 2 out]
            n629 = local write "Id max"(w2275) -> ()
            n630 = local write "Id min"(w2273) -> ()
            n631 = local write "Ig max"(w2274) -> ()
            n632 = local write "Ig min"(w2272) -> ()
            n633 = Insert Into Array(array=w2281, new element=w2263) -> (w2270:dbl[])  [unwired: 1 in]
            n634 = Insert Into Array(array=w2280, new element=w2263) -> (w2265:dbl[])  [unwired: 1 in]
            n635 = Insert Into Array(array=w2279, new element=w2264) -> (w2259:dbl[])  [unwired: 1 in]
            n636 = Insert Into Array(array=w2278, new element=w2264) -> (w2282:dbl[])  [unwired: 1 in]
            n637 = control-ref of="Imax vs time"() -> (w2283:refnum<vi>)
            n638 = call "4155C Config Chart Colours.vi"("Numeric"=w2266, "XY Graph 2"=w2283) -> ()  [unwired: 6 in]
            n639 = call "4155C Split array.vi"("Number of VAR2 steps"=w2266, "Y2 data in"=w2259, "X data in"=w2262, "Y1 data in"=w2259, "Y3 data in"=w2270, "error in (no error)"=w2271) -> ("Array of clusters"=w2284:cluster{"Y data in":dbl[], "X data in":dbl[]}[], "error out"=w2269:errorcluster)  [unwired: 1 in]
            n640 = call "4155C Split array.vi"("Number of VAR2 steps"=w2266, "Y2 data in"=w2259, "X data in"=w2262, "Y1 data in"=w2259, "Y3 data in"=w2265, "error in (no error)"=w2269) -> ("Array of clusters"=w2267:cluster{"Y data in":dbl[], "X data in":dbl[]}[], "error out"=w2268:errorcluster)  [unwired: 1 in]
            n641 = local write "Imax vs time"(w2284) -> ()
            n642 = local write "Imin vs time"(w2267) -> ()
          }
        }
        n643 = Open/Create/Replace File(file path (use dialog)=w2220, error in=w2159, operation (0:open)=w2199) -> (refnum out=w2217:refnum<file>, error out=w2218:errorcluster)  [unwired: 3 in, 1 out]
        n644 = call "4155C Write array to file.vi"("Byte Stream File Refnum"=w2217, "Header"=w2209, "Data Array"=w2228, "error in (no error)"=w2218) -> ("dup refnum"=w2215:refnum<file>, "error out"=w2216:errorcluster)  [unwired: 1 in]
        n645 = local write "Vp vs time (FPP Bias Stress)"(w2155) -> ()
        n646 = Close File(refnum=w2215, error in=w2216) -> (error out=w2204:errorcluster)  [unwired: 1 out]
      }
      frame "serial" {
        n647 = local read "Termination char\n(0xA = '\\n' = LF)\n(0xD = '\\r' = CR)"() -> (w2321:u8)
        n648 = local read "Enable Termination\nChar (T)"() -> (w2322:bool)
        n649 = Index Array(array=w2329, index=0 ("Index")) -> (element=w2328:string)
        n650 = local read "parity"() -> (w2312:u16)
        n651 = local read "Delay before read (ms)"() -> (w2323:u32)
        n652 = local read "byte count"() -> (w2320:u32)
        n653 = local read "VISA resource name"() -> (w2316:refnum<visa-resource-name>)
        n654 = local read "baud rate"() -> (w2315:u32)
        n655 = local read "Serial End Mode for Reads"() -> (w2314:u16)
        n656 = local read "Timeout (ms)"() -> (w2319:u32)
        n657 = local read "data bits"() -> (w2313:u16)
        n658 = local read "stop bits"() -> (w2318:u16)
        n659 = local read "flow control"() -> (w2317:u16)
        n660 = call "Serial write and read v0.5.vi"("Delay before read (ms)"=w2323, "Termination char\n(0xA = '\\n' = LF)\n(0xD = '\\r' = CR)"=w2321, "Enable Termination\nChar (T)"=w2322, "parity"=w2312, "stop bits"=w2318, "string to write"=w2328, "flow control"=w2317, "byte count"=w2320, "Serial Settings:Serial End Mode for Reads"=w2314, "Timeout (ms)"=w2319, "error in (no error)"=w2334, "VISA resource name"=w2316, "baud rate"=w2315, "data bits"=w2313) -> ("Serial port output"=w2324:string, "error out"=w2333:errorcluster)
        n661 = Build Array (concatenate)(w2324, w2325) -> (w2326:string[])
      }
    }
    "Probe 4 Indicator" <- w70
    "Timings Indicator" <- w71
    n662 = local read "Time Units"() -> (w104:u16)
    n663 = case shown="0" w104 {
      tunnel: ["Time (Seconds)" ("element") "Time (Minutes)" ("element") "Time (Hours)" ("element")] -> w73
      frame 0 {
      }
      frame 1, Default {
      }
      frame 2 {
      }
    }
    n664 = Build Array(w153, w110, w120, w119, w118, w117, w116, w115, w114, w113, w112, w111, w109) -> (w174:dbl[][])
    n665 = Transpose 2D Array(2D array=w174) -> (transposed array=w173:dbl[][])
    n666 = Concatenate Strings(w79, "-I-vs-time.txt" ("Suffix (Imax,Imin,Ion,Ioff)")) -> (w184:string)
    n667 = Build Array(w73, "Is max (A)" ("VAR2 Name"), "Is min (A)" ("VAR2 Name"), "Id max (A)" ("VAR2 Name"), "Id min (A)" ("VAR2 Name"), "Ig max (A)" ("VAR2 Name"), "Ig min (A)" ("VAR2 Name"), "Is on (A)" ("VAR2 Name"), "Is off (A)" ("VAR2 Name"), "Id on (A)" ("VAR2 Name"), "Id off (A)" ("VAR2 Name"), "Ig on (A)" ("VAR2 Name"), "Ig off (A)" ("VAR2 Name")) -> (w179:string[])
    n668 = Array To Spreadsheet String(array=w173, 3:"%e" ("format string")) -> (spreadsheet string=w177:string)  [unwired: 1 in]
    n669 = Array To Spreadsheet String(array=w179, 3:"" ("format string")) -> (spreadsheet string=w178:string)  [unwired: 1 in]
    n670 = String To Path(string=w184) -> (path=w183:path)
    n671 = Build Array(w178, w177) -> (w176:string[])
    n672 = Write to Text File(file (use dialog)=w183, text=w176, error in=w152) -> (refnum out=w185:refnum<file>, error out=w175:errorcluster)  [unwired: 1 in, 1 out]
    n673 = Close File(refnum=w185, error in=w175) -> (error out=w107:errorcluster)  [unwired: 1 out]
    n674 = Concatenate Strings(w79, "-serial-port.txt" ("Suffix (serial port log)")) -> (w155:string)
    n675 = String To Path(string=w155) -> (path=w154:path)
    n676 = Build Array(w73, "Serial port input" ("VAR2 Name"), "Serial port output: ") -> (w145:string[])
    n677 = Array To Spreadsheet String(array=w149, 3:"" ("format string")) -> (spreadsheet string=w142:string)  [unwired: 1 in]
    n678 = Array To Spreadsheet String(array=w145, 3:"" ("format string")) -> (spreadsheet string=w143:string)  [unwired: 1 in]
    n679 = Build Array(w143, w142) -> (w144:string[])
    n680 = Array To Spreadsheet String(array=w148, 3:"" ("format string")) -> (spreadsheet string=w160:string)  [unwired: 1 in]
    n681 = Write to Text File(file (use dialog)=w154, text=w144, error in=w107) -> (refnum out=w156:refnum<file>, error out=w157:errorcluster)  [unwired: 1 in, 1 out]
    n682 = Close File(refnum=w156, error in=w157) -> (error out=w80:errorcluster)  [unwired: 1 out]
    n683 = local write "Serial port data"(w160) -> ()
    n684 = Build Array(w78, w77, w76, w75) -> (w89:dbl[][])
    n685 = Build Array(w73, "Is (A)" ("VAR2 Name"), "Id (A)" ("VAR2 Name"), "Ig (A)" ("VAR2 Name")) -> (w85:string[])
    n686 = Transpose 2D Array(2D array=w89) -> (transposed array=w88:dbl[][])
    n687 = Concatenate Strings(w79, "-sample.txt" ("Suffix (Imax,Imin,Ion,Ioff)")) -> (w95:string)
    n688 = Array To Spreadsheet String(array=w85, 3:"" ("format string")) -> (spreadsheet string=w84:string)  [unwired: 1 in]
    n689 = Array To Spreadsheet String(array=w88, 3:"%e" ("format string")) -> (spreadsheet string=w92:string)  [unwired: 1 in]
    n690 = String To Path(string=w95) -> (path=w94:path)
    n691 = Build Array(w84, w92) -> (w91:string[])
    n692 = Write to Text File(file (use dialog)=w94, text=w91, error in=w80) -> (refnum out=w96:refnum<file>, error out=w90:errorcluster)  [unwired: 1 in, 1 out]
    n693 = Close File(refnum=w96, error in=w90) -> (error out=w72:errorcluster)  [unwired: 1 out]
    "error out" <- w72
  }
  "Is max" <- w13
  "Id max" <- w13
  "Ig max" <- w13
  "Imax vs time" <- w2
  "I vs Vg" <- w2
  "Imin vs time" <- w2
  "I vs Vd" <- w2
  "Serial port data" <- "" ("Serial port data")
  "Is min" <- w12
  "Id min" <- w12
  "Ig min" <- w12
  "Ion vs time" <- w2
  "Ioff vs time" <- w2
  "Is on" <- w11
  "Id on" <- w11
  "Ig on" <- w11
  "Is off" <- w10
  "Id off" <- w10
  "Ig off" <- w10
  "I vs time (Bias Stress)" <- w2
  "Vp1" <- w3
  "Vp2" <- w3
  "Vp vs time (FPP Bias Stress)" <- w2
  "Vp vs Vg (FPP)" <- w2
  "Vdg vs time (Bias Stress)" <- w2
